vi "Autonomous Independent.vi"   [LabVIEW 2015]
doc: "This VI is called when autonomous begins, and will automatically be terminated when autonomous ends. You can carry out timed or sensor driven robot movement independently without needing to return to the caller."
uses:
  Robot Global Data.vi
  <vilib>/addons/control/pid/pid.llb/PID (DBL).vi
  navX Library v2/navX Library v2.lvlib
  <vilib>/addons/control/pid/NI_PID_pid.lvlib
panel:
  # "1 - Low Bar (Far Left)\n5 - Far Right"
  # "0 - Porticullis\n1 - Shovel the Fries\n2 - Low Bar\n3 - Rock Wall\n4 - Rough Terrain\n5\n6\n7"
types:
  T1 = typedef "navX Library v2.lvlib/Z900_navX_DeviceTypeDef.ctl" = cluster{"Interface":cluster{"Protocol":T2, "Update Rate (4Hz-60Hz)":u8, "navX Open TypeDef":variant}, "Notify Packet":refnum<notifier>, "Loop VI Refnum":refnum<vi>, "Ready to Close Occurrence Refnum":refnum<k4>}
  T2 = typedef "navX Library v2.lvlib/Z900_navX_ProtocolTypeDef.ctl" = enum16{"SERIAL", "I2C", "SPI"}
  T3 = typedef "WPI_EncoderDevRef.ctl" = cluster{"DevStatus":errorcluster, "EncoderIndex":T4, "CounterIndex":T5, "DistancePerCount":dbl, "Decoding Type":T6}
  T4 = typedef "FPGA_EncoderIdx.ctl" = enum8{"Enc 0", "Enc 1", "Enc 2", "Enc 3", "Enc 4", "Enc 5", "Enc 6", "Enc 7", "Invalid"}
  T5 = typedef "FPGA_CounterCtrSystemIndex.ctl" = enum8{"Ctr 0", "Ctr 1", "Ctr 2", "Ctr 3", "Ctr 4", "Ctr 5", "Ctr 6", "Ctr 7", "Invalid"}
  T6 = typedef "WPI_EncoderType.ctl" = enum16{"1x", "2x", "4x"}
  T7 = cluster{"proportional gain (Kc)":dbl, "integral time (Ti, min)":dbl, "derivative time (Td, min)":dbl}
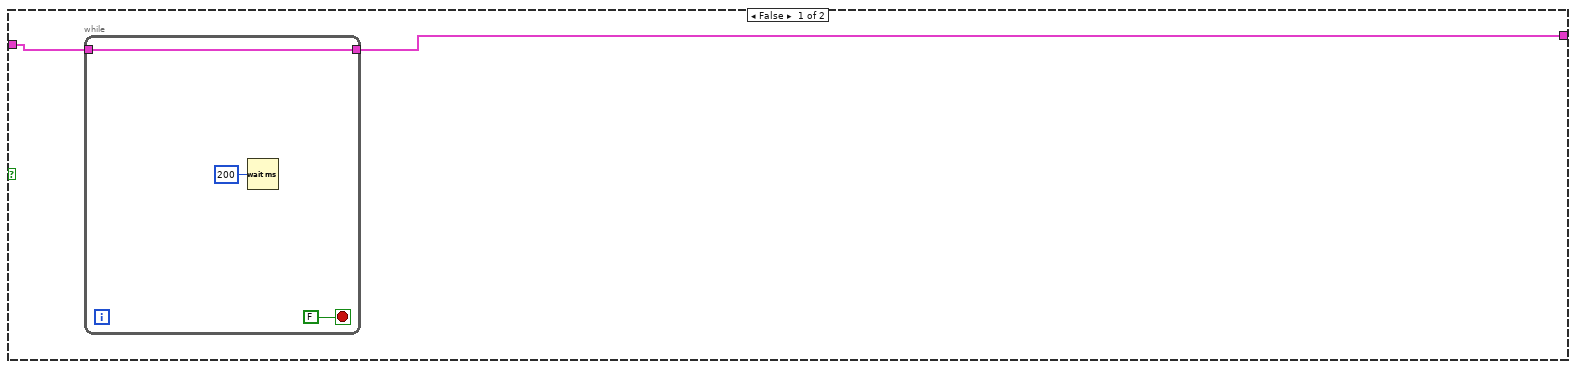
[diagram p2: hidden frame]
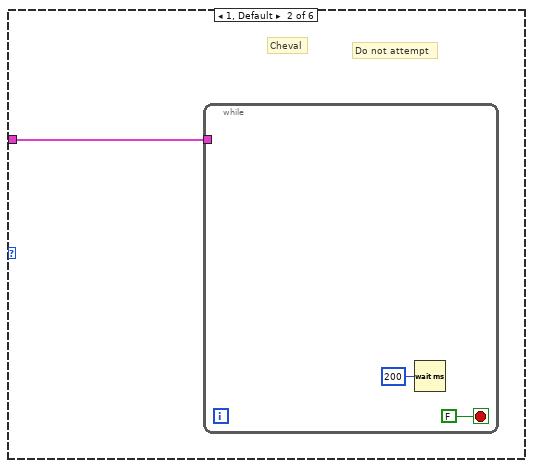
[diagram p3: hidden frame]
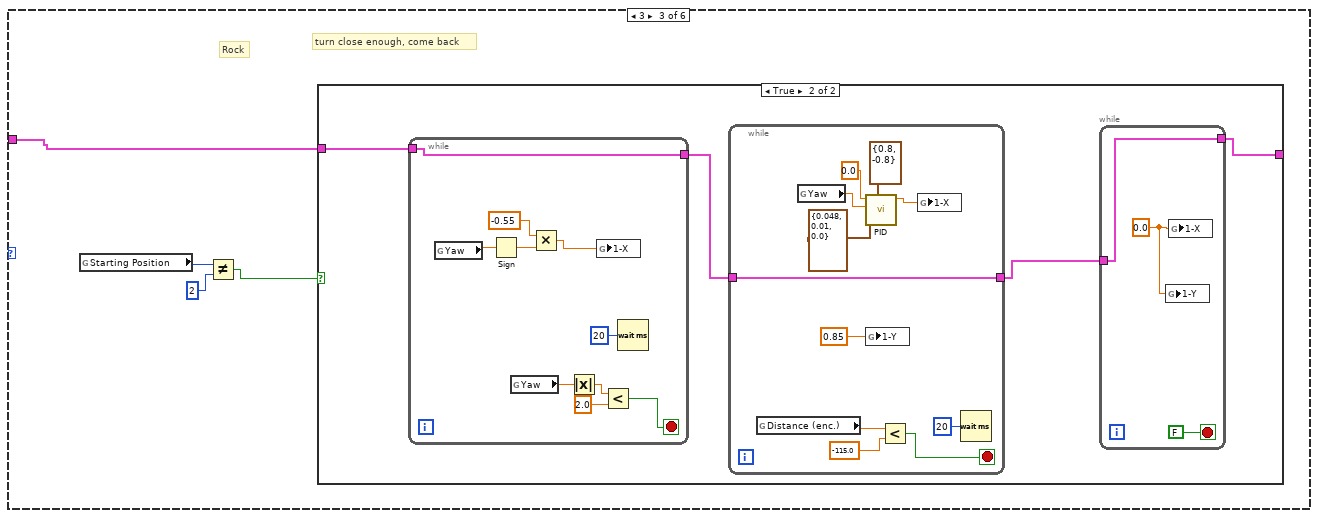
[diagram p4: hidden frame]
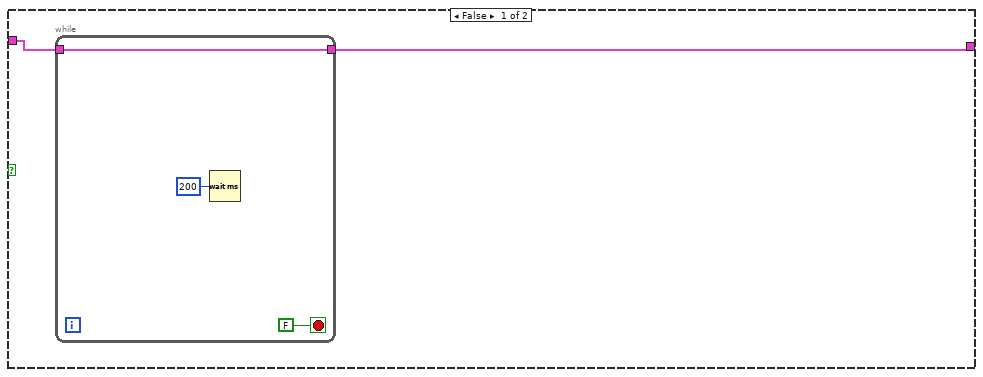
[diagram p5: hidden frame]
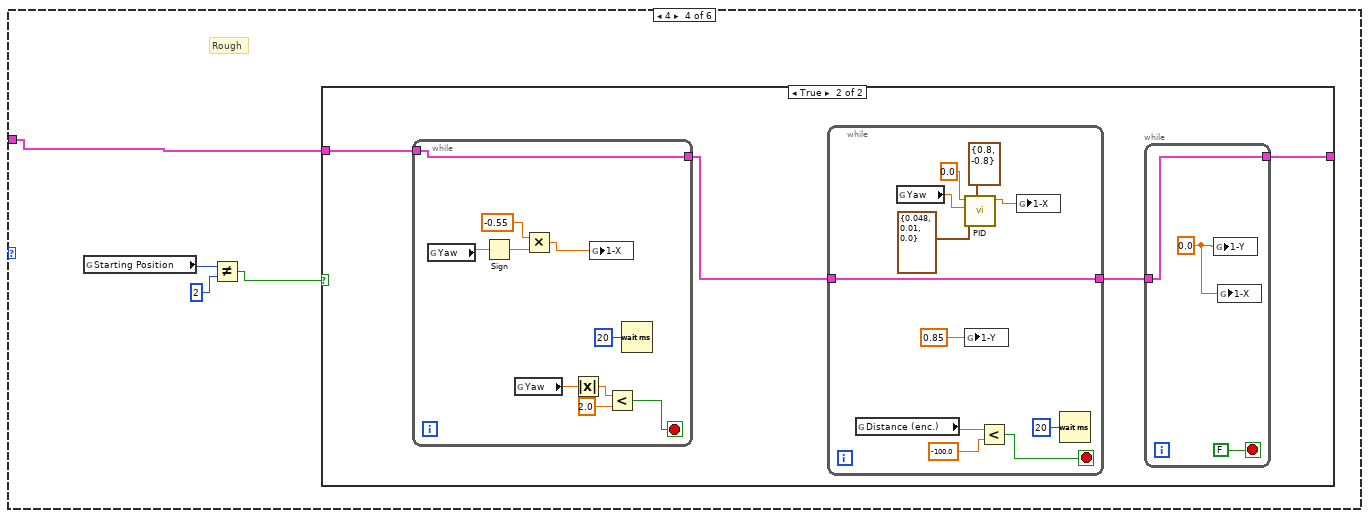
[diagram p6: hidden frame]
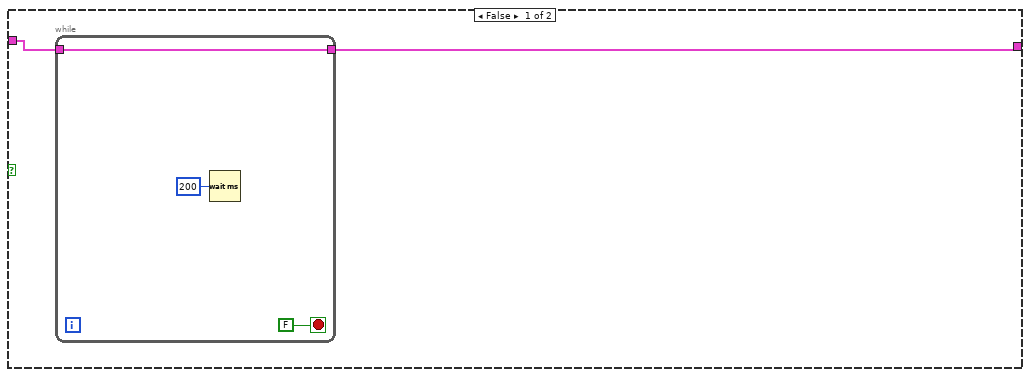
[diagram p7: hidden frame]
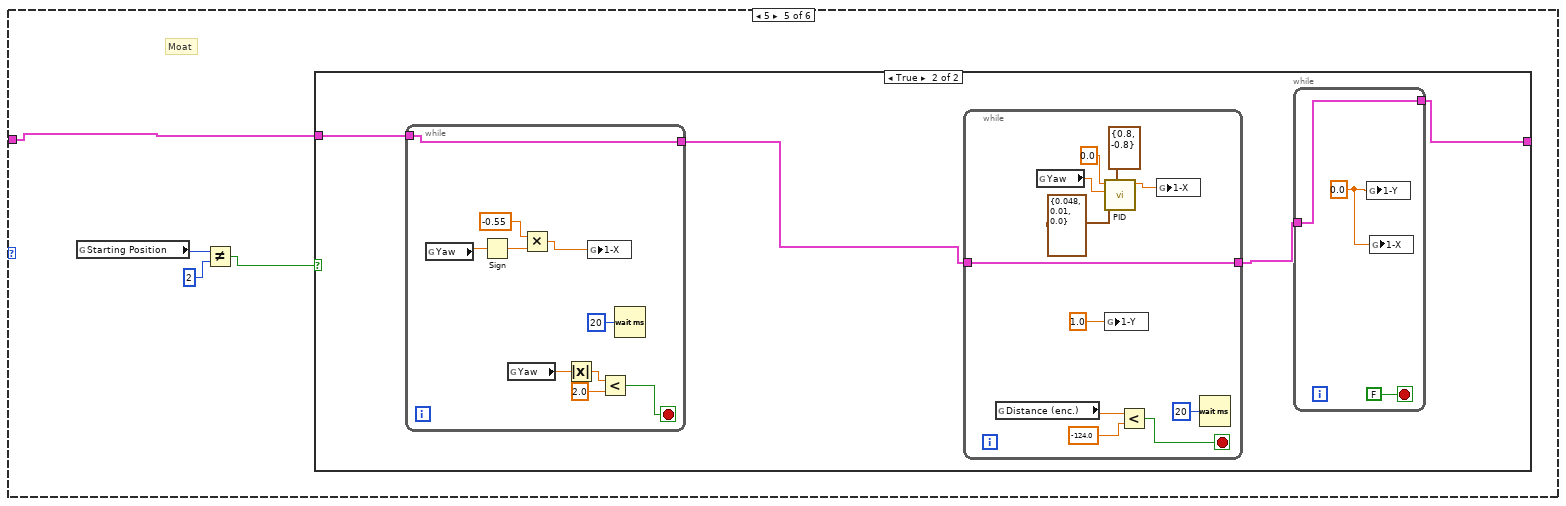
[diagram p8: hidden frame]
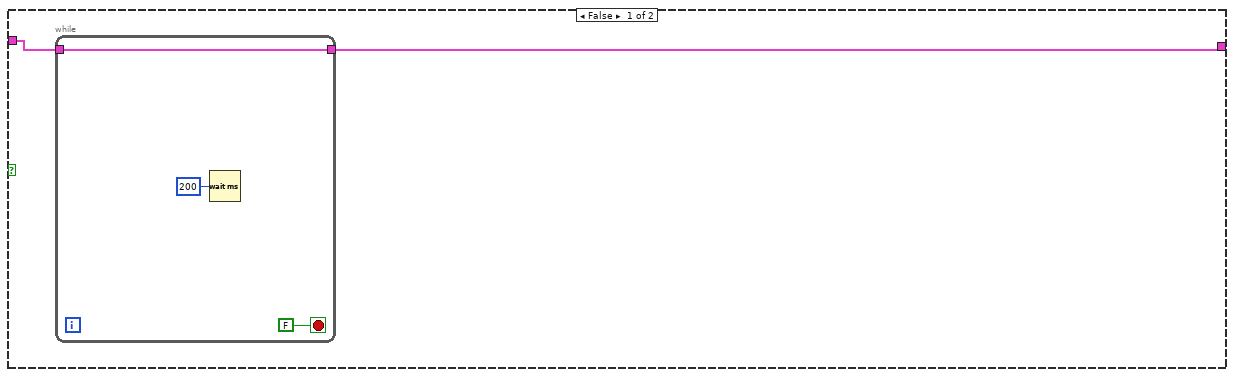
[diagram p9: hidden frame]
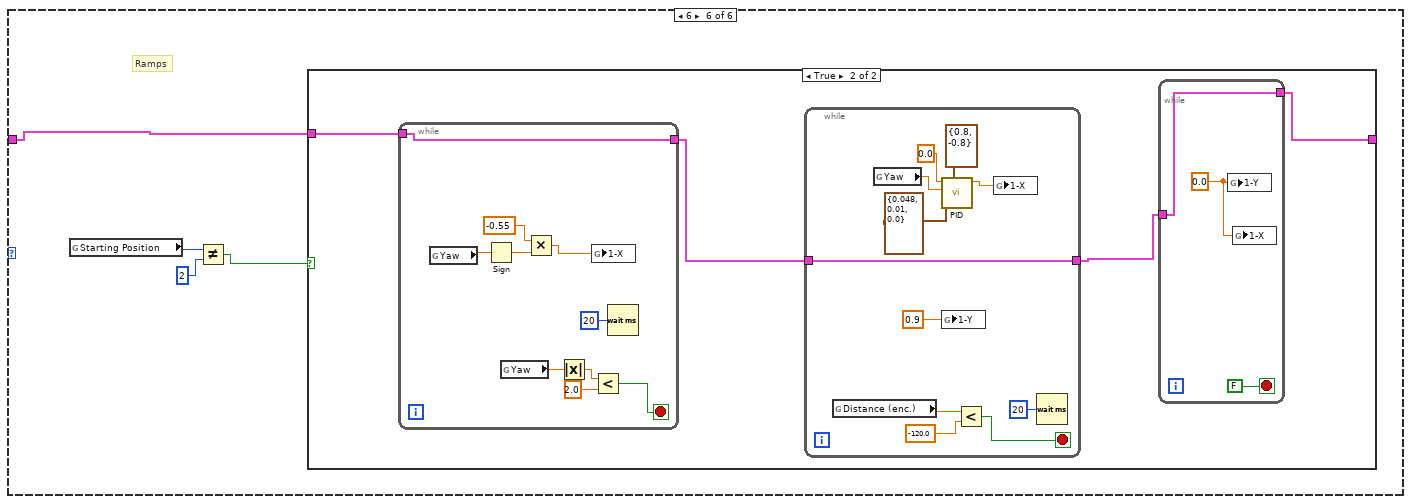
[diagram p10: hidden frame]
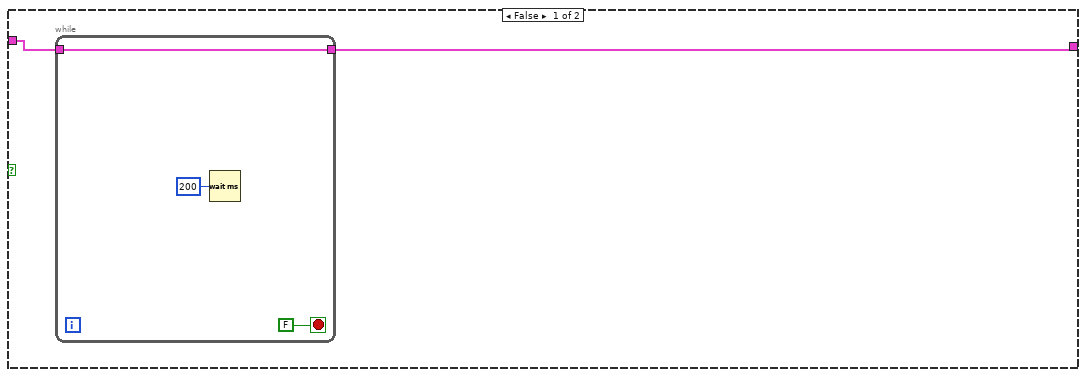
[diagram p11: hidden frame]
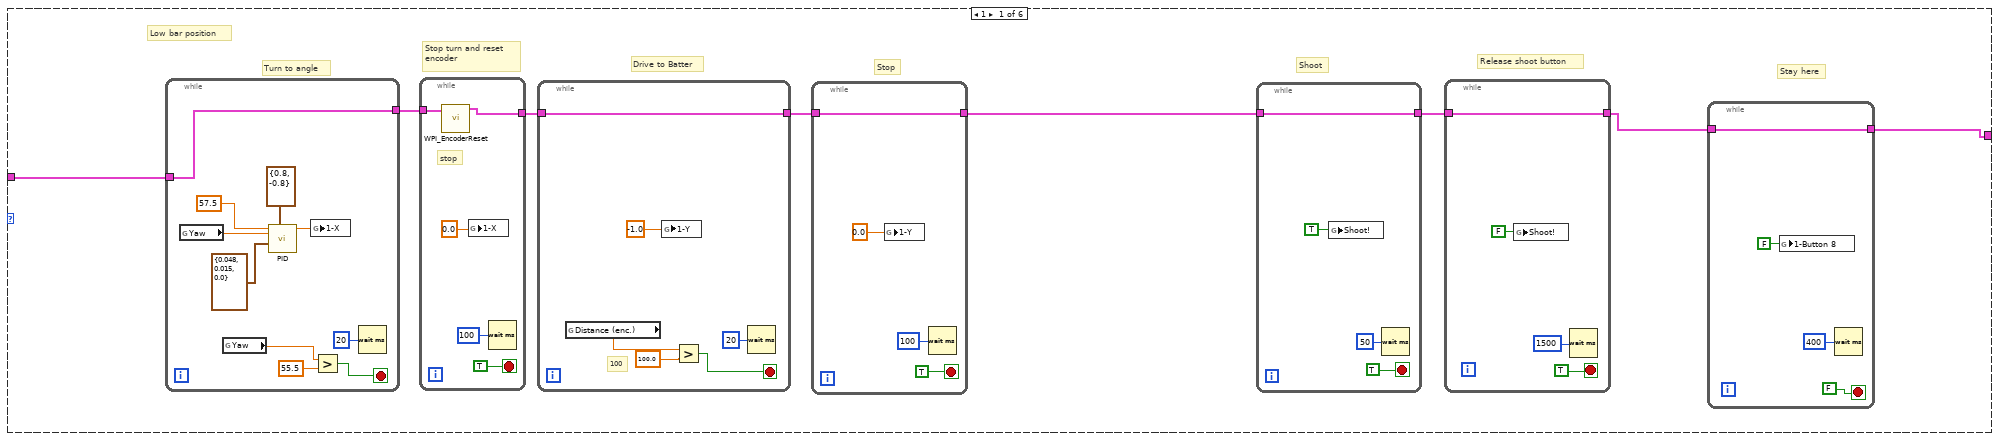
[diagram p12: hidden frame]
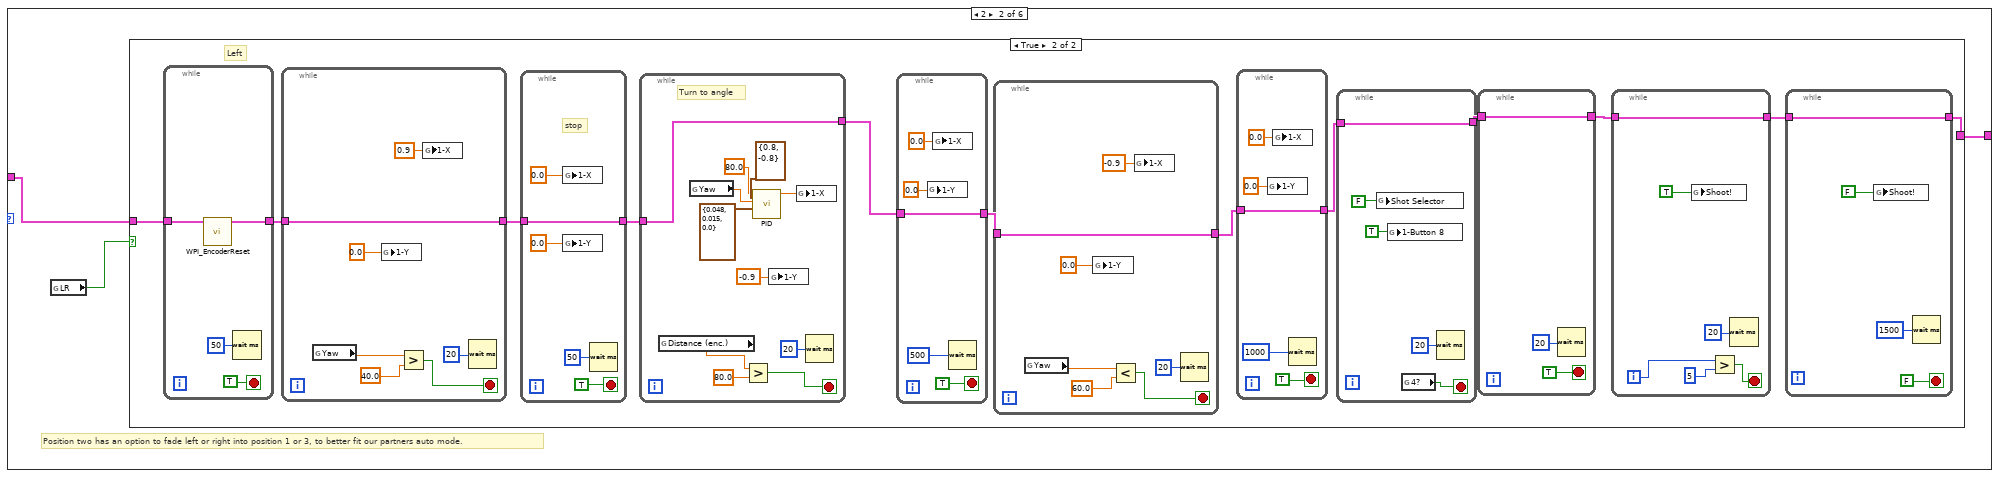
[diagram p13: hidden frame]
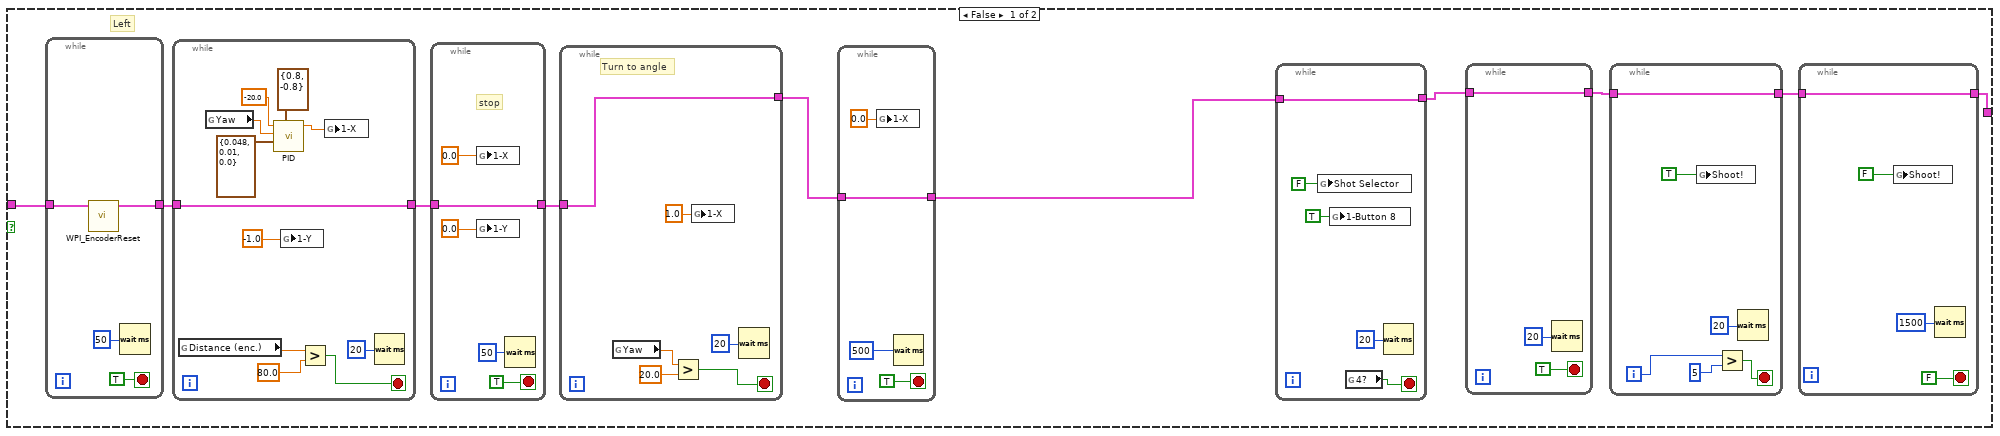
[diagram p14: hidden frame]
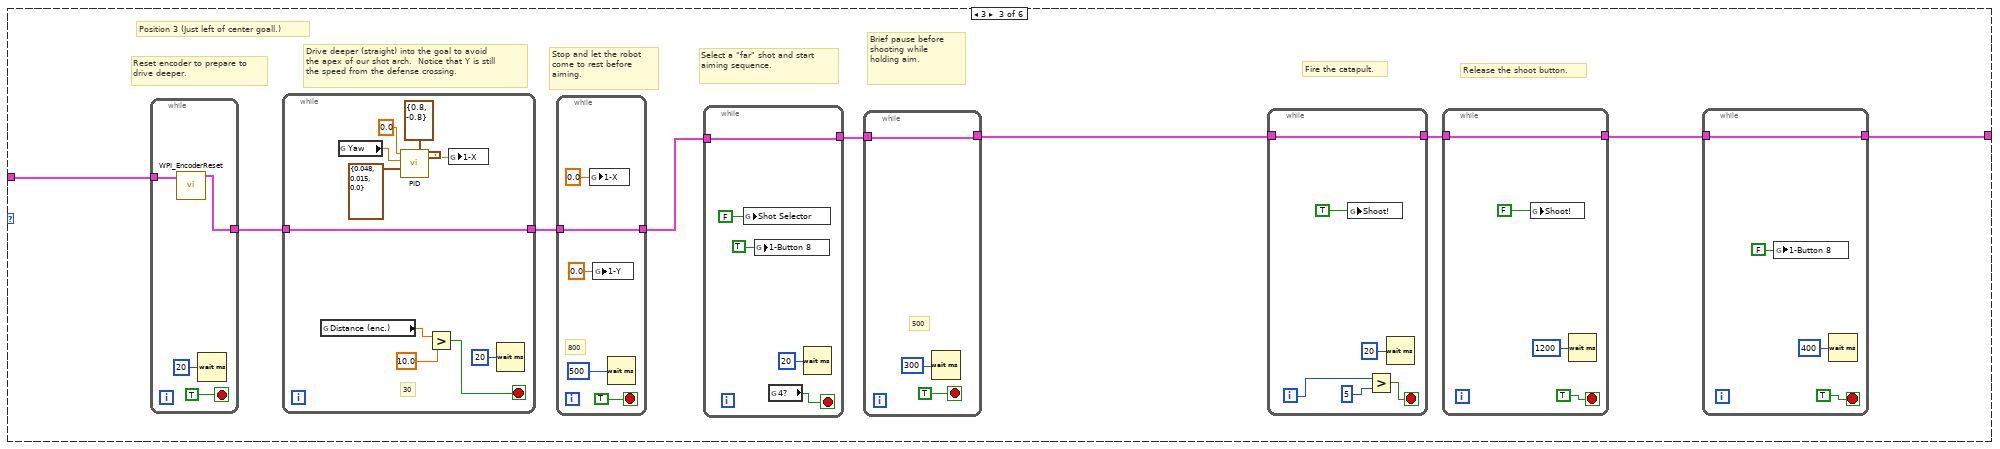
[diagram p15: hidden frame]
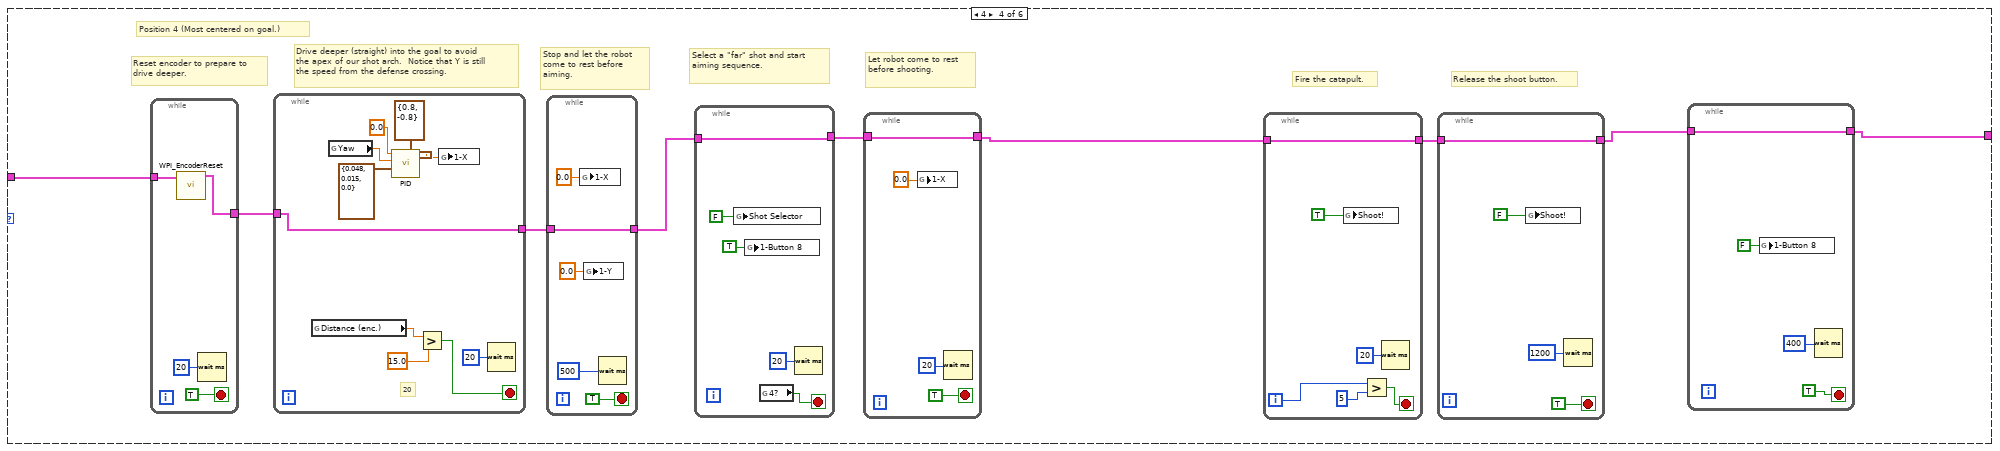
[diagram p16: hidden frame]
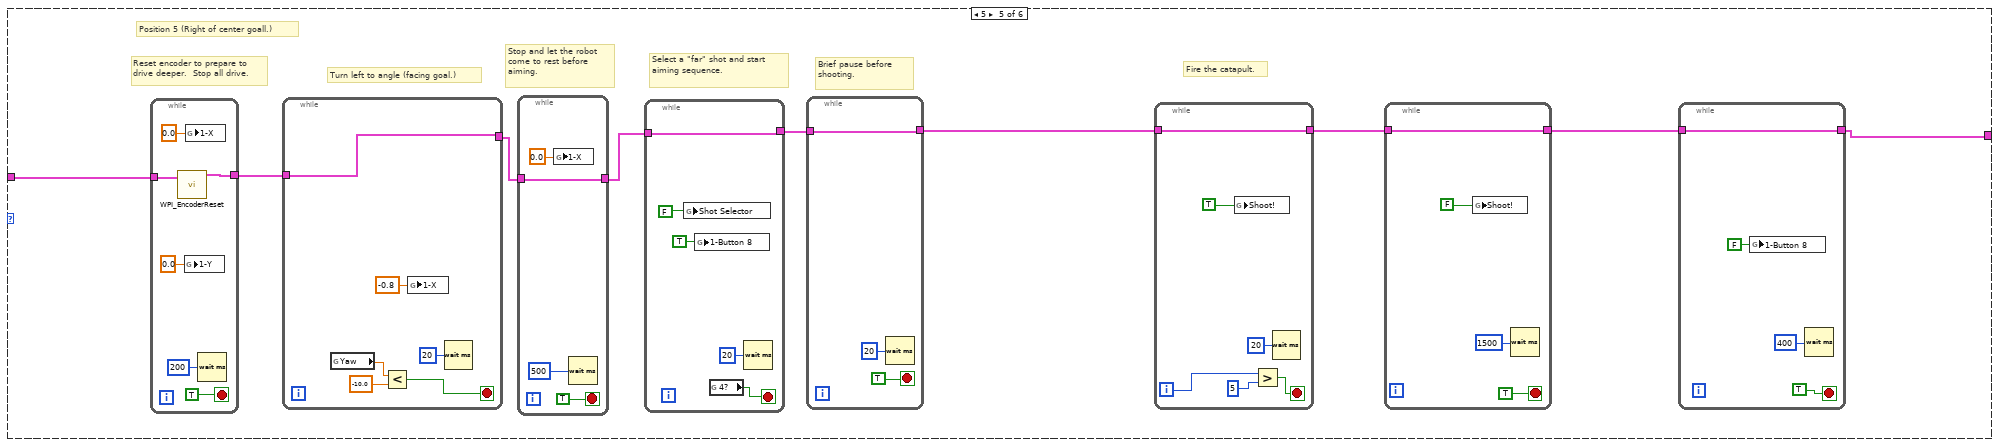
[diagram p17: hidden frame]
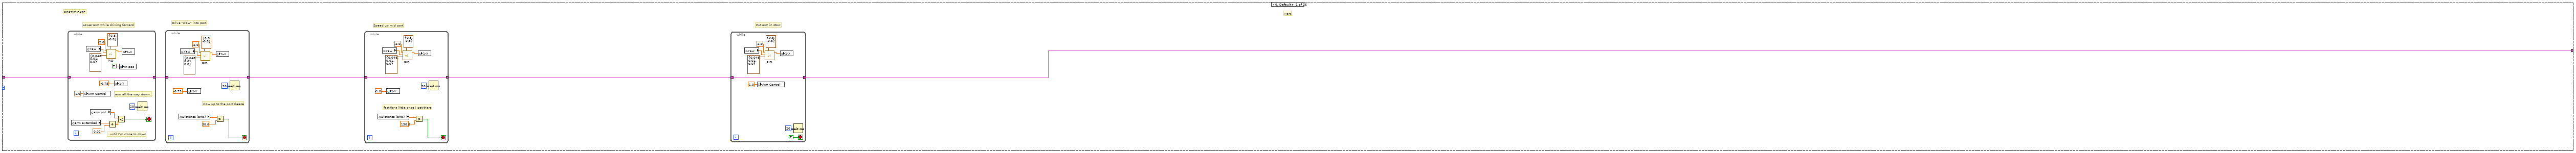
[diagram p18: hidden frame]
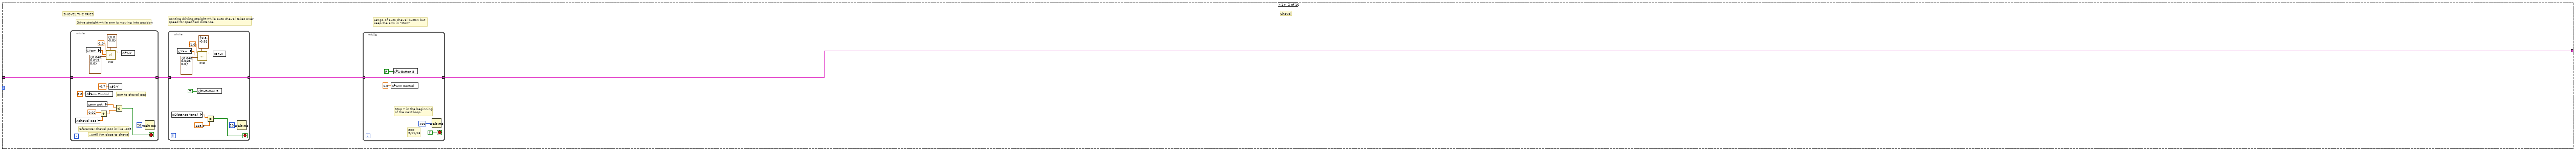
[diagram p19: hidden frame]
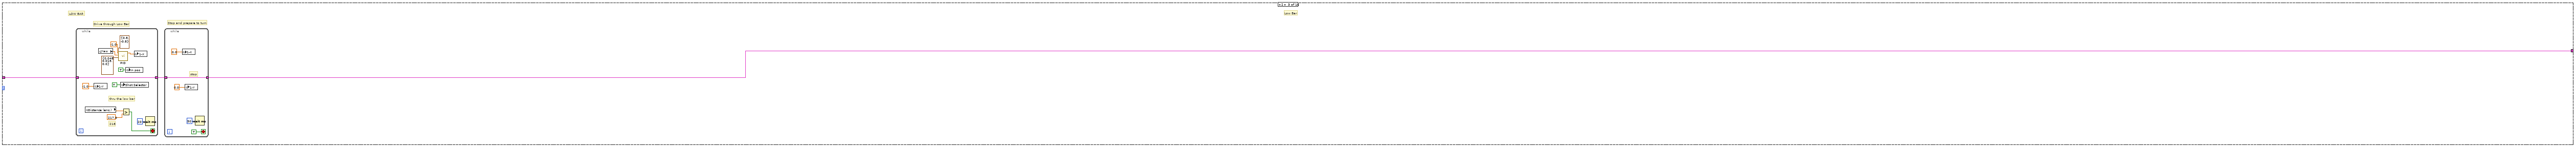
[diagram p20: hidden frame]
diagram:
  # "Our auto philosophy is to write the driver inputs to global variables, and the code for both modes is in periodic tasks"
  # "If the defense is not Cheval\nand the position is not 2\n(bc of wierd fade in 2),\nreturn to the neutral zone"
  # "GUIDE TO THESE AUTOS:\nThree loops are present. \nThe first is generally the \"cross defense\" loop, with the selector being which defense is to be crossed\nThe second is \"shoot the ball\".  The selector is what position - defense pos 5 and 2 in particular are different from the rest.\nThe third is \"return to neutral zone\". Specific to each defense\n\nTwo ball is entirely in the first loop"
  # "Last year we once had a problem.\nWe saved as default a hard left turn on the\njoystick. When we started auto we crashed into\nthe wall. We went overboard to make sure that's\nfixed this year. Reset EVERYTHING"
  # "Forces low bar to be low bar!"
  # "Every 20ms, report that we are running autonomous\ncode. Loop will abort the same time as the VI."
  # "This tells you the driver position\nand alliance color"
  n1 = while {
    stop <- FALSE stop-if-true
    n2 = call <vilib>:"WPI_DriverStationReport Robot Code State.vi"("Autonomous"=TRUE) -> ()  [unwired: 10 in, 1 out]
    n3 = Wait (ms)(milliseconds to wait=u32 20) -> ()  [unwired: 1 out]
  }
  n4 = call <vilib>:"WPI_DriverStationGet Alliance Info.vi"() -> ()  [unwired: 12 out]
  n5 = call "Z900_navX_RefNum_Get.vi"("refnum name"="NavX") -> ("navX Device"=w1:T1)  [unwired: 9 in, 1 out]
  n6 = call <vilib>:"WPI_EncoderRefNum Registry Get.vi"("refnum name"="encoder") -> ("EncoderDevRef"=w15:T3)  [unwired: 9 in, 1 out]
  n7 = while {
    tunnel: w15 -> [w40]
    tunnel: [w39] -> w13
    tunnel: w1 -> [w24]
    stop <- TRUE stop-if-true
    # "500"
    n8 = global read "Robot Global Data.vi" "CamTargetMem"() -> (w19:dbl)
    n9 = global write "Robot Global Data.vi" "In pos"(FALSE ("In pos")) -> ()
    n10 = global write "Robot Global Data.vi" "arm override"(FALSE ("In pos")) -> ()
    n11 = global write "Robot Global Data.vi" "1-X"(0.0 ("1-X")) -> ()
    n12 = global write "Robot Global Data.vi" "1-Y"(0.0 ("1-X")) -> ()
    n13 = call "Z900_navX_Set_ZeroYaw.vi"("navX Device"=w24) -> ()  [unwired: 9 in, 2 out]
    n14 = global write "Robot Global Data.vi" "1-Trigger"(FALSE ("In pos")) -> ()
    n15 = global write "Robot Global Data.vi" "retainer num"(i16 2 ("retainer num")) -> ()
    n16 = global write "Robot Global Data.vi" "in ctl num"(i16 0 ("retainer num")) -> ()
    n17 = global write "Robot Global Data.vi" "Shoot!"(FALSE ("In pos")) -> ()
    n18 = global write "Robot Global Data.vi" "Shot Selector"(FALSE ("In pos")) -> ()
    n19 = global write "Robot Global Data.vi" "Arm Control"(1.0 ("retainer num")) -> ()
    n20 = global write "Robot Global Data.vi" "climb num"(0 ("retainer num")) -> ()
    n21 = global write "Robot Global Data.vi" "left num"(i8 0 ("retainer num")) -> ()
    n22 = global write "Robot Global Data.vi" "right num"(i8 0 ("retainer num")) -> ()
    n23 = global write "Robot Global Data.vi" "1-Button 5"(FALSE ("In pos")) -> ()
    n24 = global write "Robot Global Data.vi" "1-TopLeft"(FALSE ("In pos")) -> ()
    n25 = call <vilib>:"WPI_EncoderReset.vi"("EncoderDevRef"=w40) -> ("EncoderDevRef"=w39:T3)  [unwired: 9 in, 1 out]
    n26 = global write "Robot Global Data.vi" "Pins / Intake timing"(550.0 ("Pins / Intake timing")) -> ()
    n27 = global write "Robot Global Data.vi" "CamTargetReal"(w19) -> ()
    n28 = global write "Robot Global Data.vi" "Slew"(0.2 ("PTO speed")) -> ()
    n29 = Wait (ms)(milliseconds to wait=u32 50) -> ()  [unwired: 1 out]
  }
  n30 = global read "Robot Global Data.vi" "Defense to Cross"() -> (w12:i32)
  n31 = case shown="8" w12 {
    tunnel: w13 -> [w46 w96 w129 w149 w162 w175 w188 w212 w311 w604 w625 w823 w1043 w1309 w1568 w1848]
    tunnel: [w42 w93 w128 w148 w161 w174 w187 w200 w313 w603 w627 w825 w1045 w1311 w1570 w1850] -> w3
    frame 0, Default {
      # "Port"
      # "Put arm in stow"
      # "Speed up mid port"
      # "Drive \"slow\" into port."
      # "Lower arm while driving forward"
      # "PORTICLEASE"
      n32 = while {
        tunnel: w46 -> [w86]
        tunnel: [w86] -> w45
        stop <- w87 stop-if-true
        # "..until I'm close to down"
        # "arm all the way down..."
        n33 = global read "Robot Global Data.vi" "arm extended"() -> (w89:dbl)
        n34 = global write "Robot Global Data.vi" "Arm Control"(-1.0 ("retainer num")) -> ()
        n35 = global read "Robot Global Data.vi" "Yaw"() -> (w79:dbl)
        n36 = global read "Robot Global Data.vi" "arm pot"() -> (w91:dbl)
        n37 = call-poly <vilib>:"PID.vi"("output range"=cluster{"output high":dbl, "output low":dbl} {"output high"=0.8, "output low"=-0.8} ("output range 2"), "PID gains"=T7 {"proportional gain (Kc)"=0.048, "integral time (Ti, min)"=0.01, "derivative time (Td, min)"=0.0} ("PID gains 2"), "process variable"=w79, "setpoint"=-2.0) -> ("output"=w81:dbl)  [unwired: 6 in, 1 out]
        n38 = Add(x=w89, y=0.02) -> (x+y=w90:dbl)
        n39 = global write "Robot Global Data.vi" "1-Y"(-0.75 ("1-X")) -> ()
        n40 = Less?(x=w91, y=w90) -> (x < y?=w87:bool)
        n41 = global write "Robot Global Data.vi" "In pos"(TRUE ("In pos")) -> ()
        n42 = global write "Robot Global Data.vi" "1-X"(w81) -> ()
        n43 = Wait (ms)(milliseconds to wait=u32 20) -> ()  [unwired: 1 out]
      }
      n44 = while {
        tunnel: w45 -> [w72]
        tunnel: [w72] -> w44
        stop <- w74 stop-if-true
        # "slow up to the porticlease"
        n45 = global read "Robot Global Data.vi" "Distance (enc.)"() -> (w76:dbl)
        n46 = global read "Robot Global Data.vi" "Yaw"() -> (w67:dbl)
        n47 = global write "Robot Global Data.vi" "1-Y"(-0.75 ("1-X")) -> ()
        n48 = call-poly <vilib>:"PID.vi"("output range"=cluster{"output high":dbl, "output low":dbl} {"output high"=0.8, "output low"=-0.8} ("output range 2"), "PID gains"=T7 {"proportional gain (Kc)"=0.048, "integral time (Ti, min)"=0.01, "derivative time (Td, min)"=0.0} ("PID gains 2"), "process variable"=w67, "setpoint"=-2.0) -> ("output"=w69:dbl)  [unwired: 6 in, 1 out]
        n49 = Greater?(x=w76, y=50.0) -> (0:w74:bool)
        n50 = global write "Robot Global Data.vi" "1-X"(w69) -> ()
        n51 = Wait (ms)(milliseconds to wait=u32 20) -> ()  [unwired: 1 out]
      }
      n52 = while {
        tunnel: w44 -> [w61]
        tunnel: [w61] -> w43
        stop <- w63 stop-if-true
        # "fast for a little once i get there"
        n53 = global read "Robot Global Data.vi" "Distance (enc.)"() -> (w65:dbl)
        n54 = global read "Robot Global Data.vi" "Yaw"() -> (w56:dbl)
        n55 = global write "Robot Global Data.vi" "1-Y"(-1.0 ("1-X")) -> ()
        n56 = call-poly <vilib>:"PID.vi"("output range"=cluster{"output high":dbl, "output low":dbl} {"output high"=0.8, "output low"=-0.8} ("output range 2"), "PID gains"=T7 {"proportional gain (Kc)"=0.048, "integral time (Ti, min)"=0.01, "derivative time (Td, min)"=0.0} ("PID gains 2"), "process variable"=w56, "setpoint"=-2.0) -> ("output"=w58:dbl)  [unwired: 6 in, 1 out]
        n57 = Greater?(x=w65, y=130.0) -> (0:w63:bool)
        n58 = global write "Robot Global Data.vi" "1-X"(w58) -> ()
        n59 = Wait (ms)(milliseconds to wait=u32 20) -> ()  [unwired: 1 out]
      }
      n60 = while {
        tunnel: w43 -> [w54]
        tunnel: [w54] -> w42
        stop <- TRUE stop-if-true
        n61 = global read "Robot Global Data.vi" "Yaw"() -> (w47:dbl)
        n62 = global write "Robot Global Data.vi" "Arm Control"(-1.0 ("retainer num")) -> ()
        n63 = call-poly <vilib>:"PID.vi"("output range"=cluster{"output high":dbl, "output low":dbl} {"output high"=0.8, "output low"=-0.8} ("output range 2"), "PID gains"=T7 {"proportional gain (Kc)"=0.048, "integral time (Ti, min)"=0.01, "derivative time (Td, min)"=0.0} ("PID gains 2"), "process variable"=w47, "setpoint"=-2.0) -> ("output"=w49:dbl)  [unwired: 6 in, 1 out]
        n64 = global write "Robot Global Data.vi" "1-X"(w49) -> ()
        n65 = Wait (ms)(milliseconds to wait=u32 20) -> ()  [unwired: 1 out]
      }
    }
    frame 1 {
      # "Cheval"
      # "Let go of auto cheval button but keep the arm in \"stow\""
      # "Contine driving straight while auto cheval takes over speed for specified distance."
      # "Drive straight while arm is moving into position"
      # "SHOVEL THE FRIES"
      n66 = while {
        tunnel: w96 -> [w125]
        tunnel: [w125] -> w95
        stop <- w119 stop-if-true
        # "reference: cheval pos is like .425"
        # "..until I'm close to cheval"
        # "arm to cheval pos"
        n67 = global read "Robot Global Data.vi" "cheval pos"() -> (w120:dbl)
        n68 = global write "Robot Global Data.vi" "Arm Control"(0.0 ("retainer num")) -> ()
        n69 = global read "Robot Global Data.vi" "Yaw"() -> (w114:dbl)
        n70 = global read "Robot Global Data.vi" "arm pot"() -> (w123:dbl)
        n71 = Add(x=0.02, y=w120) -> (x+y=w122:dbl)
        n72 = call-poly <vilib>:"PID.vi"("output range"=cluster{"output high":dbl, "output low":dbl} {"output high"=0.8, "output low"=-0.8} ("output range 2"), "PID gains"=T7 {"proportional gain (Kc)"=0.048, "integral time (Ti, min)"=0.015, "derivative time (Td, min)"=0.0} ("PID gains 2"), "process variable"=w114, "setpoint"=-1.0) -> ("output"=w116:dbl)  [unwired: 6 in, 1 out]
        n73 = global write "Robot Global Data.vi" "1-Y"(-0.7 ("1-Y")) -> ()
        n74 = Less?(x=w123, y=w122) -> (x < y?=w119:bool)
        n75 = global write "Robot Global Data.vi" "1-X"(w116) -> ()
        n76 = Wait (ms)(milliseconds to wait=u32 20) -> ()  [unwired: 1 out]
      }
      n77 = while {
        tunnel: w95 -> [w111]
        tunnel: [w111] -> w94
        stop <- w107 stop-if-true
        n78 = global read "Robot Global Data.vi" "Distance (enc.)"() -> (w109:dbl)
        n79 = global read "Robot Global Data.vi" "Yaw"() -> (w102:dbl)
        n80 = global write "Robot Global Data.vi" "1-Button 5"(TRUE ("In pos")) -> ()
        n81 = call-poly <vilib>:"PID.vi"("output range"=cluster{"output high":dbl, "output low":dbl} {"output high"=0.8, "output low"=-0.8} ("output range 2"), "PID gains"=T7 {"proportional gain (Kc)"=0.048, "integral time (Ti, min)"=0.015, "derivative time (Td, min)"=0.0} ("PID gains 2"), "process variable"=w102, "setpoint"=-1.0) -> ("output"=w104:dbl)  [unwired: 6 in, 1 out]
        n82 = Greater?(x=w109, y=125.0) -> (0:w107:bool)
        n83 = global write "Robot Global Data.vi" "1-X"(w104) -> ()
        n84 = Wait (ms)(milliseconds to wait=u32 20) -> ()  [unwired: 1 out]
      }
      n85 = while {
        tunnel: w94 -> [w100]
        tunnel: [w100] -> w93
        stop <- TRUE stop-if-true
        # "800\n3/11/16"
        # "Stop Y in the beginning\nof the next loop."
        n86 = global write "Robot Global Data.vi" "Arm Control"(1.0 ("retainer num")) -> ()
        n87 = global write "Robot Global Data.vi" "1-Button 5"(FALSE ("In pos")) -> ()
        n88 = Wait (ms)(milliseconds to wait=u32 400) -> ()  [unwired: 1 out]
      }
    }
    frame 2 {
      # "Low Bar"
      # "Stop and prepare to turn"
      # "Drive through Low Bar"
      # "LOW BAR"
      n89 = while {
        tunnel: w129 -> [w146]
        tunnel: [w146] -> w127
        stop <- w142 stop-if-true
        # "218"
        # "thru the low bar"
        n90 = global read "Robot Global Data.vi" "Distance (enc.)"() -> (w144:dbl)
        n91 = global write "Robot Global Data.vi" "1-Y"(-1.0 ("1-X")) -> ()
        n92 = global read "Robot Global Data.vi" "Yaw"() -> (w137:dbl)
        n93 = call-poly <vilib>:"PID.vi"("output range"=cluster{"output high":dbl, "output low":dbl} {"output high"=0.8, "output low"=-0.8} ("output range 2"), "PID gains"=T7 {"proportional gain (Kc)"=0.048, "integral time (Ti, min)"=0.015, "derivative time (Td, min)"=0.0} ("PID gains 2"), "process variable"=w137, "setpoint"=-1.0) -> ("output"=w139:dbl)  [unwired: 6 in, 1 out]
        n94 = global write "Robot Global Data.vi" "Shot Selector"(TRUE ("In pos")) -> ()
        n95 = Greater?(x=w144, y=217.0) -> (0:w142:bool)
        n96 = global write "Robot Global Data.vi" "In pos"(TRUE ("In pos")) -> ()
        n97 = global write "Robot Global Data.vi" "1-X"(w139) -> ()
        n98 = Wait (ms)(milliseconds to wait=u32 20) -> ()  [unwired: 1 out]
      }
      n99 = while {
        tunnel: w127 -> [w133]
        tunnel: [w133] -> w128
        stop <- TRUE stop-if-true
        # "stop"
        n100 = global write "Robot Global Data.vi" "1-X"(0.0 ("1-X")) -> ()
        n101 = global write "Robot Global Data.vi" "1-Y"(0.0 ("1-X")) -> ()
        n102 = Wait (ms)(milliseconds to wait=u32 50) -> ()  [unwired: 1 out]
      }
    }
    frame 3 {
      # "Rock"
      # "Drive straight at speed for distance"
      # "Rock Wall"
      n103 = while {
        tunnel: w149 -> [w159]
        tunnel: [w159] -> w148
        stop <- w155 stop-if-true
        n104 = global read "Robot Global Data.vi" "Distance (enc.)"() -> (w157:dbl)
        n105 = global read "Robot Global Data.vi" "Yaw"() -> (w150:dbl)
        n106 = global write "Robot Global Data.vi" "1-Y"(-0.85 ("1-X")) -> ()
        n107 = call-poly <vilib>:"PID.vi"("output range"=cluster{"output high":dbl, "output low":dbl} {"output high"=0.8, "output low"=-0.8} ("output range 2"), "PID gains"=T7 {"proportional gain (Kc)"=0.048, "integral time (Ti, min)"=0.01, "derivative time (Td, min)"=0.0} ("PID gains 2"), "process variable"=w150, "setpoint"=-1.0) -> ("output"=w152:dbl)  [unwired: 6 in, 1 out]
        n108 = Greater?(x=w157, y=145.0) -> (0:w155:bool)
        n109 = global write "Robot Global Data.vi" "1-X"(w152) -> ()
        n110 = Wait (ms)(milliseconds to wait=u32 20) -> ()  [unwired: 1 out]
      }
    }
    frame 4 {
      # "Rough"
      # "Drive straight at speed for distance"
      # "Rough Terrain"
      n111 = while {
        tunnel: w162 -> [w172]
        tunnel: [w172] -> w161
        stop <- w168 stop-if-true
        n112 = global read "Robot Global Data.vi" "Distance (enc.)"() -> (w170:dbl)
        n113 = global read "Robot Global Data.vi" "Yaw"() -> (w163:dbl)
        n114 = call-poly <vilib>:"PID.vi"("output range"=cluster{"output high":dbl, "output low":dbl} {"output high"=0.8, "output low"=-0.8} ("output range 2"), "PID gains"=T7 {"proportional gain (Kc)"=0.048, "integral time (Ti, min)"=0.008, "derivative time (Td, min)"=0.0} ("PID gains 2"), "process variable"=w163, "setpoint"=-1.0) -> ("output"=w165:dbl)  [unwired: 6 in, 1 out]
        n115 = global write "Robot Global Data.vi" "1-Y"(-0.9 ("1-X")) -> ()
        n116 = Greater?(x=w170, y=135.0) -> (0:w168:bool)
        n117 = global write "Robot Global Data.vi" "1-X"(w165) -> ()
        n118 = Wait (ms)(milliseconds to wait=u32 20) -> ()  [unwired: 1 out]
      }
    }
    frame 5 {
      # "Moat"
      # "Drive straight at speed for distance"
      # "Moat !!!!!"
      n119 = while {
        tunnel: w175 -> [w185]
        tunnel: [w185] -> w174
        stop <- w181 stop-if-true
        n120 = global read "Robot Global Data.vi" "Distance (enc.)"() -> (w183:dbl)
        n121 = global read "Robot Global Data.vi" "Yaw"() -> (w176:dbl)
        n122 = call-poly <vilib>:"PID.vi"("output range"=cluster{"output high":dbl, "output low":dbl} {"output high"=0.8, "output low"=-0.8} ("output range 2"), "PID gains"=T7 {"proportional gain (Kc)"=0.048, "integral time (Ti, min)"=0.01, "derivative time (Td, min)"=0.0} ("PID gains 2"), "process variable"=w176, "setpoint"=-1.0) -> ("output"=w178:dbl)  [unwired: 6 in, 1 out]
        n123 = global write "Robot Global Data.vi" "1-Y"(-0.85 ("1-X")) -> ()
        n124 = Greater?(x=w183, y=150.0) -> (0:w181:bool)
        n125 = global write "Robot Global Data.vi" "1-X"(w178) -> ()
        n126 = Wait (ms)(milliseconds to wait=u32 20) -> ()  [unwired: 1 out]
      }
    }
    frame 6 {
      # "Ramps"
      # "Drive straight at speed for distance"
      # "Ramparts !!!!!"
      n127 = while {
        tunnel: w188 -> [w198]
        tunnel: [w198] -> w187
        stop <- w194 stop-if-true
        n128 = global read "Robot Global Data.vi" "Distance (enc.)"() -> (w196:dbl)
        n129 = global read "Robot Global Data.vi" "Yaw"() -> (w189:dbl)
        n130 = call-poly <vilib>:"PID.vi"("output range"=cluster{"output high":dbl, "output low":dbl} {"output high"=0.8, "output low"=-0.8} ("output range 2"), "PID gains"=T7 {"proportional gain (Kc)"=0.048, "integral time (Ti, min)"=0.01, "derivative time (Td, min)"=0.0} ("PID gains 2"), "process variable"=w189, "setpoint"=-1.0) -> ("output"=w191:dbl)  [unwired: 6 in, 1 out]
        n131 = global write "Robot Global Data.vi" "1-Y"(-0.9 ("1-X")) -> ()
        n132 = Greater?(x=w196, y=140.0) -> (0:w194:bool)
        n133 = global write "Robot Global Data.vi" "1-X"(w191) -> ()
        n134 = Wait (ms)(milliseconds to wait=u32 20) -> ()  [unwired: 1 out]
      }
    }
    frame 7 {
      # "Low bar, far shot with vision and return to neutral zone. Contained fully in this loop, since pos 1 was already used for no vision batter shot low bar"
      # "Stop turn and reset encoder"
      # "Turn to angle"
      # "Low bar position"
      # "Stop and prepare to turn"
      # "Drive through Low Bar"
      # "LOW BAR"
      n135 = while {
        tunnel: w212 -> [w284]
        tunnel: [w284] -> w211
        stop <- w280 stop-if-true
        # "218"
        # "thru the low bar"
        n136 = global read "Robot Global Data.vi" "Distance (enc.)"() -> (w282:dbl)
        n137 = global write "Robot Global Data.vi" "1-Y"(-1.0 ("1-X")) -> ()
        n138 = global read "Robot Global Data.vi" "Yaw"() -> (w275:dbl)
        n139 = call-poly <vilib>:"PID.vi"("output range"=cluster{"output high":dbl, "output low":dbl} {"output high"=0.8, "output low"=-0.8} ("output range 2"), "PID gains"=T7 {"proportional gain (Kc)"=0.048, "integral time (Ti, min)"=0.015, "derivative time (Td, min)"=0.0} ("PID gains 2"), "process variable"=w275, "setpoint"=-1.0) -> ("output"=w277:dbl)  [unwired: 6 in, 1 out]
        n140 = Greater?(x=w282, y=200.0) -> (0:w280:bool)
        n141 = global write "Robot Global Data.vi" "In pos"(TRUE ("In pos")) -> ()
        n142 = global write "Robot Global Data.vi" "1-X"(w277) -> ()
        n143 = Wait (ms)(milliseconds to wait=u32 20) -> ()  [unwired: 1 out]
      }
      n144 = while {
        tunnel: w211 -> [w272]
        tunnel: [w272] -> w209
        stop <- TRUE stop-if-true
        # "stop"
        n145 = global write "Robot Global Data.vi" "1-X"(0.0 ("1-X")) -> ()
        n146 = global write "Robot Global Data.vi" "1-Y"(0.0 ("1-X")) -> ()
        n147 = Wait (ms)(milliseconds to wait=u32 50) -> ()  [unwired: 1 out]
      }
      n148 = while {
        tunnel: [w265] -> w210
        tunnel: w209 -> [w265]
        stop <- w264 stop-if-true
        n149 = global read "Robot Global Data.vi" "Yaw"() -> (w267:dbl)
        n150 = global write "Robot Global Data.vi" "1-X"(0.8 ("1-X")) -> ()
        n151 = Greater?(x=w267, y=20.0) -> (0:w264:bool)
        n152 = Wait (ms)(milliseconds to wait=u32 20) -> ()  [unwired: 1 out]
      }
      n153 = while {
        tunnel: [w259] -> w206
        tunnel: w210 -> [w259]
        stop <- TRUE stop-if-true
        n154 = global write "Robot Global Data.vi" "1-X"(0.0 ("1-X")) -> ()
        n155 = Wait (ms)(milliseconds to wait=u32 500) -> ()  [unwired: 1 out]
      }
      n156 = while {
        tunnel: [w256] -> w205
        tunnel: w206 -> [w256]
        stop <- w258 stop-if-true
        n157 = global write "Robot Global Data.vi" "Shot Selector"(FALSE ("In pos")) -> ()
        n158 = global write "Robot Global Data.vi" "1-Button 8"(TRUE ("1-Button 8")) -> ()
        n159 = global read "Robot Global Data.vi" "4?"() -> (w258:bool)
        n160 = Wait (ms)(milliseconds to wait=u32 20) -> ()  [unwired: 1 out]
      }
      n161 = while {
        tunnel: w205 -> [w242]
        tunnel: [w242] -> w207
        stop <- TRUE stop-if-true
        n162 = Wait (ms)(milliseconds to wait=u32 200) -> ()  [unwired: 1 out]
      }
      n163 = while {
        tunnel: [w253] -> w208
        tunnel: w207 -> [w253]
        i -> [w251]
        stop <- w249 stop-if-true
        n164 = global write "Robot Global Data.vi" "Shoot!"(TRUE ("1-Button 8")) -> ()
        n165 = Greater?(x=w251, y=5) -> (0:w249:bool)
        n166 = Wait (ms)(milliseconds to wait=u32 20) -> ()  [unwired: 1 out]
      }
      n167 = while {
        tunnel: [w247] -> w203
        tunnel: w208 -> [w247]
        stop <- TRUE stop-if-true
        n168 = global write "Robot Global Data.vi" "Shoot!"(FALSE ("1-Button 8")) -> ()
        n169 = Wait (ms)(milliseconds to wait=u32 1200) -> ()  [unwired: 1 out]
      }
      n170 = while {
        tunnel: w203 -> [w235]
        tunnel: [w235] -> w204
        stop <- w237 stop-if-true
        n171 = global read "Robot Global Data.vi" "Yaw"() -> (w234:dbl)
        n172 = global write "Robot Global Data.vi" "1-Button 8"(FALSE ("1-Button 8")) -> ()
        n173 = Sign(1:w234) -> (0:w233:dbl)
        n174 = global read "Robot Global Data.vi" "Yaw"() -> (w240:dbl)
        n175 = Multiply(x=-0.57, y=w233) -> (x*y=w231:dbl)
        n176 = Absolute Value(x=w240) -> (abs(x)=w239:dbl)
        n177 = Less?(x=w239, y=7.0) -> (x < y?=w237:bool)
        n178 = global write "Robot Global Data.vi" "1-X"(w231) -> ()
        n179 = Wait (ms)(milliseconds to wait=u32 20) -> ()  [unwired: 1 out]
      }
      n180 = while {
        tunnel: w204 -> [w229]
        tunnel: [w229] -> w202
        stop <- TRUE stop-if-true
        w227 = 0.0 ("1-X")
        n181 = Wait (ms)(milliseconds to wait=u32 20) -> ()  [unwired: 1 out]
        n182 = global write "Robot Global Data.vi" "1-X"(w227) -> ()
        n183 = global write "Robot Global Data.vi" "1-Y"(w227) -> ()
      }
      n184 = while {
        tunnel: w202 -> [w225]
        tunnel: [w225] -> w201
        stop <- w217 stop-if-true
        n185 = global read "Robot Global Data.vi" "Yaw"() -> (w220:dbl)
        n186 = global read "Robot Global Data.vi" "Distance (enc.)"() -> (w219:dbl)
        n187 = call-poly <vilib>:"PID.vi"("output range"=cluster{"output high":dbl, "output low":dbl} {"output high"=0.8, "output low"=-0.8} ("output range 2"), "PID gains"=T7 {"proportional gain (Kc)"=0.048, "integral time (Ti, min)"=0.015, "derivative time (Td, min)"=0.0} ("PID gains 2"), "process variable"=w220, "setpoint"=-1.0) -> ("output"=w222:dbl)  [unwired: 6 in, 1 out]
        n188 = global write "Robot Global Data.vi" "1-Y"(1.0 ("1-Y")) -> ()
        n189 = global write "Robot Global Data.vi" "1-X"(w222) -> ()
        n190 = Less?(x=w219, y=30.0) -> (x < y?=w217:bool)
      }
      n191 = while {
        tunnel: w201 -> [w215]
        tunnel: [w215] -> w200
        stop <- FALSE stop-if-true
        w213 = 0.0 ("1-X")
        n192 = global write "Robot Global Data.vi" "1-X"(w213) -> ()
        n193 = global write "Robot Global Data.vi" "1-Y"(w213) -> ()
      }
    }
    frame 8 {
      # "REAL 2 BALL"
      # "3 STAGE DECEL"
      # "?"
      # "3 STAGE DECELERATION AND LOW GEAR"
      # "APPRX GOAL"
      # "and STOP"
      # "DO IT AGAIN"
      # "PICK UP"
      # "COME BACK"
      # "TURN TO 0"
      # "FIRE"
      # "AIM"
      # "SICK DROPS"
      # "S CURVE"
      # "APPRX GOAL"
      # "DISRGARD ALL COMMENTS NOT IN CAPS"
      # "2 BALL?"
      n194 = while {
        tunnel: w311 -> [w540]
        tunnel: [w540] -> w310
        i -> [w533]
        stop <- w537 stop-if-true
        # "stop"
        n195 = global write "Robot Global Data.vi" "Arm Control"(-1.0 ("retainer num")) -> ()
        n196 = global write "Robot Global Data.vi" "In pos"(TRUE ("In pos")) -> ()
        n197 = global write "Robot Global Data.vi" "in ctl num"(i16 2 ("retainer num")) -> ()
        n198 = global write "Robot Global Data.vi" "1-Trigger"(TRUE ("In pos")) -> ()
        n199 = global write "Robot Global Data.vi" "retainer num"(i16 2 ("retainer num")) -> ()
        n200 = global write "Robot Global Data.vi" "1-X"(0.0 ("1-X")) -> ()
        n201 = Greater?(x=w533, y=15) -> (0:w537:bool)
        n202 = global write "Robot Global Data.vi" "1-Y"(0.0 ("1-X")) -> ()
        n203 = Wait (ms)(milliseconds to wait=u32 20) -> ()  [unwired: 1 out]
      }
      n204 = while {
        tunnel: w310 -> [w528]
        tunnel: [w528] -> w309
        i -> [w521]
        stop <- w525 stop-if-true
        # "stop"
        n205 = global write "Robot Global Data.vi" "In pos"(TRUE ("In pos")) -> ()
        n206 = global write "Robot Global Data.vi" "in ctl num"(i16 2 ("retainer num")) -> ()
        n207 = global write "Robot Global Data.vi" "retainer num"(i16 2 ("retainer num")) -> ()
        n208 = global write "Robot Global Data.vi" "Arm Control"(1.0 ("retainer num")) -> ()
        n209 = global write "Robot Global Data.vi" "1-X"(0.0 ("1-X")) -> ()
        n210 = Greater?(x=w521, y=17) -> (0:w525:bool)
        n211 = global write "Robot Global Data.vi" "1-Y"(0.0 ("1-X")) -> ()
        n212 = Wait (ms)(milliseconds to wait=u32 20) -> ()  [unwired: 1 out]
      }
      n213 = while {
        tunnel: w309 -> [w569]
        tunnel: [w569] -> w312
        stop <- w565 stop-if-true
        # "-23"
        # "218"
        # "thru the low bar"
        n214 = global read "Robot Global Data.vi" "CamTargetMem"() -> (w557:dbl)
        n215 = global read "Robot Global Data.vi" "Distance (enc.)"() -> (w567:dbl)
        n216 = global write "Robot Global Data.vi" "1-Y"(-0.8 ("1-X")) -> ()
        n217 = global read "Robot Global Data.vi" "Yaw"() -> (w560:dbl)
        n218 = Add(x=w557, y=0.01) -> (x+y=w558:dbl)
        n219 = global write "Robot Global Data.vi" "Pins / Intake timing"(0.0 ("Pins / Intake timing")) -> ()
        n220 = call-poly <vilib>:"PID.vi"("output range"=cluster{"output high":dbl, "output low":dbl} {"output high"=0.8, "output low"=-0.8} ("output range 2"), "PID gains"=T7 {"proportional gain (Kc)"=0.048, "integral time (Ti, min)"=0.015, "derivative time (Td, min)"=0.0} ("PID gains 2"), "process variable"=w560, "setpoint"=-26.0) -> ("output"=w562:dbl)  [unwired: 6 in, 1 out]
        n221 = global write "Robot Global Data.vi" "CamTargetReal"(w558) -> ()
        n222 = Greater?(x=w567, y=16.0) -> (0:w565:bool)
        n223 = global write "Robot Global Data.vi" "1-X"(w562) -> ()
        n224 = Wait (ms)(milliseconds to wait=u32 20) -> ()  [unwired: 1 out]
      }
      n225 = while {
        tunnel: w312 -> [w555]
        tunnel: [w555] -> w297
        stop <- w551 stop-if-true
        # "125"
        # "thru the low bar"
        n226 = global write "Robot Global Data.vi" "in ctl num"(i16 0 ("retainer num")) -> ()
        n227 = global read "Robot Global Data.vi" "Distance (enc.)"() -> (w553:dbl)
        n228 = global write "Robot Global Data.vi" "1-Y"(-1.0 ("1-X")) -> ()
        n229 = global read "Robot Global Data.vi" "Yaw"() -> (w546:dbl)
        n230 = call-poly <vilib>:"PID.vi"("output range"=cluster{"output high":dbl, "output low":dbl} {"output high"=0.8, "output low"=-0.8} ("output range 2"), "PID gains"=T7 {"proportional gain (Kc)"=0.048, "integral time (Ti, min)"=0.015, "derivative time (Td, min)"=0.0} ("PID gains 2"), "process variable"=w546, "setpoint"=4.0) -> ("output"=w548:dbl)  [unwired: 6 in, 1 out]
        n231 = Greater?(x=w553, y=100.0) -> (0:w551:bool)
        n232 = global write "Robot Global Data.vi" "1-X"(w548) -> ()
        n233 = global write "Robot Global Data.vi" "Slew"(0.2 ("1-Y")) -> ()
        n234 = global write "Robot Global Data.vi" "In pos"(TRUE ("In pos")) -> ()
        n235 = Wait (ms)(milliseconds to wait=u32 20) -> ()  [unwired: 1 out]
      }
      n236 = while {
        tunnel: w297 -> [w427]
        tunnel: [w427] -> w293
        stop <- w423 stop-if-true
        # "125"
        # "thru the low bar"
        n237 = global write "Robot Global Data.vi" "in ctl num"(i16 0 ("retainer num")) -> ()
        n238 = global read "Robot Global Data.vi" "Distance (enc.)"() -> (w425:dbl)
        n239 = global write "Robot Global Data.vi" "1-Y"(-1.0 ("1-X")) -> ()
        n240 = global read "Robot Global Data.vi" "Yaw"() -> (w418:dbl)
        n241 = call-poly <vilib>:"PID.vi"("output range"=cluster{"output high":dbl, "output low":dbl} {"output high"=0.8, "output low"=-0.8} ("output range 2"), "PID gains"=T7 {"proportional gain (Kc)"=0.048, "integral time (Ti, min)"=0.015, "derivative time (Td, min)"=0.0} ("PID gains 2"), "process variable"=w418, "setpoint"=4.0) -> ("output"=w420:dbl)  [unwired: 6 in, 1 out]
        n242 = Greater?(x=w425, y=175.0) -> (0:w423:bool)
        n243 = global write "Robot Global Data.vi" "1-X"(w420) -> ()
        n244 = global write "Robot Global Data.vi" "Slew"(0.2 ("1-Y")) -> ()
        n245 = global write "Robot Global Data.vi" "In pos"(TRUE ("In pos")) -> ()
        n246 = Wait (ms)(milliseconds to wait=u32 20) -> ()  [unwired: 1 out]
      }
      n247 = while {
        tunnel: w293 -> [w391]
        tunnel: [w391] -> w292
        stop <- w387 stop-if-true
        # "180"
        # "125"
        # "thru the low bar"
        n248 = global write "Robot Global Data.vi" "in ctl num"(i16 0 ("retainer num")) -> ()
        n249 = global read "Robot Global Data.vi" "Distance (enc.)"() -> (w389:dbl)
        n250 = global write "Robot Global Data.vi" "1-Trigger"(FALSE ("In pos")) -> ()
        n251 = global write "Robot Global Data.vi" "1-Y"(-0.65 ("1-X")) -> ()
        n252 = global read "Robot Global Data.vi" "Yaw"() -> (w382:dbl)
        n253 = call-poly <vilib>:"PID.vi"("output range"=cluster{"output high":dbl, "output low":dbl} {"output high"=0.8, "output low"=-0.8} ("output range 2"), "PID gains"=T7 {"proportional gain (Kc)"=0.048, "integral time (Ti, min)"=0.015, "derivative time (Td, min)"=0.0} ("PID gains 2"), "process variable"=w382, "setpoint"=4.0) -> ("output"=w384:dbl)  [unwired: 6 in, 1 out]
        n254 = Greater?(x=w389, y=185.0) -> (0:w387:bool)
        n255 = global write "Robot Global Data.vi" "1-X"(w384) -> ()
        n256 = global write "Robot Global Data.vi" "Slew"(0.2 ("1-Y")) -> ()
        n257 = global write "Robot Global Data.vi" "In pos"(TRUE ("In pos")) -> ()
        n258 = Wait (ms)(milliseconds to wait=u32 20) -> ()  [unwired: 1 out]
      }
      n259 = while {
        tunnel: w292 -> [w376]
        tunnel: [w376] -> w291
        stop <- w372 stop-if-true
        # "190"
        # "125"
        # "thru the low bar"
        n260 = global write "Robot Global Data.vi" "in ctl num"(i16 0 ("retainer num")) -> ()
        n261 = global read "Robot Global Data.vi" "Distance (enc.)"() -> (w374:dbl)
        n262 = global write "Robot Global Data.vi" "1-Trigger"(FALSE ("In pos")) -> ()
        n263 = global write "Robot Global Data.vi" "1-Y"(-0.55 ("1-X")) -> ()
        n264 = global read "Robot Global Data.vi" "Yaw"() -> (w367:dbl)
        n265 = call-poly <vilib>:"PID.vi"("output range"=cluster{"output high":dbl, "output low":dbl} {"output high"=0.8, "output low"=-0.8} ("output range 2"), "PID gains"=T7 {"proportional gain (Kc)"=0.048, "integral time (Ti, min)"=0.015, "derivative time (Td, min)"=0.0} ("PID gains 2"), "process variable"=w367, "setpoint"=4.0) -> ("output"=w369:dbl)  [unwired: 6 in, 1 out]
        n266 = Greater?(x=w374, y=195.0) -> (0:w372:bool)
        n267 = global write "Robot Global Data.vi" "1-X"(w369) -> ()
        n268 = global write "Robot Global Data.vi" "Slew"(0.2 ("1-Y")) -> ()
        n269 = global write "Robot Global Data.vi" "In pos"(TRUE ("In pos")) -> ()
        n270 = Wait (ms)(milliseconds to wait=u32 20) -> ()  [unwired: 1 out]
      }
      n271 = while {
        tunnel: w291 -> [w439]
        tunnel: [w439] -> w301
        stop <- w445 stop-if-true
        # "35"
        n272 = global write "Robot Global Data.vi" "in ctl num"(i16 0 ("retainer num")) -> ()
        n273 = global write "Robot Global Data.vi" "Slew"(0.2 ("1-Y")) -> ()
        n274 = global read "Robot Global Data.vi" "Yaw"() -> (w447:dbl)
        n275 = global write "Robot Global Data.vi" "retainer num"(i16 0 ("retainer num")) -> ()
        n276 = Greater?(x=w447, y=27.0) -> (0:w445:bool)
        n277 = global write "Robot Global Data.vi" "1-Y"(0.0 ("1-Y")) -> ()
        n278 = global write "Robot Global Data.vi" "1-X"(0.75 ("1-X")) -> ()
        n279 = Wait (ms)(milliseconds to wait=u32 20) -> ()  [unwired: 1 out]
      }
      n280 = while {
        tunnel: w301 -> [w437]
        tunnel: [w437] -> w299
        stop <- TRUE stop-if-true
        # "stop"
        n281 = global write "Robot Global Data.vi" "1-X"(0.0 ("1-X")) -> ()
        n282 = global write "Robot Global Data.vi" "1-Y"(0.0 ("1-X")) -> ()
        n283 = Wait (ms)(milliseconds to wait=u32 700) -> ()  [unwired: 1 out]
      }
      n284 = while {
        tunnel: w299 -> [w432]
        tunnel: [w432] -> w298
        stop <- TRUE stop-if-true
        # "stop"
        n285 = global write "Robot Global Data.vi" "1-X"(0.0 ("1-X")) -> ()
        n286 = global write "Robot Global Data.vi" "Slew"(0.2 ("1-Y")) -> ()
        n287 = global write "Robot Global Data.vi" "1-Y"(0.0 ("1-X")) -> ()
        n288 = Wait (ms)(milliseconds to wait=u32 20) -> ()  [unwired: 1 out]
      }
      n289 = while {
        tunnel: [w600] -> w315
        tunnel: w298 -> [w600]
        stop <- w602 stop-if-true
        n290 = global write "Robot Global Data.vi" "Shot Selector"(FALSE ("In pos")) -> ()
        n291 = global write "Robot Global Data.vi" "1-Button 8"(TRUE ("1-Button 8")) -> ()
        n292 = global read "Robot Global Data.vi" "4?"() -> (w602:bool)
        n293 = Wait (ms)(milliseconds to wait=u32 20) -> ()  [unwired: 1 out]
      }
      n294 = while {
        tunnel: w315 -> [w586]
        tunnel: [w586] -> w316
        stop <- TRUE stop-if-true
        n295 = Wait (ms)(milliseconds to wait=u32 200) -> ()  [unwired: 1 out]
      }
      n296 = while {
        tunnel: [w597] -> w317
        tunnel: w316 -> [w597]
        i -> [w595]
        stop <- w593 stop-if-true
        n297 = global write "Robot Global Data.vi" "Shoot!"(TRUE ("1-Button 8")) -> ()
        n298 = Greater?(x=w595, y=5) -> (0:w593:bool)
        n299 = Wait (ms)(milliseconds to wait=u32 20) -> ()  [unwired: 1 out]
      }
      n300 = while {
        tunnel: [w591] -> w314
        tunnel: w317 -> [w591]
        stop <- TRUE stop-if-true
        n301 = global write "Robot Global Data.vi" "Shoot!"(FALSE ("1-Button 8")) -> ()
        n302 = Wait (ms)(milliseconds to wait=u32 500) -> ()  [unwired: 1 out]
      }
      n303 = while {
        tunnel: w314 -> [w583]
        tunnel: [w583] -> w307
        stop <- TRUE stop-if-true
        n304 = global write "Robot Global Data.vi" "1-Button 8"(FALSE ("1-Button 8")) -> ()
        n305 = Wait (ms)(milliseconds to wait=u32 20) -> ()  [unwired: 1 out]
      }
      n306 = while {
        tunnel: w307 -> [w513]
        tunnel: [w513] -> w308
        stop <- w515 stop-if-true
        # "13"
        n307 = global read "Robot Global Data.vi" "Yaw"() -> (w512:dbl)
        n308 = global write "Robot Global Data.vi" "1-Button 8"(FALSE ("1-Button 8")) -> ()
        n309 = Sign(1:w512) -> (0:w511:dbl)
        n310 = global read "Robot Global Data.vi" "Yaw"() -> (w518:dbl)
        n311 = Multiply(x=-0.65, y=w511) -> (x*y=w509:dbl)
        n312 = global write "Robot Global Data.vi" "retainer num"(i16 2 ("retainer num")) -> ()
        n313 = Absolute Value(x=w518) -> (abs(x)=w517:dbl)
        n314 = Less?(x=w517, y=21.0) -> (x < y?=w515:bool)
        n315 = global write "Robot Global Data.vi" "1-X"(w509) -> ()
        n316 = Wait (ms)(milliseconds to wait=u32 20) -> ()  [unwired: 1 out]
      }
      n317 = while {
        tunnel: w308 -> [w505]
        tunnel: [w505] -> w306
        stop <- w501 stop-if-true
        # "218"
        # "thru the low bar"
        n318 = global write "Robot Global Data.vi" "in ctl num"(i16 0 ("retainer num")) -> ()
        n319 = global read "Robot Global Data.vi" "Distance (enc.)"() -> (w503:dbl)
        n320 = global write "Robot Global Data.vi" "1-Y"(1.0 ("1-X")) -> ()
        n321 = global read "Robot Global Data.vi" "Yaw"() -> (w496:dbl)
        n322 = call-poly <vilib>:"PID.vi"("output range"=cluster{"output high":dbl, "output low":dbl} {"output high"=0.8, "output low"=-0.8} ("output range 2"), "PID gains"=T7 {"proportional gain (Kc)"=0.048, "integral time (Ti, min)"=0.015, "derivative time (Td, min)"=0.0} ("PID gains 2"), "process variable"=w496, "setpoint"=4.0) -> ("output"=w498:dbl)  [unwired: 6 in, 1 out]
        n323 = Less?(x=w503, y=90.0) -> (x < y?=w501:bool)
        n324 = global write "Robot Global Data.vi" "In pos"(TRUE ("In pos")) -> ()
        n325 = global write "Robot Global Data.vi" "1-X"(w498) -> ()
        n326 = Wait (ms)(milliseconds to wait=u32 20) -> ()  [unwired: 1 out]
      }
      n327 = while {
        tunnel: w306 -> [w492]
        tunnel: [w492] -> w300
        stop <- w488 stop-if-true
        # "32"
        # "thru the low bar"
        n328 = global write "Robot Global Data.vi" "in ctl num"(i16 2 ("retainer num")) -> ()
        n329 = global read "Robot Global Data.vi" "Distance (enc.)"() -> (w490:dbl)
        n330 = global write "Robot Global Data.vi" "1-Y"(0.66 ("1-X")) -> ()
        n331 = global read "Robot Global Data.vi" "Yaw"() -> (w483:dbl)
        n332 = call-poly <vilib>:"PID.vi"("output range"=cluster{"output high":dbl, "output low":dbl} {"output high"=0.8, "output low"=-0.8} ("output range 2"), "PID gains"=T7 {"proportional gain (Kc)"=0.048, "integral time (Ti, min)"=0.015, "derivative time (Td, min)"=0.0} ("PID gains 2"), "process variable"=w483, "setpoint"=2.0) -> ("output"=w485:dbl)  [unwired: 6 in, 1 out]
        n333 = Less?(x=w490, y=42.0) -> (x < y?=w488:bool)
        n334 = global write "Robot Global Data.vi" "1-Trigger"(TRUE ("In pos")) -> ()
        n335 = global write "Robot Global Data.vi" "In pos"(TRUE ("In pos")) -> ()
        n336 = global write "Robot Global Data.vi" "1-X"(w485) -> ()
        n337 = Wait (ms)(milliseconds to wait=u32 20) -> ()  [unwired: 1 out]
      }
      n338 = while {
        tunnel: w300 -> [w578]
        tunnel: [w577] -> w290
        i -> [w575]
        stop <- w576 stop-if-true
        w580 = 0.0 ("1-X")
        n339 = call <vilib>:"WPI_EncoderReset.vi"("EncoderDevRef"=w578) -> ("EncoderDevRef"=w577:T3)  [unwired: 9 in, 1 out]
        n340 = Wait (ms)(milliseconds to wait=u32 20) -> ()  [unwired: 1 out]
        n341 = global write "Robot Global Data.vi" "1-X"(w580) -> ()
        n342 = Greater?(x=w575, y=10) -> (0:w576:bool)
        n343 = global write "Robot Global Data.vi" "1-Y"(w580) -> ()
      }
      n344 = while {
        tunnel: w290 -> [w460]
        tunnel: [w460] -> w287
        stop <- w456 stop-if-true
        # "115"
        # "218"
        # "thru the low bar"
        n345 = global write "Robot Global Data.vi" "in ctl num"(i16 2 ("retainer num")) -> ()
        n346 = global read "Robot Global Data.vi" "Distance (enc.)"() -> (w458:dbl)
        n347 = global write "Robot Global Data.vi" "1-Y"(-0.9 ("1-X")) -> ()
        n348 = global read "Robot Global Data.vi" "Yaw"() -> (w451:dbl)
        n349 = call-poly <vilib>:"PID.vi"("output range"=cluster{"output high":dbl, "output low":dbl} {"output high"=0.8, "output low"=-0.8} ("output range 2"), "PID gains"=T7 {"proportional gain (Kc)"=0.048, "integral time (Ti, min)"=0.015, "derivative time (Td, min)"=0.0} ("PID gains 2"), "process variable"=w451, "setpoint"=-1.0) -> ("output"=w453:dbl)  [unwired: 6 in, 1 out]
        n350 = Greater?(x=w458, y=70.0) -> (0:w456:bool)
        n351 = global write "Robot Global Data.vi" "In pos"(TRUE ("In pos")) -> ()
        n352 = global write "Robot Global Data.vi" "1-X"(w453) -> ()
        n353 = Wait (ms)(milliseconds to wait=u32 20) -> ()  [unwired: 1 out]
      }
      n354 = while {
        tunnel: w287 -> [w361]
        tunnel: [w361] -> w289
        stop <- w357 stop-if-true
        # "125"
        # "thru the low bar"
        n355 = global write "Robot Global Data.vi" "in ctl num"(i16 0 ("retainer num")) -> ()
        n356 = global read "Robot Global Data.vi" "Distance (enc.)"() -> (w359:dbl)
        n357 = global write "Robot Global Data.vi" "1-Y"(-1.0 ("1-X")) -> ()
        n358 = global read "Robot Global Data.vi" "Yaw"() -> (w352:dbl)
        n359 = call-poly <vilib>:"PID.vi"("output range"=cluster{"output high":dbl, "output low":dbl} {"output high"=0.8, "output low"=-0.8} ("output range 2"), "PID gains"=T7 {"proportional gain (Kc)"=0.048, "integral time (Ti, min)"=0.015, "derivative time (Td, min)"=0.0} ("PID gains 2"), "process variable"=w352, "setpoint"=4.0) -> ("output"=w354:dbl)  [unwired: 6 in, 1 out]
        n360 = Greater?(x=w359, y=165.0) -> (0:w357:bool)
        n361 = global write "Robot Global Data.vi" "1-X"(w354) -> ()
        n362 = global write "Robot Global Data.vi" "Slew"(0.2 ("1-Y")) -> ()
        n363 = global write "Robot Global Data.vi" "In pos"(TRUE ("In pos")) -> ()
        n364 = Wait (ms)(milliseconds to wait=u32 20) -> ()  [unwired: 1 out]
      }
      n365 = while {
        tunnel: w289 -> [w347]
        tunnel: [w347] -> w288
        stop <- w343 stop-if-true
        # "180"
        # "125"
        # "thru the low bar"
        n366 = global write "Robot Global Data.vi" "in ctl num"(i16 0 ("retainer num")) -> ()
        n367 = global read "Robot Global Data.vi" "Distance (enc.)"() -> (w345:dbl)
        n368 = global write "Robot Global Data.vi" "1-Trigger"(FALSE ("In pos")) -> ()
        n369 = global write "Robot Global Data.vi" "1-Y"(-0.65 ("1-X")) -> ()
        n370 = global read "Robot Global Data.vi" "Yaw"() -> (w338:dbl)
        n371 = call-poly <vilib>:"PID.vi"("output range"=cluster{"output high":dbl, "output low":dbl} {"output high"=0.8, "output low"=-0.8} ("output range 2"), "PID gains"=T7 {"proportional gain (Kc)"=0.048, "integral time (Ti, min)"=0.015, "derivative time (Td, min)"=0.0} ("PID gains 2"), "process variable"=w338, "setpoint"=4.0) -> ("output"=w340:dbl)  [unwired: 6 in, 1 out]
        n372 = Greater?(x=w345, y=175.0) -> (0:w343:bool)
        n373 = global write "Robot Global Data.vi" "1-X"(w340) -> ()
        n374 = global write "Robot Global Data.vi" "Slew"(0.2 ("1-Y")) -> ()
        n375 = global write "Robot Global Data.vi" "In pos"(TRUE ("In pos")) -> ()
        n376 = Wait (ms)(milliseconds to wait=u32 20) -> ()  [unwired: 1 out]
      }
      n377 = while {
        tunnel: w288 -> [w332]
        tunnel: [w332] -> w286
        stop <- w328 stop-if-true
        # "190"
        # "125"
        # "thru the low bar"
        n378 = global write "Robot Global Data.vi" "in ctl num"(i16 0 ("retainer num")) -> ()
        n379 = global read "Robot Global Data.vi" "Distance (enc.)"() -> (w330:dbl)
        n380 = global write "Robot Global Data.vi" "1-Trigger"(FALSE ("In pos")) -> ()
        n381 = global write "Robot Global Data.vi" "1-Y"(-0.55 ("1-X")) -> ()
        n382 = global read "Robot Global Data.vi" "Yaw"() -> (w323:dbl)
        n383 = call-poly <vilib>:"PID.vi"("output range"=cluster{"output high":dbl, "output low":dbl} {"output high"=0.8, "output low"=-0.8} ("output range 2"), "PID gains"=T7 {"proportional gain (Kc)"=0.048, "integral time (Ti, min)"=0.015, "derivative time (Td, min)"=0.0} ("PID gains 2"), "process variable"=w323, "setpoint"=4.0) -> ("output"=w325:dbl)  [unwired: 6 in, 1 out]
        n384 = Greater?(x=w330, y=185.0) -> (0:w328:bool)
        n385 = global write "Robot Global Data.vi" "1-X"(w325) -> ()
        n386 = global write "Robot Global Data.vi" "Slew"(0.2 ("1-Y")) -> ()
        n387 = global write "Robot Global Data.vi" "In pos"(TRUE ("In pos")) -> ()
        n388 = Wait (ms)(milliseconds to wait=u32 20) -> ()  [unwired: 1 out]
      }
      n389 = while {
        tunnel: w286 -> [w413]
        tunnel: [w413] -> w296
        stop <- w409 stop-if-true
        # "25"
        n390 = global write "Robot Global Data.vi" "in ctl num"(i16 0 ("retainer num")) -> ()
        n391 = global write "Robot Global Data.vi" "Slew"(0.2 ("1-Y")) -> ()
        n392 = global read "Robot Global Data.vi" "Yaw"() -> (w411:dbl)
        n393 = global write "Robot Global Data.vi" "retainer num"(i16 0 ("retainer num")) -> ()
        n394 = global write "Robot Global Data.vi" "1-Trigger"(FALSE ("In pos")) -> ()
        n395 = Greater?(x=w411, y=33.0) -> (0:w409:bool)
        n396 = global write "Robot Global Data.vi" "1-Y"(0.0 ("1-Y")) -> ()
        n397 = global write "Robot Global Data.vi" "1-X"(0.75 ("1-X")) -> ()
        n398 = Wait (ms)(milliseconds to wait=u32 20) -> ()  [unwired: 1 out]
      }
      n399 = while {
        tunnel: w296 -> [w401]
        tunnel: [w401] -> w295
        stop <- TRUE stop-if-true
        # "stop"
        n400 = global write "Robot Global Data.vi" "1-X"(0.0 ("1-X")) -> ()
        n401 = global write "Robot Global Data.vi" "1-Y"(0.0 ("1-X")) -> ()
        n402 = Wait (ms)(milliseconds to wait=u32 700) -> ()  [unwired: 1 out]
      }
      n403 = while {
        tunnel: w295 -> [w396]
        tunnel: [w396] -> w294
        stop <- TRUE stop-if-true
        # "stop"
        n404 = global write "Robot Global Data.vi" "1-X"(0.0 ("1-X")) -> ()
        n405 = global write "Robot Global Data.vi" "Slew"(0.2 ("1-Y")) -> ()
        n406 = global write "Robot Global Data.vi" "1-Y"(0.0 ("1-X")) -> ()
        n407 = Wait (ms)(milliseconds to wait=u32 20) -> ()  [unwired: 1 out]
      }
      n408 = while {
        tunnel: [w477] -> w305
        tunnel: w294 -> [w477]
        stop <- w479 stop-if-true
        n409 = global write "Robot Global Data.vi" "Shot Selector"(FALSE ("In pos")) -> ()
        n410 = global write "Robot Global Data.vi" "1-Button 8"(TRUE ("1-Button 8")) -> ()
        n411 = global read "Robot Global Data.vi" "4?"() -> (w479:bool)
        n412 = Wait (ms)(milliseconds to wait=u32 20) -> ()  [unwired: 1 out]
      }
      n413 = while {
        tunnel: w305 -> [w463]
        tunnel: [w463] -> w303
        stop <- TRUE stop-if-true
        n414 = Wait (ms)(milliseconds to wait=u32 250) -> ()  [unwired: 1 out]
      }
      n415 = while {
        tunnel: [w474] -> w304
        tunnel: w303 -> [w474]
        i -> [w472]
        stop <- w470 stop-if-true
        n416 = global write "Robot Global Data.vi" "Shoot!"(TRUE ("1-Button 8")) -> ()
        n417 = Greater?(x=w472, y=5) -> (0:w470:bool)
        n418 = Wait (ms)(milliseconds to wait=u32 20) -> ()  [unwired: 1 out]
      }
      n419 = while {
        tunnel: [w468] -> w302
        tunnel: w304 -> [w468]
        stop <- TRUE stop-if-true
        n420 = global write "Robot Global Data.vi" "Shoot!"(FALSE ("1-Button 8")) -> ()
        n421 = Wait (ms)(milliseconds to wait=u32 700) -> ()  [unwired: 1 out]
      }
      n422 = while {
        tunnel: w302 -> [w573]
        tunnel: [w573] -> w313
        stop <- FALSE stop-if-true
        w571 = 0.0 ("1-X")
        n423 = global write "Robot Global Data.vi" "1-X"(w571) -> ()
        n424 = global write "Robot Global Data.vi" "1-Y"(w571) -> ()
      }
    }
    frame 9 {
      # "Do nothing"
      n425 = while {
        tunnel: w604 -> [w605]
        tunnel: [w605] -> w603
        stop <- FALSE stop-if-true
        n426 = Wait (ms)(milliseconds to wait=u32 30000) -> ()  [unwired: 1 out]
      }
    }
    frame 10 {
      # "OLD 2 BALL"
      # "DO IT AGAIN"
      # "PICK UP"
      # "COME BACK"
      # "TURN TO 0"
      # "FIRE"
      # "AIM"
      # "SICK DROPS"
      # "S CURVE"
      # "APPRX GOAL"
      # "DISRGARD ALL COMMENTS NOT IN CAPS"
      # "2 BALL?"
      n427 = while {
        tunnel: w625 -> [w745]
        tunnel: [w745] -> w622
        i -> [w738]
        stop <- w742 stop-if-true
        # "stop"
        n428 = global write "Robot Global Data.vi" "Arm Control"(-1.0 ("retainer num")) -> ()
        n429 = global write "Robot Global Data.vi" "In pos"(TRUE ("In pos")) -> ()
        n430 = global write "Robot Global Data.vi" "in ctl num"(i16 2 ("retainer num")) -> ()
        n431 = global write "Robot Global Data.vi" "1-Trigger"(FALSE ("In pos")) -> ()
        n432 = global write "Robot Global Data.vi" "retainer num"(i16 0 ("retainer num")) -> ()
        n433 = global write "Robot Global Data.vi" "1-X"(0.0 ("1-X")) -> ()
        n434 = Greater?(x=w738, y=15) -> (0:w742:bool)
        n435 = global write "Robot Global Data.vi" "1-Y"(0.0 ("1-X")) -> ()
        n436 = Wait (ms)(milliseconds to wait=u32 20) -> ()  [unwired: 1 out]
      }
      n437 = while {
        tunnel: w622 -> [w724]
        tunnel: [w724] -> w621
        i -> [w717]
        stop <- w721 stop-if-true
        # "stop"
        n438 = global write "Robot Global Data.vi" "In pos"(TRUE ("In pos")) -> ()
        n439 = global write "Robot Global Data.vi" "in ctl num"(i16 2 ("retainer num")) -> ()
        n440 = global write "Robot Global Data.vi" "retainer num"(i16 0 ("retainer num")) -> ()
        n441 = global write "Robot Global Data.vi" "Arm Control"(1.0 ("retainer num")) -> ()
        n442 = global write "Robot Global Data.vi" "1-X"(0.0 ("1-X")) -> ()
        n443 = Greater?(x=w717, y=17) -> (0:w721:bool)
        n444 = global write "Robot Global Data.vi" "1-Y"(0.0 ("1-X")) -> ()
        n445 = Wait (ms)(milliseconds to wait=u32 20) -> ()  [unwired: 1 out]
      }
      n446 = while {
        tunnel: w621 -> [w775]
        tunnel: [w775] -> w626
        stop <- w771 stop-if-true
        # "218"
        # "thru the low bar"
        n447 = global read "Robot Global Data.vi" "Distance (enc.)"() -> (w773:dbl)
        n448 = global write "Robot Global Data.vi" "1-Y"(-1.0 ("1-X")) -> ()
        n449 = global read "Robot Global Data.vi" "Yaw"() -> (w766:dbl)
        n450 = global write "Robot Global Data.vi" "Pins / Intake timing"(0.0 ("Pins / Intake timing")) -> ()
        n451 = call-poly <vilib>:"PID.vi"("output range"=cluster{"output high":dbl, "output low":dbl} {"output high"=0.8, "output low"=-0.8} ("output range 2"), "PID gains"=T7 {"proportional gain (Kc)"=0.048, "integral time (Ti, min)"=0.015, "derivative time (Td, min)"=0.0} ("PID gains 2"), "process variable"=w766, "setpoint"=-36.0) -> ("output"=w768:dbl)  [unwired: 6 in, 1 out]
        n452 = Greater?(x=w773, y=26.0) -> (0:w771:bool)
        n453 = global write "Robot Global Data.vi" "1-X"(w768) -> ()
        n454 = Wait (ms)(milliseconds to wait=u32 20) -> ()  [unwired: 1 out]
      }
      n455 = while {
        tunnel: w626 -> [w763]
        tunnel: [w763] -> w624
        stop <- w759 stop-if-true
        # "218"
        # "thru the low bar"
        n456 = global write "Robot Global Data.vi" "in ctl num"(i16 0 ("retainer num")) -> ()
        n457 = global read "Robot Global Data.vi" "Distance (enc.)"() -> (w761:dbl)
        n458 = global write "Robot Global Data.vi" "1-Y"(-1.0 ("1-X")) -> ()
        n459 = global read "Robot Global Data.vi" "Yaw"() -> (w754:dbl)
        n460 = call-poly <vilib>:"PID.vi"("output range"=cluster{"output high":dbl, "output low":dbl} {"output high"=0.8, "output low"=-0.8} ("output range 2"), "PID gains"=T7 {"proportional gain (Kc)"=0.048, "integral time (Ti, min)"=0.015, "derivative time (Td, min)"=0.0} ("PID gains 2"), "process variable"=w754, "setpoint"=2.0) -> ("output"=w756:dbl)  [unwired: 6 in, 1 out]
        n461 = Greater?(x=w761, y=175.0) -> (0:w759:bool)
        n462 = global write "Robot Global Data.vi" "In pos"(TRUE ("In pos")) -> ()
        n463 = global write "Robot Global Data.vi" "1-X"(w756) -> ()
        n464 = Wait (ms)(milliseconds to wait=u32 20) -> ()  [unwired: 1 out]
      }
      n465 = while {
        tunnel: w624 -> [w733]
        tunnel: [w733] -> w623
        stop <- w730 stop-if-true
        # "218"
        n466 = global read "Robot Global Data.vi" "Yaw"() -> (w728:dbl)
        n467 = global write "Robot Global Data.vi" "1-Trigger"(FALSE ("In pos")) -> ()
        n468 = global write "Robot Global Data.vi" "1-X"(0.8 ("1-X")) -> ()
        n469 = global write "Robot Global Data.vi" "1-Y"(0.0 ("1-X")) -> ()
        n470 = Greater?(x=w728, y=8.0) -> (0:w730:bool)
        n471 = global write "Robot Global Data.vi" "In pos"(TRUE ("In pos")) -> ()
        n472 = Wait (ms)(milliseconds to wait=u32 20) -> ()  [unwired: 1 out]
      }
      n473 = while {
        tunnel: w623 -> [w750]
        tunnel: [w750] -> w616
        stop <- TRUE stop-if-true
        # "stop"
        n474 = global write "Robot Global Data.vi" "1-X"(0.0 ("1-X")) -> ()
        n475 = global write "Robot Global Data.vi" "1-Y"(0.0 ("1-X")) -> ()
        n476 = Wait (ms)(milliseconds to wait=u32 500) -> ()  [unwired: 1 out]
      }
      n477 = while {
        tunnel: [w803] -> w629
        tunnel: w616 -> [w803]
        stop <- w805 stop-if-true
        n478 = global write "Robot Global Data.vi" "Shot Selector"(FALSE ("In pos")) -> ()
        n479 = global write "Robot Global Data.vi" "1-Button 8"(TRUE ("1-Button 8")) -> ()
        n480 = global read "Robot Global Data.vi" "4?"() -> (w805:bool)
        n481 = Wait (ms)(milliseconds to wait=u32 20) -> ()  [unwired: 1 out]
      }
      n482 = while {
        tunnel: w629 -> [w789]
        tunnel: [w789] -> w630
        stop <- TRUE stop-if-true
        n483 = Wait (ms)(milliseconds to wait=u32 350) -> ()  [unwired: 1 out]
      }
      n484 = while {
        tunnel: [w800] -> w631
        tunnel: w630 -> [w800]
        i -> [w798]
        stop <- w796 stop-if-true
        n485 = global write "Robot Global Data.vi" "Shoot!"(TRUE ("1-Button 8")) -> ()
        n486 = Greater?(x=w798, y=5) -> (0:w796:bool)
        n487 = Wait (ms)(milliseconds to wait=u32 20) -> ()  [unwired: 1 out]
      }
      n488 = while {
        tunnel: [w794] -> w628
        tunnel: w631 -> [w794]
        stop <- TRUE stop-if-true
        n489 = global write "Robot Global Data.vi" "Shoot!"(FALSE ("1-Button 8")) -> ()
        n490 = Wait (ms)(milliseconds to wait=u32 700) -> ()  [unwired: 1 out]
      }
      n491 = while {
        tunnel: w628 -> [w786]
        tunnel: [w786] -> w619
        stop <- TRUE stop-if-true
        n492 = global write "Robot Global Data.vi" "1-Button 8"(FALSE ("1-Button 8")) -> ()
        n493 = Wait (ms)(milliseconds to wait=u32 20) -> ()  [unwired: 1 out]
      }
      n494 = while {
        tunnel: w619 -> [w709]
        tunnel: [w709] -> w620
        stop <- w711 stop-if-true
        n495 = global read "Robot Global Data.vi" "Yaw"() -> (w708:dbl)
        n496 = global write "Robot Global Data.vi" "1-Button 8"(FALSE ("1-Button 8")) -> ()
        n497 = Sign(1:w708) -> (0:w707:dbl)
        n498 = global read "Robot Global Data.vi" "Yaw"() -> (w714:dbl)
        n499 = Multiply(x=-0.65, y=w707) -> (x*y=w705:dbl)
        n500 = Absolute Value(x=w714) -> (abs(x)=w713:dbl)
        n501 = Less?(x=w713, y=13.0) -> (x < y?=w711:bool)
        n502 = global write "Robot Global Data.vi" "1-X"(w705) -> ()
        n503 = Wait (ms)(milliseconds to wait=u32 20) -> ()  [unwired: 1 out]
      }
      n504 = while {
        tunnel: w620 -> [w702]
        tunnel: [w702] -> w618
        stop <- w698 stop-if-true
        # "218"
        # "thru the low bar"
        n505 = global write "Robot Global Data.vi" "in ctl num"(i16 0 ("retainer num")) -> ()
        n506 = global read "Robot Global Data.vi" "Distance (enc.)"() -> (w700:dbl)
        n507 = global write "Robot Global Data.vi" "1-Y"(1.0 ("1-X")) -> ()
        n508 = global read "Robot Global Data.vi" "Yaw"() -> (w693:dbl)
        n509 = call-poly <vilib>:"PID.vi"("output range"=cluster{"output high":dbl, "output low":dbl} {"output high"=0.8, "output low"=-0.8} ("output range 2"), "PID gains"=T7 {"proportional gain (Kc)"=0.048, "integral time (Ti, min)"=0.015, "derivative time (Td, min)"=0.0} ("PID gains 2"), "process variable"=w693, "setpoint"=7.0) -> ("output"=w695:dbl)  [unwired: 6 in, 1 out]
        n510 = Less?(x=w700, y=120.0) -> (x < y?=w698:bool)
        n511 = global write "Robot Global Data.vi" "In pos"(TRUE ("In pos")) -> ()
        n512 = global write "Robot Global Data.vi" "1-X"(w695) -> ()
        n513 = Wait (ms)(milliseconds to wait=u32 20) -> ()  [unwired: 1 out]
      }
      n514 = while {
        tunnel: w618 -> [w689]
        tunnel: [w689] -> w617
        stop <- w685 stop-if-true
        # "218"
        # "thru the low bar"
        n515 = global write "Robot Global Data.vi" "in ctl num"(i16 2 ("retainer num")) -> ()
        n516 = global read "Robot Global Data.vi" "Distance (enc.)"() -> (w687:dbl)
        n517 = global write "Robot Global Data.vi" "1-Y"(1.0 ("1-X")) -> ()
        n518 = global read "Robot Global Data.vi" "Yaw"() -> (w680:dbl)
        n519 = call-poly <vilib>:"PID.vi"("output range"=cluster{"output high":dbl, "output low":dbl} {"output high"=0.8, "output low"=-0.8} ("output range 2"), "PID gains"=T7 {"proportional gain (Kc)"=0.048, "integral time (Ti, min)"=0.015, "derivative time (Td, min)"=0.0} ("PID gains 2"), "process variable"=w680, "setpoint"=9.0) -> ("output"=w682:dbl)  [unwired: 6 in, 1 out]
        n520 = Less?(x=w687, y=20.0) -> (x < y?=w685:bool)
        n521 = global write "Robot Global Data.vi" "In pos"(TRUE ("In pos")) -> ()
        n522 = global write "Robot Global Data.vi" "1-X"(w682) -> ()
        n523 = Wait (ms)(milliseconds to wait=u32 20) -> ()  [unwired: 1 out]
      }
      n524 = while {
        tunnel: w617 -> [w783]
        tunnel: [w783] -> w615
        stop <- TRUE stop-if-true
        w781 = 0.0 ("1-X")
        n525 = Wait (ms)(milliseconds to wait=u32 20) -> ()  [unwired: 1 out]
        n526 = global write "Robot Global Data.vi" "1-X"(w781) -> ()
        n527 = global write "Robot Global Data.vi" "1-Y"(w781) -> ()
      }
      n528 = while {
        tunnel: w615 -> [w657]
        tunnel: [w657] -> w611
        stop <- w653 stop-if-true
        # "218"
        # "thru the low bar"
        n529 = global write "Robot Global Data.vi" "in ctl num"(i16 2 ("retainer num")) -> ()
        n530 = global read "Robot Global Data.vi" "Distance (enc.)"() -> (w655:dbl)
        n531 = global write "Robot Global Data.vi" "1-Y"(-1.0 ("1-X")) -> ()
        n532 = global read "Robot Global Data.vi" "Yaw"() -> (w648:dbl)
        n533 = call-poly <vilib>:"PID.vi"("output range"=cluster{"output high":dbl, "output low":dbl} {"output high"=0.8, "output low"=-0.8} ("output range 2"), "PID gains"=T7 {"proportional gain (Kc)"=0.048, "integral time (Ti, min)"=0.015, "derivative time (Td, min)"=0.0} ("PID gains 2"), "process variable"=w648, "setpoint"=0.0) -> ("output"=w650:dbl)  [unwired: 6 in, 1 out]
        n534 = Greater?(x=w655, y=175.0) -> (0:w653:bool)
        n535 = global write "Robot Global Data.vi" "In pos"(TRUE ("In pos")) -> ()
        n536 = global write "Robot Global Data.vi" "1-X"(w650) -> ()
        n537 = Wait (ms)(milliseconds to wait=u32 20) -> ()  [unwired: 1 out]
      }
      n538 = while {
        tunnel: w611 -> [w639]
        tunnel: [w639] -> w612
        stop <- w636 stop-if-true
        # "218"
        # "thru the low bar"
        n539 = global read "Robot Global Data.vi" "Yaw"() -> (w634:dbl)
        n540 = global write "Robot Global Data.vi" "1-X"(0.9 ("1-X")) -> ()
        n541 = global write "Robot Global Data.vi" "in ctl num"(i16 0 ("retainer num")) -> ()
        n542 = global write "Robot Global Data.vi" "1-Y"(0.0 ("1-X")) -> ()
        n543 = Greater?(x=w634, y=8.0) -> (0:w636:bool)
        n544 = global write "Robot Global Data.vi" "In pos"(TRUE ("In pos")) -> ()
        n545 = Wait (ms)(milliseconds to wait=u32 20) -> ()  [unwired: 1 out]
      }
      n546 = while {
        tunnel: w612 -> [w644]
        tunnel: [w644] -> w614
        stop <- TRUE stop-if-true
        # "stop"
        n547 = global write "Robot Global Data.vi" "1-X"(0.0 ("1-X")) -> ()
        n548 = global write "Robot Global Data.vi" "1-Y"(0.0 ("1-X")) -> ()
        n549 = Wait (ms)(milliseconds to wait=u32 500) -> ()  [unwired: 1 out]
      }
      n550 = while {
        tunnel: [w675] -> w613
        tunnel: w614 -> [w675]
        stop <- w677 stop-if-true
        n551 = global write "Robot Global Data.vi" "Shot Selector"(FALSE ("In pos")) -> ()
        n552 = global write "Robot Global Data.vi" "1-Button 8"(TRUE ("1-Button 8")) -> ()
        n553 = global read "Robot Global Data.vi" "4?"() -> (w677:bool)
        n554 = Wait (ms)(milliseconds to wait=u32 20) -> ()  [unwired: 1 out]
      }
      n555 = while {
        tunnel: w613 -> [w661]
        tunnel: [w661] -> w609
        stop <- TRUE stop-if-true
        n556 = global write "Robot Global Data.vi" "1-Button 8"(FALSE ("1-Button 8")) -> ()
        n557 = Wait (ms)(milliseconds to wait=u32 350) -> ()  [unwired: 1 out]
      }
      n558 = while {
        tunnel: [w672] -> w610
        tunnel: w609 -> [w672]
        i -> [w670]
        stop <- w668 stop-if-true
        n559 = global write "Robot Global Data.vi" "Shoot!"(TRUE ("1-Button 8")) -> ()
        n560 = Greater?(x=w670, y=5) -> (0:w668:bool)
        n561 = Wait (ms)(milliseconds to wait=u32 20) -> ()  [unwired: 1 out]
      }
      n562 = while {
        tunnel: [w666] -> w608
        tunnel: w610 -> [w666]
        stop <- TRUE stop-if-true
        n563 = global write "Robot Global Data.vi" "Shoot!"(FALSE ("1-Button 8")) -> ()
        n564 = Wait (ms)(milliseconds to wait=u32 700) -> ()  [unwired: 1 out]
      }
      n565 = while {
        tunnel: w608 -> [w779]
        tunnel: [w779] -> w627
        stop <- FALSE stop-if-true
        w777 = 0.0 ("1-X")
        n566 = global write "Robot Global Data.vi" "1-X"(w777) -> ()
        n567 = global write "Robot Global Data.vi" "1-Y"(w777) -> ()
      }
    }
    frame 11 {
      # "OLD 2 BALL"
      # "THIS  IS A TWO BALL THAT HAS WORKED IN UNDER 14 SECONDS"
      # "and STOP"
      # "DO IT AGAIN"
      # "PICK UP"
      # "COME BACK"
      # "TURN TO 0"
      # "FIRE"
      # "AIM"
      # "SICK DROPS"
      # "S CURVE"
      # "APPRX GOAL"
      # "DISRGARD ALL COMMENTS NOT IN CAPS"
      # "2 BALL?"
      n568 = while {
        tunnel: w823 -> [w962]
        tunnel: [w962] -> w822
        i -> [w955]
        stop <- w959 stop-if-true
        # "stop"
        n569 = global write "Robot Global Data.vi" "Arm Control"(-1.0 ("retainer num")) -> ()
        n570 = global write "Robot Global Data.vi" "In pos"(TRUE ("In pos")) -> ()
        n571 = global write "Robot Global Data.vi" "in ctl num"(i16 2 ("retainer num")) -> ()
        n572 = global write "Robot Global Data.vi" "1-Trigger"(TRUE ("In pos")) -> ()
        n573 = global write "Robot Global Data.vi" "retainer num"(i16 2 ("retainer num")) -> ()
        n574 = global write "Robot Global Data.vi" "1-X"(0.0 ("1-X")) -> ()
        n575 = Greater?(x=w955, y=15) -> (0:w959:bool)
        n576 = global write "Robot Global Data.vi" "1-Y"(0.0 ("1-X")) -> ()
        n577 = Wait (ms)(milliseconds to wait=u32 20) -> ()  [unwired: 1 out]
      }
      n578 = while {
        tunnel: w822 -> [w950]
        tunnel: [w950] -> w821
        i -> [w943]
        stop <- w947 stop-if-true
        # "stop"
        n579 = global write "Robot Global Data.vi" "In pos"(TRUE ("In pos")) -> ()
        n580 = global write "Robot Global Data.vi" "in ctl num"(i16 2 ("retainer num")) -> ()
        n581 = global write "Robot Global Data.vi" "retainer num"(i16 2 ("retainer num")) -> ()
        n582 = global write "Robot Global Data.vi" "Arm Control"(1.0 ("retainer num")) -> ()
        n583 = global write "Robot Global Data.vi" "1-X"(0.0 ("1-X")) -> ()
        n584 = Greater?(x=w943, y=17) -> (0:w947:bool)
        n585 = global write "Robot Global Data.vi" "1-Y"(0.0 ("1-X")) -> ()
        n586 = Wait (ms)(milliseconds to wait=u32 20) -> ()  [unwired: 1 out]
      }
      n587 = while {
        tunnel: w821 -> [w987]
        tunnel: [w987] -> w824
        stop <- w983 stop-if-true
        # "-23"
        # "218"
        # "thru the low bar"
        n588 = global read "Robot Global Data.vi" "Distance (enc.)"() -> (w985:dbl)
        n589 = global write "Robot Global Data.vi" "1-Y"(-0.8 ("1-X")) -> ()
        n590 = global read "Robot Global Data.vi" "Yaw"() -> (w978:dbl)
        n591 = global write "Robot Global Data.vi" "Pins / Intake timing"(0.0 ("Pins / Intake timing")) -> ()
        n592 = call-poly <vilib>:"PID.vi"("output range"=cluster{"output high":dbl, "output low":dbl} {"output high"=0.8, "output low"=-0.8} ("output range 2"), "PID gains"=T7 {"proportional gain (Kc)"=0.048, "integral time (Ti, min)"=0.015, "derivative time (Td, min)"=0.0} ("PID gains 2"), "process variable"=w978, "setpoint"=-26.0) -> ("output"=w980:dbl)  [unwired: 6 in, 1 out]
        n593 = Greater?(x=w985, y=16.0) -> (0:w983:bool)
        n594 = global write "Robot Global Data.vi" "1-X"(w980) -> ()
        n595 = Wait (ms)(milliseconds to wait=u32 20) -> ()  [unwired: 1 out]
      }
      n596 = while {
        tunnel: w824 -> [w976]
        tunnel: [w976] -> w812
        stop <- w972 stop-if-true
        # "125"
        # "thru the low bar"
        n597 = global write "Robot Global Data.vi" "in ctl num"(i16 0 ("retainer num")) -> ()
        n598 = global read "Robot Global Data.vi" "Distance (enc.)"() -> (w974:dbl)
        n599 = global write "Robot Global Data.vi" "1-Y"(-1.0 ("1-X")) -> ()
        n600 = global read "Robot Global Data.vi" "Yaw"() -> (w967:dbl)
        n601 = call-poly <vilib>:"PID.vi"("output range"=cluster{"output high":dbl, "output low":dbl} {"output high"=0.8, "output low"=-0.8} ("output range 2"), "PID gains"=T7 {"proportional gain (Kc)"=0.048, "integral time (Ti, min)"=0.015, "derivative time (Td, min)"=0.0} ("PID gains 2"), "process variable"=w967, "setpoint"=4.0) -> ("output"=w969:dbl)  [unwired: 6 in, 1 out]
        n602 = Greater?(x=w974, y=135.0) -> (0:w972:bool)
        n603 = global write "Robot Global Data.vi" "1-X"(w969) -> ()
        n604 = global write "Robot Global Data.vi" "In pos"(TRUE ("In pos")) -> ()
        n605 = Wait (ms)(milliseconds to wait=u32 20) -> ()  [unwired: 1 out]
      }
      n606 = while {
        tunnel: w812 -> [w868]
        tunnel: [w868] -> w811
        stop <- w864 stop-if-true
        # "198"
        # "188"
        n607 = global write "Robot Global Data.vi" "in ctl num"(i16 0 ("retainer num")) -> ()
        n608 = global read "Robot Global Data.vi" "Distance (enc.)"() -> (w866:dbl)
        n609 = global write "Robot Global Data.vi" "retainer num"(i16 0 ("retainer num")) -> ()
        n610 = global read "Robot Global Data.vi" "Yaw"() -> (w859:dbl)
        n611 = global write "Robot Global Data.vi" "Slew"(0.2 ("1-Y")) -> ()
        n612 = Greater?(x=w866, y=194.0) -> (0:w864:bool)
        n613 = call-poly <vilib>:"PID.vi"("output range"=cluster{"output high":dbl, "output low":dbl} {"output high"=0.8, "output low"=-0.8} ("output range 2"), "PID gains"=T7 {"proportional gain (Kc)"=0.048, "integral time (Ti, min)"=0.015, "derivative time (Td, min)"=0.0} ("PID gains 2"), "process variable"=w859, "setpoint"=52.0) -> ("output"=w861:dbl)  [unwired: 6 in, 1 out]
        n614 = global write "Robot Global Data.vi" "1-Y"(-0.7 ("1-Y")) -> ()
        n615 = global write "Robot Global Data.vi" "1-X"(w861) -> ()
        n616 = Wait (ms)(milliseconds to wait=u32 20) -> ()  [unwired: 1 out]
      }
      n617 = while {
        tunnel: w811 -> [w853]
        tunnel: [w853] -> w810
        stop <- TRUE stop-if-true
        # "stop"
        n618 = global write "Robot Global Data.vi" "1-X"(0.0 ("1-X")) -> ()
        n619 = global write "Robot Global Data.vi" "1-Trigger"(FALSE ("In pos")) -> ()
        n620 = global write "Robot Global Data.vi" "1-Y"(0.0 ("1-X")) -> ()
        n621 = Wait (ms)(milliseconds to wait=u32 500) -> ()  [unwired: 1 out]
      }
      n622 = while {
        tunnel: [w1018] -> w827
        tunnel: w810 -> [w1018]
        stop <- w1020 stop-if-true
        n623 = global write "Robot Global Data.vi" "Shot Selector"(FALSE ("In pos")) -> ()
        n624 = global write "Robot Global Data.vi" "1-Button 8"(TRUE ("1-Button 8")) -> ()
        n625 = global read "Robot Global Data.vi" "4?"() -> (w1020:bool)
        n626 = Wait (ms)(milliseconds to wait=u32 20) -> ()  [unwired: 1 out]
      }
      n627 = while {
        tunnel: w827 -> [w1004]
        tunnel: [w1004] -> w828
        stop <- TRUE stop-if-true
        n628 = Wait (ms)(milliseconds to wait=u32 200) -> ()  [unwired: 1 out]
      }
      n629 = while {
        tunnel: [w1015] -> w829
        tunnel: w828 -> [w1015]
        i -> [w1013]
        stop <- w1011 stop-if-true
        n630 = global write "Robot Global Data.vi" "Shoot!"(TRUE ("1-Button 8")) -> ()
        n631 = Greater?(x=w1013, y=5) -> (0:w1011:bool)
        n632 = Wait (ms)(milliseconds to wait=u32 20) -> ()  [unwired: 1 out]
      }
      n633 = while {
        tunnel: [w1009] -> w826
        tunnel: w829 -> [w1009]
        stop <- TRUE stop-if-true
        n634 = global write "Robot Global Data.vi" "Shoot!"(FALSE ("1-Button 8")) -> ()
        n635 = Wait (ms)(milliseconds to wait=u32 500) -> ()  [unwired: 1 out]
      }
      n636 = while {
        tunnel: w826 -> [w1001]
        tunnel: [w1001] -> w819
        stop <- TRUE stop-if-true
        n637 = global write "Robot Global Data.vi" "1-Button 8"(FALSE ("1-Button 8")) -> ()
        n638 = Wait (ms)(milliseconds to wait=u32 20) -> ()  [unwired: 1 out]
      }
      n639 = while {
        tunnel: w819 -> [w935]
        tunnel: [w935] -> w820
        stop <- w937 stop-if-true
        # "13"
        n640 = global read "Robot Global Data.vi" "Yaw"() -> (w934:dbl)
        n641 = global write "Robot Global Data.vi" "1-Button 8"(FALSE ("1-Button 8")) -> ()
        n642 = Sign(1:w934) -> (0:w933:dbl)
        n643 = global read "Robot Global Data.vi" "Yaw"() -> (w940:dbl)
        n644 = Multiply(x=-0.65, y=w933) -> (x*y=w931:dbl)
        n645 = global write "Robot Global Data.vi" "retainer num"(i16 2 ("retainer num")) -> ()
        n646 = Absolute Value(x=w940) -> (abs(x)=w939:dbl)
        n647 = Less?(x=w939, y=21.0) -> (x < y?=w937:bool)
        n648 = global write "Robot Global Data.vi" "1-X"(w931) -> ()
        n649 = Wait (ms)(milliseconds to wait=u32 20) -> ()  [unwired: 1 out]
      }
      n650 = while {
        tunnel: w820 -> [w927]
        tunnel: [w927] -> w818
        stop <- w923 stop-if-true
        # "218"
        # "thru the low bar"
        n651 = global write "Robot Global Data.vi" "in ctl num"(i16 0 ("retainer num")) -> ()
        n652 = global read "Robot Global Data.vi" "Distance (enc.)"() -> (w925:dbl)
        n653 = global write "Robot Global Data.vi" "1-Y"(1.0 ("1-X")) -> ()
        n654 = global read "Robot Global Data.vi" "Yaw"() -> (w918:dbl)
        n655 = call-poly <vilib>:"PID.vi"("output range"=cluster{"output high":dbl, "output low":dbl} {"output high"=0.8, "output low"=-0.8} ("output range 2"), "PID gains"=T7 {"proportional gain (Kc)"=0.048, "integral time (Ti, min)"=0.015, "derivative time (Td, min)"=0.0} ("PID gains 2"), "process variable"=w918, "setpoint"=10.0) -> ("output"=w920:dbl)  [unwired: 6 in, 1 out]
        n656 = Less?(x=w925, y=90.0) -> (x < y?=w923:bool)
        n657 = global write "Robot Global Data.vi" "In pos"(TRUE ("In pos")) -> ()
        n658 = global write "Robot Global Data.vi" "1-X"(w920) -> ()
        n659 = Wait (ms)(milliseconds to wait=u32 20) -> ()  [unwired: 1 out]
      }
      n660 = while {
        tunnel: w818 -> [w914]
        tunnel: [w914] -> w807
        stop <- w910 stop-if-true
        # "32"
        # "thru the low bar"
        n661 = global write "Robot Global Data.vi" "in ctl num"(i16 2 ("retainer num")) -> ()
        n662 = global read "Robot Global Data.vi" "Distance (enc.)"() -> (w912:dbl)
        n663 = global write "Robot Global Data.vi" "retainer num"(i16 0 ("retainer num")) -> ()
        n664 = global write "Robot Global Data.vi" "1-Y"(0.66 ("1-X")) -> ()
        n665 = global read "Robot Global Data.vi" "Yaw"() -> (w905:dbl)
        n666 = call-poly <vilib>:"PID.vi"("output range"=cluster{"output high":dbl, "output low":dbl} {"output high"=0.8, "output low"=-0.8} ("output range 2"), "PID gains"=T7 {"proportional gain (Kc)"=0.048, "integral time (Ti, min)"=0.015, "derivative time (Td, min)"=0.0} ("PID gains 2"), "process variable"=w905, "setpoint"=5.0) -> ("output"=w907:dbl)  [unwired: 6 in, 1 out]
        n667 = Less?(x=w912, y=44.0) -> (x < y?=w910:bool)
        n668 = global write "Robot Global Data.vi" "1-Trigger"(TRUE ("In pos")) -> ()
        n669 = global write "Robot Global Data.vi" "In pos"(TRUE ("In pos")) -> ()
        n670 = global write "Robot Global Data.vi" "1-X"(w907) -> ()
        n671 = Wait (ms)(milliseconds to wait=u32 20) -> ()  [unwired: 1 out]
      }
      n672 = while {
        tunnel: w807 -> [w996]
        tunnel: [w995] -> w817
        i -> [w993]
        stop <- w994 stop-if-true
        w998 = 0.0 ("1-X")
        n673 = call <vilib>:"WPI_EncoderReset.vi"("EncoderDevRef"=w996) -> ("EncoderDevRef"=w995:T3)  [unwired: 9 in, 1 out]
        n674 = Wait (ms)(milliseconds to wait=u32 20) -> ()  [unwired: 1 out]
        n675 = global write "Robot Global Data.vi" "1-X"(w998) -> ()
        n676 = Greater?(x=w993, y=3) -> (0:w994:bool)
        n677 = global write "Robot Global Data.vi" "1-Y"(w998) -> ()
      }
      n678 = while {
        tunnel: w817 -> [w880]
        tunnel: [w880] -> w809
        stop <- w876 stop-if-true
        # "115"
        # "218"
        # "thru the low bar"
        n679 = global write "Robot Global Data.vi" "in ctl num"(i16 2 ("retainer num")) -> ()
        n680 = global read "Robot Global Data.vi" "Distance (enc.)"() -> (w878:dbl)
        n681 = global write "Robot Global Data.vi" "1-Y"(-1.0 ("1-X")) -> ()
        n682 = global read "Robot Global Data.vi" "Yaw"() -> (w871:dbl)
        n683 = call-poly <vilib>:"PID.vi"("output range"=cluster{"output high":dbl, "output low":dbl} {"output high"=0.8, "output low"=-0.8} ("output range 2"), "PID gains"=T7 {"proportional gain (Kc)"=0.048, "integral time (Ti, min)"=0.015, "derivative time (Td, min)"=0.0} ("PID gains 2"), "process variable"=w871, "setpoint"=2.0) -> ("output"=w873:dbl)  [unwired: 6 in, 1 out]
        n684 = Greater?(x=w878, y=110.0) -> (0:w876:bool)
        n685 = global write "Robot Global Data.vi" "In pos"(TRUE ("In pos")) -> ()
        n686 = global write "Robot Global Data.vi" "1-X"(w873) -> ()
        n687 = Wait (ms)(milliseconds to wait=u32 20) -> ()  [unwired: 1 out]
      }
      n688 = while {
        tunnel: w809 -> [w848]
        tunnel: [w848] -> w806
        stop <- w844 stop-if-true
        # "175"
        # "thru the low bar"
        n689 = global read "Robot Global Data.vi" "Distance (enc.)"() -> (w846:dbl)
        n690 = global write "Robot Global Data.vi" "1-Y"(-0.7 ("1-X")) -> ()
        n691 = global read "Robot Global Data.vi" "Yaw"() -> (w839:dbl)
        n692 = call-poly <vilib>:"PID.vi"("output range"=cluster{"output high":dbl, "output low":dbl} {"output high"=0.8, "output low"=-0.8} ("output range 2"), "PID gains"=T7 {"proportional gain (Kc)"=0.048, "integral time (Ti, min)"=0.015, "derivative time (Td, min)"=0.0} ("PID gains 2"), "process variable"=w839, "setpoint"=52.0) -> ("output"=w841:dbl)  [unwired: 6 in, 1 out]
        n693 = Greater?(x=w846, y=183.0) -> (0:w844:bool)
        n694 = global write "Robot Global Data.vi" "1-X"(w841) -> ()
        n695 = global write "Robot Global Data.vi" "In pos"(TRUE ("In pos")) -> ()
        n696 = Wait (ms)(milliseconds to wait=u32 20) -> ()  [unwired: 1 out]
      }
      n697 = while {
        tunnel: w806 -> [w835]
        tunnel: [w835] -> w808
        stop <- TRUE stop-if-true
        # "stop"
        n698 = global write "Robot Global Data.vi" "in ctl num"(i16 0 ("retainer num")) -> ()
        n699 = global write "Robot Global Data.vi" "1-X"(0.0 ("1-X")) -> ()
        n700 = global write "Robot Global Data.vi" "1-Trigger"(FALSE ("In pos")) -> ()
        n701 = global write "Robot Global Data.vi" "1-Y"(0.0 ("1-X")) -> ()
        n702 = Wait (ms)(milliseconds to wait=u32 400) -> ()  [unwired: 1 out]
      }
      n703 = while {
        tunnel: [w898] -> w816
        tunnel: w808 -> [w898]
        stop <- w900 stop-if-true
        n704 = global write "Robot Global Data.vi" "Shot Selector"(FALSE ("In pos")) -> ()
        n705 = global write "Robot Global Data.vi" "1-Button 8"(TRUE ("1-Button 8")) -> ()
        n706 = global read "Robot Global Data.vi" "4?"() -> (w900:bool)
        n707 = Wait (ms)(milliseconds to wait=u32 20) -> ()  [unwired: 1 out]
      }
      n708 = while {
        tunnel: w816 -> [w884]
        tunnel: [w884] -> w814
        stop <- TRUE stop-if-true
        n709 = global write "Robot Global Data.vi" "1-Button 8"(FALSE ("1-Button 8")) -> ()
        n710 = Wait (ms)(milliseconds to wait=u32 250) -> ()  [unwired: 1 out]
      }
      n711 = while {
        tunnel: [w895] -> w815
        tunnel: w814 -> [w895]
        i -> [w893]
        stop <- w891 stop-if-true
        n712 = global write "Robot Global Data.vi" "Shoot!"(TRUE ("1-Button 8")) -> ()
        n713 = Greater?(x=w893, y=5) -> (0:w891:bool)
        n714 = Wait (ms)(milliseconds to wait=u32 20) -> ()  [unwired: 1 out]
      }
      n715 = while {
        tunnel: [w889] -> w813
        tunnel: w815 -> [w889]
        stop <- TRUE stop-if-true
        n716 = global write "Robot Global Data.vi" "Shoot!"(FALSE ("1-Button 8")) -> ()
        n717 = Wait (ms)(milliseconds to wait=u32 700) -> ()  [unwired: 1 out]
      }
      n718 = while {
        tunnel: w813 -> [w991]
        tunnel: [w991] -> w825
        stop <- FALSE stop-if-true
        w989 = 0.0 ("1-X")
        n719 = global write "Robot Global Data.vi" "1-X"(w989) -> ()
        n720 = global write "Robot Global Data.vi" "1-Y"(w989) -> ()
      }
    }
    frame 13 {
      # "OLD 2 BALL"
      # "APPRX GOAL"
      # "and STOP"
      # "DO IT AGAIN"
      # "PICK UP"
      # "COME BACK"
      # "TURN TO 0"
      # "FIRE"
      # "AIM"
      # "SICK DROPS"
      # "S CURVE"
      # "APPRX GOAL"
      # "DISRGARD ALL COMMENTS NOT IN CAPS"
      # "2 BALL?"
      n721 = while {
        tunnel: w1043 -> [w1229]
        tunnel: [w1229] -> w1042
        i -> [w1222]
        stop <- w1226 stop-if-true
        # "stop"
        n722 = global write "Robot Global Data.vi" "Arm Control"(-1.0 ("retainer num")) -> ()
        n723 = global write "Robot Global Data.vi" "In pos"(TRUE ("In pos")) -> ()
        n724 = global write "Robot Global Data.vi" "in ctl num"(i16 2 ("retainer num")) -> ()
        n725 = global write "Robot Global Data.vi" "1-Trigger"(TRUE ("In pos")) -> ()
        n726 = global write "Robot Global Data.vi" "retainer num"(i16 2 ("retainer num")) -> ()
        n727 = global write "Robot Global Data.vi" "1-X"(0.0 ("1-X")) -> ()
        n728 = Greater?(x=w1222, y=15) -> (0:w1226:bool)
        n729 = global write "Robot Global Data.vi" "1-Y"(0.0 ("1-X")) -> ()
        n730 = Wait (ms)(milliseconds to wait=u32 20) -> ()  [unwired: 1 out]
      }
      n731 = while {
        tunnel: w1042 -> [w1217]
        tunnel: [w1217] -> w1041
        i -> [w1210]
        stop <- w1214 stop-if-true
        # "stop"
        n732 = global write "Robot Global Data.vi" "In pos"(TRUE ("In pos")) -> ()
        n733 = global write "Robot Global Data.vi" "in ctl num"(i16 2 ("retainer num")) -> ()
        n734 = global write "Robot Global Data.vi" "retainer num"(i16 2 ("retainer num")) -> ()
        n735 = global write "Robot Global Data.vi" "Arm Control"(1.0 ("retainer num")) -> ()
        n736 = global write "Robot Global Data.vi" "1-X"(0.0 ("1-X")) -> ()
        n737 = Greater?(x=w1210, y=17) -> (0:w1214:bool)
        n738 = global write "Robot Global Data.vi" "1-Y"(0.0 ("1-X")) -> ()
        n739 = Wait (ms)(milliseconds to wait=u32 20) -> ()  [unwired: 1 out]
      }
      n740 = while {
        tunnel: w1041 -> [w1255]
        tunnel: [w1255] -> w1044
        stop <- w1251 stop-if-true
        # "-26"
        # "218"
        # "thru the low bar"
        n741 = global read "Robot Global Data.vi" "Distance (enc.)"() -> (w1253:dbl)
        n742 = global write "Robot Global Data.vi" "1-Y"(-0.8 ("1-X")) -> ()
        n743 = global read "Robot Global Data.vi" "Yaw"() -> (w1246:dbl)
        n744 = global write "Robot Global Data.vi" "Pins / Intake timing"(0.0 ("Pins / Intake timing")) -> ()
        n745 = call-poly <vilib>:"PID.vi"("output range"=cluster{"output high":dbl, "output low":dbl} {"output high"=0.8, "output low"=-0.8} ("output range 2"), "PID gains"=T7 {"proportional gain (Kc)"=0.048, "integral time (Ti, min)"=0.015, "derivative time (Td, min)"=0.0} ("PID gains 2"), "process variable"=w1246, "setpoint"=-24.0) -> ("output"=w1248:dbl)  [unwired: 6 in, 1 out]
        n746 = Greater?(x=w1253, y=16.0) -> (0:w1251:bool)
        n747 = global write "Robot Global Data.vi" "1-X"(w1248) -> ()
        n748 = Wait (ms)(milliseconds to wait=u32 20) -> ()  [unwired: 1 out]
      }
      n749 = while {
        tunnel: w1044 -> [w1244]
        tunnel: [w1244] -> w1029
        stop <- w1240 stop-if-true
        # "125"
        # "thru the low bar"
        n750 = global write "Robot Global Data.vi" "in ctl num"(i16 0 ("retainer num")) -> ()
        n751 = global read "Robot Global Data.vi" "Distance (enc.)"() -> (w1242:dbl)
        n752 = global write "Robot Global Data.vi" "1-Y"(-1.0 ("1-X")) -> ()
        n753 = global read "Robot Global Data.vi" "Yaw"() -> (w1235:dbl)
        n754 = call-poly <vilib>:"PID.vi"("output range"=cluster{"output high":dbl, "output low":dbl} {"output high"=0.8, "output low"=-0.8} ("output range 2"), "PID gains"=T7 {"proportional gain (Kc)"=0.048, "integral time (Ti, min)"=0.015, "derivative time (Td, min)"=0.0} ("PID gains 2"), "process variable"=w1235, "setpoint"=4.0) -> ("output"=w1237:dbl)  [unwired: 6 in, 1 out]
        n755 = Greater?(x=w1242, y=100.0) -> (0:w1240:bool)
        n756 = global write "Robot Global Data.vi" "1-X"(w1237) -> ()
        n757 = global write "Robot Global Data.vi" "Slew"(0.2 ("1-Y")) -> ()
        n758 = global write "Robot Global Data.vi" "In pos"(TRUE ("In pos")) -> ()
        n759 = Wait (ms)(milliseconds to wait=u32 20) -> ()  [unwired: 1 out]
      }
      n760 = while {
        tunnel: w1029 -> [w1114]
        tunnel: [w1114] -> w1028
        stop <- w1110 stop-if-true
        # "125"
        # "thru the low bar"
        n761 = global write "Robot Global Data.vi" "in ctl num"(i16 0 ("retainer num")) -> ()
        n762 = global read "Robot Global Data.vi" "Distance (enc.)"() -> (w1112:dbl)
        n763 = global write "Robot Global Data.vi" "1-Y"(-1.0 ("1-X")) -> ()
        n764 = global read "Robot Global Data.vi" "Yaw"() -> (w1105:dbl)
        n765 = call-poly <vilib>:"PID.vi"("output range"=cluster{"output high":dbl, "output low":dbl} {"output high"=0.8, "output low"=-0.8} ("output range 2"), "PID gains"=T7 {"proportional gain (Kc)"=0.048, "integral time (Ti, min)"=0.015, "derivative time (Td, min)"=0.0} ("PID gains 2"), "process variable"=w1105, "setpoint"=4.0) -> ("output"=w1107:dbl)  [unwired: 6 in, 1 out]
        n766 = Greater?(x=w1112, y=175.0) -> (0:w1110:bool)
        n767 = global write "Robot Global Data.vi" "1-X"(w1107) -> ()
        n768 = global write "Robot Global Data.vi" "Slew"(0.04 ("1-Y")) -> ()
        n769 = global write "Robot Global Data.vi" "In pos"(TRUE ("In pos")) -> ()
        n770 = Wait (ms)(milliseconds to wait=u32 20) -> ()  [unwired: 1 out]
      }
      n771 = while {
        tunnel: w1028 -> [w1136]
        tunnel: [w1136] -> w1033
        stop <- w1132 stop-if-true
        # "20"
        n772 = global write "Robot Global Data.vi" "in ctl num"(i16 0 ("retainer num")) -> ()
        n773 = global write "Robot Global Data.vi" "Slew"(0.2 ("1-Y")) -> ()
        n774 = global read "Robot Global Data.vi" "Yaw"() -> (w1134:dbl)
        n775 = global write "Robot Global Data.vi" "retainer num"(i16 0 ("retainer num")) -> ()
        n776 = global write "Robot Global Data.vi" "1-Trigger"(FALSE ("In pos")) -> ()
        n777 = Greater?(x=w1134, y=24.0) -> (0:w1132:bool)
        n778 = global write "Robot Global Data.vi" "1-Y"(0.0 ("1-Y")) -> ()
        n779 = global write "Robot Global Data.vi" "1-X"(0.8 ("1-X")) -> ()
        n780 = Wait (ms)(milliseconds to wait=u32 20) -> ()  [unwired: 1 out]
      }
      n781 = while {
        tunnel: w1033 -> [w1124]
        tunnel: [w1124] -> w1031
        stop <- TRUE stop-if-true
        # "stop"
        n782 = global write "Robot Global Data.vi" "1-X"(0.0 ("1-X")) -> ()
        n783 = global write "Robot Global Data.vi" "1-Y"(0.0 ("1-X")) -> ()
        n784 = Wait (ms)(milliseconds to wait=u32 500) -> ()  [unwired: 1 out]
      }
      n785 = while {
        tunnel: w1031 -> [w1119]
        tunnel: [w1119] -> w1030
        stop <- TRUE stop-if-true
        # "stop"
        n786 = global write "Robot Global Data.vi" "1-X"(0.0 ("1-X")) -> ()
        n787 = global write "Robot Global Data.vi" "Slew"(0.2 ("1-Y")) -> ()
        n788 = global write "Robot Global Data.vi" "1-Y"(0.0 ("1-X")) -> ()
        n789 = Wait (ms)(milliseconds to wait=u32 20) -> ()  [unwired: 1 out]
      }
      n790 = while {
        tunnel: [w1286] -> w1047
        tunnel: w1030 -> [w1286]
        stop <- w1288 stop-if-true
        n791 = global write "Robot Global Data.vi" "Shot Selector"(FALSE ("In pos")) -> ()
        n792 = global write "Robot Global Data.vi" "1-Button 8"(TRUE ("1-Button 8")) -> ()
        n793 = global read "Robot Global Data.vi" "4?"() -> (w1288:bool)
        n794 = Wait (ms)(milliseconds to wait=u32 20) -> ()  [unwired: 1 out]
      }
      n795 = while {
        tunnel: w1047 -> [w1272]
        tunnel: [w1272] -> w1048
        stop <- TRUE stop-if-true
        n796 = Wait (ms)(milliseconds to wait=u32 200) -> ()  [unwired: 1 out]
      }
      n797 = while {
        tunnel: [w1283] -> w1049
        tunnel: w1048 -> [w1283]
        i -> [w1281]
        stop <- w1279 stop-if-true
        n798 = global write "Robot Global Data.vi" "Shoot!"(TRUE ("1-Button 8")) -> ()
        n799 = Greater?(x=w1281, y=5) -> (0:w1279:bool)
        n800 = Wait (ms)(milliseconds to wait=u32 20) -> ()  [unwired: 1 out]
      }
      n801 = while {
        tunnel: [w1277] -> w1046
        tunnel: w1049 -> [w1277]
        stop <- TRUE stop-if-true
        n802 = global write "Robot Global Data.vi" "Shoot!"(FALSE ("1-Button 8")) -> ()
        n803 = Wait (ms)(milliseconds to wait=u32 500) -> ()  [unwired: 1 out]
      }
      n804 = while {
        tunnel: w1046 -> [w1269]
        tunnel: [w1269] -> w1040
        stop <- TRUE stop-if-true
        n805 = global write "Robot Global Data.vi" "1-Button 8"(FALSE ("1-Button 8")) -> ()
        n806 = Wait (ms)(milliseconds to wait=u32 20) -> ()  [unwired: 1 out]
      }
      n807 = while {
        tunnel: w1040 -> [w1202]
        tunnel: [w1202] -> w1022
        stop <- w1204 stop-if-true
        # "13"
        n808 = global read "Robot Global Data.vi" "Yaw"() -> (w1201:dbl)
        n809 = global write "Robot Global Data.vi" "1-Button 8"(FALSE ("1-Button 8")) -> ()
        n810 = Sign(1:w1201) -> (0:w1200:dbl)
        n811 = global read "Robot Global Data.vi" "Yaw"() -> (w1207:dbl)
        n812 = Multiply(x=-0.65, y=w1200) -> (x*y=w1198:dbl)
        n813 = global write "Robot Global Data.vi" "retainer num"(i16 2 ("retainer num")) -> ()
        n814 = Absolute Value(x=w1207) -> (abs(x)=w1206:dbl)
        n815 = Less?(x=w1206, y=20.0) -> (x < y?=w1204:bool)
        n816 = global write "Robot Global Data.vi" "1-X"(w1198) -> ()
        n817 = Wait (ms)(milliseconds to wait=u32 20) -> ()  [unwired: 1 out]
      }
      n818 = while {
        tunnel: w1022 -> [w1063]
        tunnel: [w1063] -> w1021
        stop <- w1059 stop-if-true
        # "218"
        # "thru the low bar"
        n819 = global write "Robot Global Data.vi" "in ctl num"(i16 0 ("retainer num")) -> ()
        n820 = global read "Robot Global Data.vi" "Distance (enc.)"() -> (w1061:dbl)
        n821 = global write "Robot Global Data.vi" "Slew"(0.04 ("Slew")) -> ()
        n822 = global write "Robot Global Data.vi" "1-Y"(1.0 ("1-X")) -> ()
        n823 = global read "Robot Global Data.vi" "Yaw"() -> (w1054:dbl)
        n824 = call-poly <vilib>:"PID.vi"("output range"=cluster{"output high":dbl, "output low":dbl} {"output high"=0.8, "output low"=-0.8} ("output range 2"), "PID gains"=T7 {"proportional gain (Kc)"=0.048, "integral time (Ti, min)"=0.015, "derivative time (Td, min)"=0.0} ("PID gains 2"), "process variable"=w1054, "setpoint"=2.0) -> ("output"=w1056:dbl)  [unwired: 6 in, 1 out]
        n825 = Less?(x=w1061, y=165.0) -> (x < y?=w1059:bool)
        n826 = global write "Robot Global Data.vi" "1-Trigger"(TRUE ("In pos")) -> ()
        n827 = global write "Robot Global Data.vi" "In pos"(TRUE ("In pos")) -> ()
        n828 = global write "Robot Global Data.vi" "1-X"(w1056) -> ()
        n829 = Wait (ms)(milliseconds to wait=u32 20) -> ()  [unwired: 1 out]
      }
      n830 = while {
        tunnel: w1021 -> [w1194]
        tunnel: [w1194] -> w1039
        stop <- w1190 stop-if-true
        # "218"
        # "thru the low bar"
        n831 = global write "Robot Global Data.vi" "in ctl num"(i16 0 ("retainer num")) -> ()
        n832 = global read "Robot Global Data.vi" "Distance (enc.)"() -> (w1192:dbl)
        n833 = global write "Robot Global Data.vi" "Slew"(0.2 ("Slew")) -> ()
        n834 = global write "Robot Global Data.vi" "1-Y"(0.6 ("1-X")) -> ()
        n835 = global read "Robot Global Data.vi" "Yaw"() -> (w1185:dbl)
        n836 = call-poly <vilib>:"PID.vi"("output range"=cluster{"output high":dbl, "output low":dbl} {"output high"=0.8, "output low"=-0.8} ("output range 2"), "PID gains"=T7 {"proportional gain (Kc)"=0.048, "integral time (Ti, min)"=0.015, "derivative time (Td, min)"=0.0} ("PID gains 2"), "process variable"=w1185, "setpoint"=3.0) -> ("output"=w1187:dbl)  [unwired: 6 in, 1 out]
        n837 = Less?(x=w1192, y=115.0) -> (x < y?=w1190:bool)
        n838 = global write "Robot Global Data.vi" "In pos"(TRUE ("In pos")) -> ()
        n839 = global write "Robot Global Data.vi" "1-X"(w1187) -> ()
        n840 = Wait (ms)(milliseconds to wait=u32 20) -> ()  [unwired: 1 out]
      }
      n841 = while {
        tunnel: w1039 -> [w1180]
        tunnel: [w1180] -> w1032
        stop <- w1176 stop-if-true
        # "4"
        # "32"
        # "thru the low bar"
        n842 = global write "Robot Global Data.vi" "in ctl num"(i16 2 ("retainer num")) -> ()
        n843 = global read "Robot Global Data.vi" "Distance (enc.)"() -> (w1178:dbl)
        n844 = global write "Robot Global Data.vi" "1-Y"(0.8 ("1-X")) -> ()
        n845 = global read "Robot Global Data.vi" "Yaw"() -> (w1171:dbl)
        n846 = call-poly <vilib>:"PID.vi"("output range"=cluster{"output high":dbl, "output low":dbl} {"output high"=0.8, "output low"=-0.8} ("output range 2"), "PID gains"=T7 {"proportional gain (Kc)"=0.048, "integral time (Ti, min)"=0.015, "derivative time (Td, min)"=0.0} ("PID gains 2"), "process variable"=w1171, "setpoint"=5.0) -> ("output"=w1173:dbl)  [unwired: 6 in, 1 out]
        n847 = Less?(x=w1178, y=44.0) -> (x < y?=w1176:bool)
        n848 = global write "Robot Global Data.vi" "In pos"(TRUE ("In pos")) -> ()
        n849 = global write "Robot Global Data.vi" "1-X"(w1173) -> ()
        n850 = Wait (ms)(milliseconds to wait=u32 20) -> ()  [unwired: 1 out]
      }
      n851 = while {
        tunnel: w1032 -> [w1264]
        tunnel: [w1263] -> w1038
        i -> [w1261]
        stop <- w1262 stop-if-true
        w1266 = 0.0 ("1-X")
        n852 = call <vilib>:"WPI_EncoderReset.vi"("EncoderDevRef"=w1264) -> ("EncoderDevRef"=w1263:T3)  [unwired: 9 in, 1 out]
        n853 = Wait (ms)(milliseconds to wait=u32 20) -> ()  [unwired: 1 out]
        n854 = global write "Robot Global Data.vi" "1-X"(w1266) -> ()
        n855 = Greater?(x=w1261, y=3) -> (0:w1262:bool)
        n856 = global write "Robot Global Data.vi" "1-Y"(w1266) -> ()
      }
      n857 = while {
        tunnel: w1038 -> [w1148]
        tunnel: [w1148] -> w1024
        stop <- w1144 stop-if-true
        # "115"
        # "218"
        # "thru the low bar"
        n858 = global write "Robot Global Data.vi" "in ctl num"(i16 2 ("retainer num")) -> ()
        n859 = global read "Robot Global Data.vi" "Distance (enc.)"() -> (w1146:dbl)
        n860 = global write "Robot Global Data.vi" "1-Y"(-1.0 ("1-X")) -> ()
        n861 = global read "Robot Global Data.vi" "Yaw"() -> (w1139:dbl)
        n862 = call-poly <vilib>:"PID.vi"("output range"=cluster{"output high":dbl, "output low":dbl} {"output high"=0.8, "output low"=-0.8} ("output range 2"), "PID gains"=T7 {"proportional gain (Kc)"=0.048, "integral time (Ti, min)"=0.015, "derivative time (Td, min)"=0.0} ("PID gains 2"), "process variable"=w1139, "setpoint"=4.0) -> ("output"=w1141:dbl)  [unwired: 6 in, 1 out]
        n863 = Greater?(x=w1146, y=90.0) -> (0:w1144:bool)
        n864 = global write "Robot Global Data.vi" "In pos"(TRUE ("In pos")) -> ()
        n865 = global write "Robot Global Data.vi" "1-X"(w1141) -> ()
        n866 = Wait (ms)(milliseconds to wait=u32 20) -> ()  [unwired: 1 out]
      }
      n867 = while {
        tunnel: w1024 -> [w1078]
        tunnel: [w1078] -> w1025
        stop <- w1074 stop-if-true
        # "125"
        # "thru the low bar"
        n868 = global write "Robot Global Data.vi" "in ctl num"(i16 0 ("retainer num")) -> ()
        n869 = global read "Robot Global Data.vi" "Distance (enc.)"() -> (w1076:dbl)
        n870 = global write "Robot Global Data.vi" "1-Y"(-1.0 ("1-X")) -> ()
        n871 = global read "Robot Global Data.vi" "Yaw"() -> (w1069:dbl)
        n872 = call-poly <vilib>:"PID.vi"("output range"=cluster{"output high":dbl, "output low":dbl} {"output high"=0.8, "output low"=-0.8} ("output range 2"), "PID gains"=T7 {"proportional gain (Kc)"=0.048, "integral time (Ti, min)"=0.015, "derivative time (Td, min)"=0.0} ("PID gains 2"), "process variable"=w1069, "setpoint"=6.0) -> ("output"=w1071:dbl)  [unwired: 6 in, 1 out]
        n873 = Greater?(x=w1076, y=175.0) -> (0:w1074:bool)
        n874 = global write "Robot Global Data.vi" "1-X"(w1071) -> ()
        n875 = global write "Robot Global Data.vi" "Slew"(0.04 ("1-Y")) -> ()
        n876 = global write "Robot Global Data.vi" "In pos"(TRUE ("In pos")) -> ()
        n877 = Wait (ms)(milliseconds to wait=u32 20) -> ()  [unwired: 1 out]
      }
      n878 = while {
        tunnel: w1025 -> [w1100]
        tunnel: [w1100] -> w1027
        stop <- w1096 stop-if-true
        # "25"
        n879 = global write "Robot Global Data.vi" "in ctl num"(i16 0 ("retainer num")) -> ()
        n880 = global write "Robot Global Data.vi" "Slew"(0.2 ("1-Y")) -> ()
        n881 = global read "Robot Global Data.vi" "Yaw"() -> (w1098:dbl)
        n882 = global write "Robot Global Data.vi" "retainer num"(i16 0 ("retainer num")) -> ()
        n883 = global write "Robot Global Data.vi" "1-Trigger"(FALSE ("In pos")) -> ()
        n884 = Greater?(x=w1098, y=24.0) -> (0:w1096:bool)
        n885 = global write "Robot Global Data.vi" "1-Y"(0.0 ("1-Y")) -> ()
        n886 = global write "Robot Global Data.vi" "1-X"(0.8 ("1-X")) -> ()
        n887 = Wait (ms)(milliseconds to wait=u32 20) -> ()  [unwired: 1 out]
      }
      n888 = while {
        tunnel: w1027 -> [w1088]
        tunnel: [w1088] -> w1026
        stop <- TRUE stop-if-true
        # "stop"
        n889 = global write "Robot Global Data.vi" "1-X"(0.0 ("1-X")) -> ()
        n890 = global write "Robot Global Data.vi" "1-Y"(0.0 ("1-X")) -> ()
        n891 = Wait (ms)(milliseconds to wait=u32 500) -> ()  [unwired: 1 out]
      }
      n892 = while {
        tunnel: w1026 -> [w1083]
        tunnel: [w1083] -> w1023
        stop <- TRUE stop-if-true
        # "stop"
        n893 = global write "Robot Global Data.vi" "1-X"(0.0 ("1-X")) -> ()
        n894 = global write "Robot Global Data.vi" "Slew"(0.2 ("1-Y")) -> ()
        n895 = global write "Robot Global Data.vi" "1-Y"(0.0 ("1-X")) -> ()
        n896 = Wait (ms)(milliseconds to wait=u32 20) -> ()  [unwired: 1 out]
      }
      n897 = while {
        tunnel: [w1166] -> w1037
        tunnel: w1023 -> [w1166]
        stop <- w1168 stop-if-true
        n898 = global write "Robot Global Data.vi" "Shot Selector"(FALSE ("In pos")) -> ()
        n899 = global write "Robot Global Data.vi" "1-Button 8"(TRUE ("1-Button 8")) -> ()
        n900 = global read "Robot Global Data.vi" "4?"() -> (w1168:bool)
        n901 = Wait (ms)(milliseconds to wait=u32 20) -> ()  [unwired: 1 out]
      }
      n902 = while {
        tunnel: w1037 -> [w1152]
        tunnel: [w1152] -> w1035
        stop <- TRUE stop-if-true
        n903 = global write "Robot Global Data.vi" "1-Button 8"(FALSE ("1-Button 8")) -> ()
        n904 = Wait (ms)(milliseconds to wait=u32 250) -> ()  [unwired: 1 out]
      }
      n905 = while {
        tunnel: [w1163] -> w1036
        tunnel: w1035 -> [w1163]
        i -> [w1161]
        stop <- w1159 stop-if-true
        n906 = global write "Robot Global Data.vi" "Shoot!"(TRUE ("1-Button 8")) -> ()
        n907 = Greater?(x=w1161, y=5) -> (0:w1159:bool)
        n908 = Wait (ms)(milliseconds to wait=u32 20) -> ()  [unwired: 1 out]
      }
      n909 = while {
        tunnel: [w1157] -> w1034
        tunnel: w1036 -> [w1157]
        stop <- TRUE stop-if-true
        n910 = global write "Robot Global Data.vi" "Shoot!"(FALSE ("1-Button 8")) -> ()
        n911 = Wait (ms)(milliseconds to wait=u32 700) -> ()  [unwired: 1 out]
      }
      n912 = while {
        tunnel: w1034 -> [w1259]
        tunnel: [w1259] -> w1045
        stop <- FALSE stop-if-true
        w1257 = 0.0 ("1-X")
        n913 = global write "Robot Global Data.vi" "1-X"(w1257) -> ()
        n914 = global write "Robot Global Data.vi" "1-Y"(w1257) -> ()
      }
    }
    frame 14 {
      # "OLD 2 BALL"
      # "APPRX GOAL"
      # "and STOP"
      # "DO IT AGAIN"
      # "PICK UP"
      # "COME BACK"
      # "TURN TO 0"
      # "FIRE"
      # "AIM"
      # "SICK DROPS"
      # "S CURVE"
      # "APPRX GOAL"
      # "DISRGARD ALL COMMENTS NOT IN CAPS"
      # "2 BALL?"
      n915 = while {
        tunnel: w1309 -> [w1484]
        tunnel: [w1484] -> w1308
        i -> [w1477]
        stop <- w1481 stop-if-true
        # "stop"
        n916 = global write "Robot Global Data.vi" "Arm Control"(-1.0 ("retainer num")) -> ()
        n917 = global write "Robot Global Data.vi" "In pos"(TRUE ("In pos")) -> ()
        n918 = global write "Robot Global Data.vi" "in ctl num"(i16 2 ("retainer num")) -> ()
        n919 = global write "Robot Global Data.vi" "1-Trigger"(TRUE ("In pos")) -> ()
        n920 = global write "Robot Global Data.vi" "retainer num"(i16 2 ("retainer num")) -> ()
        n921 = global write "Robot Global Data.vi" "1-X"(0.0 ("1-X")) -> ()
        n922 = Greater?(x=w1477, y=15) -> (0:w1481:bool)
        n923 = global write "Robot Global Data.vi" "1-Y"(0.0 ("1-X")) -> ()
        n924 = Wait (ms)(milliseconds to wait=u32 20) -> ()  [unwired: 1 out]
      }
      n925 = while {
        tunnel: w1308 -> [w1472]
        tunnel: [w1472] -> w1307
        i -> [w1465]
        stop <- w1469 stop-if-true
        # "stop"
        n926 = global write "Robot Global Data.vi" "In pos"(TRUE ("In pos")) -> ()
        n927 = global write "Robot Global Data.vi" "in ctl num"(i16 2 ("retainer num")) -> ()
        n928 = global write "Robot Global Data.vi" "retainer num"(i16 2 ("retainer num")) -> ()
        n929 = global write "Robot Global Data.vi" "Arm Control"(1.0 ("retainer num")) -> ()
        n930 = global write "Robot Global Data.vi" "1-X"(0.0 ("1-X")) -> ()
        n931 = Greater?(x=w1465, y=17) -> (0:w1469:bool)
        n932 = global write "Robot Global Data.vi" "1-Y"(0.0 ("1-X")) -> ()
        n933 = Wait (ms)(milliseconds to wait=u32 20) -> ()  [unwired: 1 out]
      }
      n934 = while {
        tunnel: w1307 -> [w1510]
        tunnel: [w1510] -> w1310
        stop <- w1506 stop-if-true
        # "-26"
        # "218"
        # "thru the low bar"
        n935 = global read "Robot Global Data.vi" "Distance (enc.)"() -> (w1508:dbl)
        n936 = global write "Robot Global Data.vi" "1-Y"(-0.8 ("1-X")) -> ()
        n937 = global read "Robot Global Data.vi" "Yaw"() -> (w1501:dbl)
        n938 = global write "Robot Global Data.vi" "Pins / Intake timing"(0.0 ("Pins / Intake timing")) -> ()
        n939 = call-poly <vilib>:"PID.vi"("output range"=cluster{"output high":dbl, "output low":dbl} {"output high"=0.8, "output low"=-0.8} ("output range 2"), "PID gains"=T7 {"proportional gain (Kc)"=0.048, "integral time (Ti, min)"=0.015, "derivative time (Td, min)"=0.0} ("PID gains 2"), "process variable"=w1501, "setpoint"=-26.0) -> ("output"=w1503:dbl)  [unwired: 6 in, 1 out]
        n940 = Greater?(x=w1508, y=16.0) -> (0:w1506:bool)
        n941 = global write "Robot Global Data.vi" "1-X"(w1503) -> ()
        n942 = Wait (ms)(milliseconds to wait=u32 20) -> ()  [unwired: 1 out]
      }
      n943 = while {
        tunnel: w1310 -> [w1499]
        tunnel: [w1499] -> w1297
        stop <- w1495 stop-if-true
        # "125"
        # "thru the low bar"
        n944 = global write "Robot Global Data.vi" "in ctl num"(i16 0 ("retainer num")) -> ()
        n945 = global read "Robot Global Data.vi" "Distance (enc.)"() -> (w1497:dbl)
        n946 = global write "Robot Global Data.vi" "1-Y"(-1.0 ("1-X")) -> ()
        n947 = global read "Robot Global Data.vi" "Yaw"() -> (w1490:dbl)
        n948 = call-poly <vilib>:"PID.vi"("output range"=cluster{"output high":dbl, "output low":dbl} {"output high"=0.8, "output low"=-0.8} ("output range 2"), "PID gains"=T7 {"proportional gain (Kc)"=0.048, "integral time (Ti, min)"=0.015, "derivative time (Td, min)"=0.0} ("PID gains 2"), "process variable"=w1490, "setpoint"=4.0) -> ("output"=w1492:dbl)  [unwired: 6 in, 1 out]
        n949 = Greater?(x=w1497, y=100.0) -> (0:w1495:bool)
        n950 = global write "Robot Global Data.vi" "1-X"(w1492) -> ()
        n951 = global write "Robot Global Data.vi" "Slew"(0.2 ("1-Y")) -> ()
        n952 = global write "Robot Global Data.vi" "In pos"(TRUE ("In pos")) -> ()
        n953 = Wait (ms)(milliseconds to wait=u32 20) -> ()  [unwired: 1 out]
      }
      n954 = while {
        tunnel: w1297 -> [w1375]
        tunnel: [w1375] -> w1296
        stop <- w1371 stop-if-true
        # "125"
        # "thru the low bar"
        n955 = global write "Robot Global Data.vi" "in ctl num"(i16 0 ("retainer num")) -> ()
        n956 = global read "Robot Global Data.vi" "Distance (enc.)"() -> (w1373:dbl)
        n957 = global write "Robot Global Data.vi" "1-Y"(-1.0 ("1-X")) -> ()
        n958 = global read "Robot Global Data.vi" "Yaw"() -> (w1366:dbl)
        n959 = call-poly <vilib>:"PID.vi"("output range"=cluster{"output high":dbl, "output low":dbl} {"output high"=0.8, "output low"=-0.8} ("output range 2"), "PID gains"=T7 {"proportional gain (Kc)"=0.048, "integral time (Ti, min)"=0.015, "derivative time (Td, min)"=0.0} ("PID gains 2"), "process variable"=w1366, "setpoint"=4.0) -> ("output"=w1368:dbl)  [unwired: 6 in, 1 out]
        n960 = Greater?(x=w1373, y=185.0) -> (0:w1371:bool)
        n961 = global write "Robot Global Data.vi" "1-X"(w1368) -> ()
        n962 = global write "Robot Global Data.vi" "Slew"(0.04 ("1-Y")) -> ()
        n963 = global write "Robot Global Data.vi" "In pos"(TRUE ("In pos")) -> ()
        n964 = Wait (ms)(milliseconds to wait=u32 20) -> ()  [unwired: 1 out]
      }
      n965 = while {
        tunnel: w1296 -> [w1391]
        tunnel: [w1391] -> w1299
        stop <- w1387 stop-if-true
        # ".8"
        # "28"
        n966 = global write "Robot Global Data.vi" "in ctl num"(i16 0 ("retainer num")) -> ()
        n967 = global write "Robot Global Data.vi" "Slew"(0.2 ("1-Y")) -> ()
        n968 = global read "Robot Global Data.vi" "Yaw"() -> (w1389:dbl)
        n969 = global write "Robot Global Data.vi" "retainer num"(i16 0 ("retainer num")) -> ()
        n970 = global write "Robot Global Data.vi" "1-Trigger"(FALSE ("In pos")) -> ()
        n971 = Greater?(x=w1389, y=16.0) -> (0:w1387:bool)
        n972 = global write "Robot Global Data.vi" "1-Y"(0.0 ("1-Y")) -> ()
        n973 = global write "Robot Global Data.vi" "1-X"(0.8 ("1-X")) -> ()
        n974 = Wait (ms)(milliseconds to wait=u32 20) -> ()  [unwired: 1 out]
      }
      n975 = while {
        tunnel: w1299 -> [w1379]
        tunnel: [w1379] -> w1290
        stop <- TRUE stop-if-true
        # "stop"
        n976 = global write "Robot Global Data.vi" "1-X"(0.0 ("1-X")) -> ()
        n977 = global write "Robot Global Data.vi" "1-Y"(0.0 ("1-X")) -> ()
        n978 = Wait (ms)(milliseconds to wait=u32 700) -> ()  [unwired: 1 out]
      }
      n979 = while {
        tunnel: [w1542] -> w1313
        tunnel: w1290 -> [w1542]
        stop <- w1544 stop-if-true
        n980 = global write "Robot Global Data.vi" "Shot Selector"(FALSE ("In pos")) -> ()
        n981 = global write "Robot Global Data.vi" "1-Button 8"(TRUE ("1-Button 8")) -> ()
        n982 = global read "Robot Global Data.vi" "4?"() -> (w1544:bool)
        n983 = Wait (ms)(milliseconds to wait=u32 20) -> ()  [unwired: 1 out]
      }
      n984 = while {
        tunnel: w1313 -> [w1528]
        tunnel: [w1528] -> w1314
        stop <- TRUE stop-if-true
        # "200"
        n985 = Wait (ms)(milliseconds to wait=u32 450) -> ()  [unwired: 1 out]
      }
      n986 = while {
        tunnel: [w1539] -> w1315
        tunnel: w1314 -> [w1539]
        i -> [w1537]
        stop <- w1535 stop-if-true
        n987 = global write "Robot Global Data.vi" "Shoot!"(TRUE ("1-Button 8")) -> ()
        n988 = Greater?(x=w1537, y=5) -> (0:w1535:bool)
        n989 = Wait (ms)(milliseconds to wait=u32 20) -> ()  [unwired: 1 out]
      }
      n990 = while {
        tunnel: [w1533] -> w1312
        tunnel: w1315 -> [w1533]
        stop <- TRUE stop-if-true
        n991 = global write "Robot Global Data.vi" "Shoot!"(FALSE ("1-Button 8")) -> ()
        n992 = Wait (ms)(milliseconds to wait=u32 500) -> ()  [unwired: 1 out]
      }
      n993 = while {
        tunnel: w1312 -> [w1525]
        tunnel: [w1525] -> w1306
        stop <- TRUE stop-if-true
        n994 = global write "Robot Global Data.vi" "1-Button 8"(FALSE ("1-Button 8")) -> ()
        n995 = Wait (ms)(milliseconds to wait=u32 20) -> ()  [unwired: 1 out]
      }
      n996 = while {
        tunnel: w1306 -> [w1457]
        tunnel: [w1457] -> w1292
        stop <- w1459 stop-if-true
        # "13"
        n997 = global read "Robot Global Data.vi" "Yaw"() -> (w1456:dbl)
        n998 = global write "Robot Global Data.vi" "1-Button 8"(FALSE ("1-Button 8")) -> ()
        n999 = Sign(1:w1456) -> (0:w1455:dbl)
        n1000 = global read "Robot Global Data.vi" "Yaw"() -> (w1462:dbl)
        n1001 = Multiply(x=-0.65, y=w1455) -> (x*y=w1453:dbl)
        n1002 = global write "Robot Global Data.vi" "retainer num"(i16 2 ("retainer num")) -> ()
        n1003 = Absolute Value(x=w1462) -> (abs(x)=w1461:dbl)
        n1004 = Less?(x=w1461, y=19.0) -> (x < y?=w1459:bool)
        n1005 = global write "Robot Global Data.vi" "1-X"(w1453) -> ()
        n1006 = Wait (ms)(milliseconds to wait=u32 20) -> ()  [unwired: 1 out]
      }
      n1007 = while {
        tunnel: w1292 -> [w1329]
        tunnel: [w1329] -> w1291
        stop <- w1325 stop-if-true
        # "218"
        # "thru the low bar"
        n1008 = global write "Robot Global Data.vi" "in ctl num"(i16 0 ("retainer num")) -> ()
        n1009 = global read "Robot Global Data.vi" "Distance (enc.)"() -> (w1327:dbl)
        n1010 = global write "Robot Global Data.vi" "Slew"(0.04 ("Slew")) -> ()
        n1011 = global write "Robot Global Data.vi" "1-Y"(1.0 ("1-X")) -> ()
        n1012 = global read "Robot Global Data.vi" "Yaw"() -> (w1320:dbl)
        n1013 = call-poly <vilib>:"PID.vi"("output range"=cluster{"output high":dbl, "output low":dbl} {"output high"=0.8, "output low"=-0.8} ("output range 2"), "PID gains"=T7 {"proportional gain (Kc)"=0.048, "integral time (Ti, min)"=0.015, "derivative time (Td, min)"=0.0} ("PID gains 2"), "process variable"=w1320, "setpoint"=2.0) -> ("output"=w1322:dbl)  [unwired: 6 in, 1 out]
        n1014 = Less?(x=w1327, y=165.0) -> (x < y?=w1325:bool)
        n1015 = global write "Robot Global Data.vi" "1-Trigger"(TRUE ("In pos")) -> ()
        n1016 = global write "Robot Global Data.vi" "In pos"(TRUE ("In pos")) -> ()
        n1017 = global write "Robot Global Data.vi" "1-X"(w1322) -> ()
        n1018 = Wait (ms)(milliseconds to wait=u32 20) -> ()  [unwired: 1 out]
      }
      n1019 = while {
        tunnel: w1291 -> [w1449]
        tunnel: [w1449] -> w1305
        stop <- w1445 stop-if-true
        # "218"
        # "thru the low bar"
        n1020 = global write "Robot Global Data.vi" "in ctl num"(i16 0 ("retainer num")) -> ()
        n1021 = global read "Robot Global Data.vi" "Distance (enc.)"() -> (w1447:dbl)
        n1022 = global write "Robot Global Data.vi" "Slew"(0.2 ("Slew")) -> ()
        n1023 = global write "Robot Global Data.vi" "1-Y"(0.6 ("1-X")) -> ()
        n1024 = global read "Robot Global Data.vi" "Yaw"() -> (w1440:dbl)
        n1025 = call-poly <vilib>:"PID.vi"("output range"=cluster{"output high":dbl, "output low":dbl} {"output high"=0.8, "output low"=-0.8} ("output range 2"), "PID gains"=T7 {"proportional gain (Kc)"=0.048, "integral time (Ti, min)"=0.015, "derivative time (Td, min)"=0.0} ("PID gains 2"), "process variable"=w1440, "setpoint"=3.0) -> ("output"=w1442:dbl)  [unwired: 6 in, 1 out]
        n1026 = Less?(x=w1447, y=115.0) -> (x < y?=w1445:bool)
        n1027 = global write "Robot Global Data.vi" "In pos"(TRUE ("In pos")) -> ()
        n1028 = global write "Robot Global Data.vi" "1-X"(w1442) -> ()
        n1029 = Wait (ms)(milliseconds to wait=u32 20) -> ()  [unwired: 1 out]
      }
      n1030 = while {
        tunnel: w1305 -> [w1435]
        tunnel: [w1435] -> w1298
        stop <- w1431 stop-if-true
        # "4"
        # "44"
        # "thru the low bar"
        n1031 = global write "Robot Global Data.vi" "in ctl num"(i16 2 ("retainer num")) -> ()
        n1032 = global read "Robot Global Data.vi" "Distance (enc.)"() -> (w1433:dbl)
        n1033 = global write "Robot Global Data.vi" "1-Y"(0.8 ("1-X")) -> ()
        n1034 = global read "Robot Global Data.vi" "Yaw"() -> (w1426:dbl)
        n1035 = call-poly <vilib>:"PID.vi"("output range"=cluster{"output high":dbl, "output low":dbl} {"output high"=0.8, "output low"=-0.8} ("output range 2"), "PID gains"=T7 {"proportional gain (Kc)"=0.048, "integral time (Ti, min)"=0.015, "derivative time (Td, min)"=0.0} ("PID gains 2"), "process variable"=w1426, "setpoint"=3.0) -> ("output"=w1428:dbl)  [unwired: 6 in, 1 out]
        n1036 = Less?(x=w1433, y=42.0) -> (x < y?=w1431:bool)
        n1037 = global write "Robot Global Data.vi" "In pos"(TRUE ("In pos")) -> ()
        n1038 = global write "Robot Global Data.vi" "1-X"(w1428) -> ()
        n1039 = Wait (ms)(milliseconds to wait=u32 20) -> ()  [unwired: 1 out]
      }
      n1040 = while {
        tunnel: w1298 -> [w1520]
        tunnel: [w1519] -> w1304
        i -> [w1517]
        stop <- w1518 stop-if-true
        w1522 = 0.0 ("1-X")
        n1041 = call <vilib>:"WPI_EncoderReset.vi"("EncoderDevRef"=w1520) -> ("EncoderDevRef"=w1519:T3)  [unwired: 9 in, 1 out]
        n1042 = Wait (ms)(milliseconds to wait=u32 20) -> ()  [unwired: 1 out]
        n1043 = global write "Robot Global Data.vi" "1-X"(w1522) -> ()
        n1044 = global write "Robot Global Data.vi" "Slew"(0.04 ("1-Y")) -> ()
        n1045 = Greater?(x=w1517, y=8) -> (0:w1518:bool)
        n1046 = global write "Robot Global Data.vi" "1-Y"(w1522) -> ()
      }
      n1047 = while {
        tunnel: w1304 -> [w1403]
        tunnel: [w1403] -> w1293
        stop <- w1399 stop-if-true
        # "115"
        # "218"
        # "thru the low bar"
        n1048 = global write "Robot Global Data.vi" "in ctl num"(i16 2 ("retainer num")) -> ()
        n1049 = global read "Robot Global Data.vi" "Distance (enc.)"() -> (w1401:dbl)
        n1050 = global write "Robot Global Data.vi" "1-Y"(-1.0 ("1-X")) -> ()
        n1051 = global read "Robot Global Data.vi" "Yaw"() -> (w1394:dbl)
        n1052 = call-poly <vilib>:"PID.vi"("output range"=cluster{"output high":dbl, "output low":dbl} {"output high"=0.8, "output low"=-0.8} ("output range 2"), "PID gains"=T7 {"proportional gain (Kc)"=0.048, "integral time (Ti, min)"=0.015, "derivative time (Td, min)"=0.0} ("PID gains 2"), "process variable"=w1394, "setpoint"=-0.5) -> ("output"=w1396:dbl)  [unwired: 6 in, 1 out]
        n1053 = Greater?(x=w1401, y=90.0) -> (0:w1399:bool)
        n1054 = global write "Robot Global Data.vi" "In pos"(TRUE ("In pos")) -> ()
        n1055 = global write "Robot Global Data.vi" "1-X"(w1396) -> ()
        n1056 = Wait (ms)(milliseconds to wait=u32 20) -> ()  [unwired: 1 out]
      }
      n1057 = while {
        tunnel: w1293 -> [w1345]
        tunnel: [w1345] -> w1294
        stop <- w1341 stop-if-true
        # "125"
        # "thru the low bar"
        n1058 = global write "Robot Global Data.vi" "in ctl num"(i16 0 ("retainer num")) -> ()
        n1059 = global read "Robot Global Data.vi" "Distance (enc.)"() -> (w1343:dbl)
        n1060 = global write "Robot Global Data.vi" "Slew"(0.2 ("1-Y")) -> ()
        n1061 = global write "Robot Global Data.vi" "1-Y"(-1.0 ("1-X")) -> ()
        n1062 = global read "Robot Global Data.vi" "Yaw"() -> (w1336:dbl)
        n1063 = call-poly <vilib>:"PID.vi"("output range"=cluster{"output high":dbl, "output low":dbl} {"output high"=0.8, "output low"=-0.8} ("output range 2"), "PID gains"=T7 {"proportional gain (Kc)"=0.048, "integral time (Ti, min)"=0.015, "derivative time (Td, min)"=0.0} ("PID gains 2"), "process variable"=w1336, "setpoint"=5.0) -> ("output"=w1338:dbl)  [unwired: 6 in, 1 out]
        n1064 = Greater?(x=w1343, y=175.0) -> (0:w1341:bool)
        n1065 = global write "Robot Global Data.vi" "1-X"(w1338) -> ()
        n1066 = global write "Robot Global Data.vi" "Slew"(0.04 ("1-Y")) -> ()
        n1067 = global write "Robot Global Data.vi" "In pos"(TRUE ("In pos")) -> ()
        n1068 = Wait (ms)(milliseconds to wait=u32 20) -> ()  [unwired: 1 out]
      }
      n1069 = while {
        tunnel: w1294 -> [w1361]
        tunnel: [w1361] -> w1295
        stop <- w1357 stop-if-true
        # "24"
        n1070 = global write "Robot Global Data.vi" "in ctl num"(i16 0 ("retainer num")) -> ()
        n1071 = global write "Robot Global Data.vi" "Slew"(0.2 ("1-Y")) -> ()
        n1072 = global read "Robot Global Data.vi" "Yaw"() -> (w1359:dbl)
        n1073 = global write "Robot Global Data.vi" "retainer num"(i16 0 ("retainer num")) -> ()
        n1074 = global write "Robot Global Data.vi" "1-Trigger"(FALSE ("In pos")) -> ()
        n1075 = Greater?(x=w1359, y=16.0) -> (0:w1357:bool)
        n1076 = global write "Robot Global Data.vi" "1-Y"(0.0 ("1-Y")) -> ()
        n1077 = global write "Robot Global Data.vi" "1-X"(0.8 ("1-X")) -> ()
        n1078 = Wait (ms)(milliseconds to wait=u32 20) -> ()  [unwired: 1 out]
      }
      n1079 = while {
        tunnel: w1295 -> [w1349]
        tunnel: [w1349] -> w1289
        stop <- TRUE stop-if-true
        # "stop"
        n1080 = global write "Robot Global Data.vi" "1-X"(0.0 ("1-X")) -> ()
        n1081 = global write "Robot Global Data.vi" "1-Y"(0.0 ("1-X")) -> ()
        n1082 = Wait (ms)(milliseconds to wait=u32 700) -> ()  [unwired: 1 out]
      }
      n1083 = while {
        tunnel: [w1421] -> w1303
        tunnel: w1289 -> [w1421]
        stop <- w1423 stop-if-true
        n1084 = global write "Robot Global Data.vi" "Shot Selector"(FALSE ("In pos")) -> ()
        n1085 = global write "Robot Global Data.vi" "1-Button 8"(TRUE ("1-Button 8")) -> ()
        n1086 = global read "Robot Global Data.vi" "4?"() -> (w1423:bool)
        n1087 = Wait (ms)(milliseconds to wait=u32 20) -> ()  [unwired: 1 out]
      }
      n1088 = while {
        tunnel: w1303 -> [w1407]
        tunnel: [w1407] -> w1301
        stop <- TRUE stop-if-true
        n1089 = global write "Robot Global Data.vi" "1-Button 8"(FALSE ("1-Button 8")) -> ()
        n1090 = Wait (ms)(milliseconds to wait=u32 450) -> ()  [unwired: 1 out]
      }
      n1091 = while {
        tunnel: [w1418] -> w1302
        tunnel: w1301 -> [w1418]
        i -> [w1416]
        stop <- w1414 stop-if-true
        n1092 = global write "Robot Global Data.vi" "Shoot!"(TRUE ("1-Button 8")) -> ()
        n1093 = Greater?(x=w1416, y=5) -> (0:w1414:bool)
        n1094 = Wait (ms)(milliseconds to wait=u32 20) -> ()  [unwired: 1 out]
      }
      n1095 = while {
        tunnel: [w1412] -> w1300
        tunnel: w1302 -> [w1412]
        stop <- TRUE stop-if-true
        n1096 = global write "Robot Global Data.vi" "Shoot!"(FALSE ("1-Button 8")) -> ()
        n1097 = Wait (ms)(milliseconds to wait=u32 700) -> ()  [unwired: 1 out]
      }
      n1098 = while {
        tunnel: w1300 -> [w1514]
        tunnel: [w1514] -> w1311
        stop <- FALSE stop-if-true
        w1512 = 0.0 ("1-X")
        n1099 = global write "Robot Global Data.vi" "1-X"(w1512) -> ()
        n1100 = global write "Robot Global Data.vi" "1-Y"(w1512) -> ()
      }
    }
    frame 16 {
      # "OLD 2 BALL"
      # "?"
      # "3 STAGE DECELERATION AND LOW GEAR"
      # "LAST THING JACOB DID ON 4/20"
      # "APPRX GOAL"
      # "and STOP"
      # "DO IT AGAIN"
      # "PICK UP"
      # "COME BACK"
      # "TURN TO 0"
      # "FIRE"
      # "AIM"
      # "SICK DROPS"
      # "S CURVE"
      # "APPRX GOAL"
      # "DISRGARD ALL COMMENTS NOT IN CAPS"
      # "2 BALL?"
      n1101 = while {
        tunnel: w1568 -> [w1767]
        tunnel: [w1767] -> w1567
        i -> [w1760]
        stop <- w1764 stop-if-true
        # "stop"
        n1102 = global write "Robot Global Data.vi" "Arm Control"(-1.0 ("retainer num")) -> ()
        n1103 = global write "Robot Global Data.vi" "In pos"(TRUE ("In pos")) -> ()
        n1104 = global write "Robot Global Data.vi" "in ctl num"(i16 2 ("retainer num")) -> ()
        n1105 = global write "Robot Global Data.vi" "1-Trigger"(TRUE ("In pos")) -> ()
        n1106 = global write "Robot Global Data.vi" "retainer num"(i16 2 ("retainer num")) -> ()
        n1107 = global write "Robot Global Data.vi" "1-X"(0.0 ("1-X")) -> ()
        n1108 = Greater?(x=w1760, y=15) -> (0:w1764:bool)
        n1109 = global write "Robot Global Data.vi" "1-Y"(0.0 ("1-X")) -> ()
        n1110 = Wait (ms)(milliseconds to wait=u32 20) -> ()  [unwired: 1 out]
      }
      n1111 = while {
        tunnel: w1567 -> [w1755]
        tunnel: [w1755] -> w1566
        i -> [w1748]
        stop <- w1752 stop-if-true
        # "stop"
        n1112 = global write "Robot Global Data.vi" "In pos"(TRUE ("In pos")) -> ()
        n1113 = global write "Robot Global Data.vi" "in ctl num"(i16 2 ("retainer num")) -> ()
        n1114 = global write "Robot Global Data.vi" "retainer num"(i16 2 ("retainer num")) -> ()
        n1115 = global write "Robot Global Data.vi" "Arm Control"(1.0 ("retainer num")) -> ()
        n1116 = global write "Robot Global Data.vi" "1-X"(0.0 ("1-X")) -> ()
        n1117 = Greater?(x=w1748, y=17) -> (0:w1752:bool)
        n1118 = global write "Robot Global Data.vi" "1-Y"(0.0 ("1-X")) -> ()
        n1119 = Wait (ms)(milliseconds to wait=u32 20) -> ()  [unwired: 1 out]
      }
      n1120 = while {
        tunnel: w1566 -> [w1793]
        tunnel: [w1793] -> w1569
        stop <- w1789 stop-if-true
        # "-23"
        # "218"
        # "thru the low bar"
        n1121 = global read "Robot Global Data.vi" "Distance (enc.)"() -> (w1791:dbl)
        n1122 = global write "Robot Global Data.vi" "1-Y"(-0.8 ("1-X")) -> ()
        n1123 = global read "Robot Global Data.vi" "Yaw"() -> (w1784:dbl)
        n1124 = global write "Robot Global Data.vi" "Pins / Intake timing"(0.0 ("Pins / Intake timing")) -> ()
        n1125 = call-poly <vilib>:"PID.vi"("output range"=cluster{"output high":dbl, "output low":dbl} {"output high"=0.8, "output low"=-0.8} ("output range 2"), "PID gains"=T7 {"proportional gain (Kc)"=0.048, "integral time (Ti, min)"=0.015, "derivative time (Td, min)"=0.0} ("PID gains 2"), "process variable"=w1784, "setpoint"=-26.0) -> ("output"=w1786:dbl)  [unwired: 6 in, 1 out]
        n1126 = Greater?(x=w1791, y=16.0) -> (0:w1789:bool)
        n1127 = global write "Robot Global Data.vi" "1-X"(w1786) -> ()
        n1128 = Wait (ms)(milliseconds to wait=u32 20) -> ()  [unwired: 1 out]
      }
      n1129 = while {
        tunnel: w1569 -> [w1782]
        tunnel: [w1782] -> w1554
        stop <- w1778 stop-if-true
        # "125"
        # "thru the low bar"
        n1130 = global write "Robot Global Data.vi" "in ctl num"(i16 0 ("retainer num")) -> ()
        n1131 = global read "Robot Global Data.vi" "Distance (enc.)"() -> (w1780:dbl)
        n1132 = global write "Robot Global Data.vi" "1-Y"(-1.0 ("1-X")) -> ()
        n1133 = global read "Robot Global Data.vi" "Yaw"() -> (w1773:dbl)
        n1134 = call-poly <vilib>:"PID.vi"("output range"=cluster{"output high":dbl, "output low":dbl} {"output high"=0.8, "output low"=-0.8} ("output range 2"), "PID gains"=T7 {"proportional gain (Kc)"=0.048, "integral time (Ti, min)"=0.015, "derivative time (Td, min)"=0.0} ("PID gains 2"), "process variable"=w1773, "setpoint"=4.0) -> ("output"=w1775:dbl)  [unwired: 6 in, 1 out]
        n1135 = Greater?(x=w1780, y=100.0) -> (0:w1778:bool)
        n1136 = global write "Robot Global Data.vi" "1-X"(w1775) -> ()
        n1137 = global write "Robot Global Data.vi" "Slew"(0.2 ("1-Y")) -> ()
        n1138 = global write "Robot Global Data.vi" "In pos"(TRUE ("In pos")) -> ()
        n1139 = Wait (ms)(milliseconds to wait=u32 20) -> ()  [unwired: 1 out]
      }
      n1140 = while {
        tunnel: w1554 -> [w1654]
        tunnel: [w1654] -> w1548
        stop <- w1650 stop-if-true
        # "125"
        # "thru the low bar"
        n1141 = global write "Robot Global Data.vi" "in ctl num"(i16 0 ("retainer num")) -> ()
        n1142 = global read "Robot Global Data.vi" "Distance (enc.)"() -> (w1652:dbl)
        n1143 = global write "Robot Global Data.vi" "1-Y"(-1.0 ("1-X")) -> ()
        n1144 = global read "Robot Global Data.vi" "Yaw"() -> (w1645:dbl)
        n1145 = call-poly <vilib>:"PID.vi"("output range"=cluster{"output high":dbl, "output low":dbl} {"output high"=0.8, "output low"=-0.8} ("output range 2"), "PID gains"=T7 {"proportional gain (Kc)"=0.048, "integral time (Ti, min)"=0.015, "derivative time (Td, min)"=0.0} ("PID gains 2"), "process variable"=w1645, "setpoint"=4.0) -> ("output"=w1647:dbl)  [unwired: 6 in, 1 out]
        n1146 = Greater?(x=w1652, y=165.0) -> (0:w1650:bool)
        n1147 = global write "Robot Global Data.vi" "1-X"(w1647) -> ()
        n1148 = global write "Robot Global Data.vi" "Slew"(0.2 ("1-Y")) -> ()
        n1149 = global write "Robot Global Data.vi" "In pos"(TRUE ("In pos")) -> ()
        n1150 = Wait (ms)(milliseconds to wait=u32 20) -> ()  [unwired: 1 out]
      }
      n1151 = while {
        tunnel: w1548 -> [w1604]
        tunnel: [w1604] -> w1547
        stop <- w1600 stop-if-true
        # "125"
        # "thru the low bar"
        n1152 = global write "Robot Global Data.vi" "in ctl num"(i16 0 ("retainer num")) -> ()
        n1153 = global read "Robot Global Data.vi" "Distance (enc.)"() -> (w1602:dbl)
        n1154 = global write "Robot Global Data.vi" "1-Trigger"(FALSE ("In pos")) -> ()
        n1155 = global write "Robot Global Data.vi" "1-Y"(-0.65 ("1-X")) -> ()
        n1156 = global read "Robot Global Data.vi" "Yaw"() -> (w1595:dbl)
        n1157 = call-poly <vilib>:"PID.vi"("output range"=cluster{"output high":dbl, "output low":dbl} {"output high"=0.8, "output low"=-0.8} ("output range 2"), "PID gains"=T7 {"proportional gain (Kc)"=0.048, "integral time (Ti, min)"=0.015, "derivative time (Td, min)"=0.0} ("PID gains 2"), "process variable"=w1595, "setpoint"=4.0) -> ("output"=w1597:dbl)  [unwired: 6 in, 1 out]
        n1158 = Greater?(x=w1602, y=180.0) -> (0:w1600:bool)
        n1159 = global write "Robot Global Data.vi" "1-X"(w1597) -> ()
        n1160 = global write "Robot Global Data.vi" "Slew"(0.2 ("1-Y")) -> ()
        n1161 = global write "Robot Global Data.vi" "In pos"(TRUE ("In pos")) -> ()
        n1162 = Wait (ms)(milliseconds to wait=u32 20) -> ()  [unwired: 1 out]
      }
      n1163 = while {
        tunnel: w1547 -> [w1589]
        tunnel: [w1589] -> w1546
        stop <- w1585 stop-if-true
        # "125"
        # "thru the low bar"
        n1164 = global write "Robot Global Data.vi" "in ctl num"(i16 0 ("retainer num")) -> ()
        n1165 = global read "Robot Global Data.vi" "Distance (enc.)"() -> (w1587:dbl)
        n1166 = global write "Robot Global Data.vi" "1-Trigger"(FALSE ("In pos")) -> ()
        n1167 = global write "Robot Global Data.vi" "1-Y"(-0.55 ("1-X")) -> ()
        n1168 = global read "Robot Global Data.vi" "Yaw"() -> (w1580:dbl)
        n1169 = call-poly <vilib>:"PID.vi"("output range"=cluster{"output high":dbl, "output low":dbl} {"output high"=0.8, "output low"=-0.8} ("output range 2"), "PID gains"=T7 {"proportional gain (Kc)"=0.048, "integral time (Ti, min)"=0.015, "derivative time (Td, min)"=0.0} ("PID gains 2"), "process variable"=w1580, "setpoint"=4.0) -> ("output"=w1582:dbl)  [unwired: 6 in, 1 out]
        n1170 = Greater?(x=w1587, y=190.0) -> (0:w1585:bool)
        n1171 = global write "Robot Global Data.vi" "1-X"(w1582) -> ()
        n1172 = global write "Robot Global Data.vi" "Slew"(0.2 ("1-Y")) -> ()
        n1173 = global write "Robot Global Data.vi" "In pos"(TRUE ("In pos")) -> ()
        n1174 = Wait (ms)(milliseconds to wait=u32 20) -> ()  [unwired: 1 out]
      }
      n1175 = while {
        tunnel: w1546 -> [w1666]
        tunnel: [w1666] -> w1558
        stop <- w1672 stop-if-true
        # "35"
        n1176 = global write "Robot Global Data.vi" "in ctl num"(i16 0 ("retainer num")) -> ()
        n1177 = global write "Robot Global Data.vi" "Slew"(0.2 ("1-Y")) -> ()
        n1178 = global read "Robot Global Data.vi" "Yaw"() -> (w1674:dbl)
        n1179 = global write "Robot Global Data.vi" "retainer num"(i16 0 ("retainer num")) -> ()
        n1180 = Greater?(x=w1674, y=19.0) -> (0:w1672:bool)
        n1181 = global write "Robot Global Data.vi" "1-Y"(0.0 ("1-Y")) -> ()
        n1182 = global write "Robot Global Data.vi" "1-X"(0.8 ("1-X")) -> ()
        n1183 = Wait (ms)(milliseconds to wait=u32 20) -> ()  [unwired: 1 out]
      }
      n1184 = while {
        tunnel: w1558 -> [w1664]
        tunnel: [w1664] -> w1556
        stop <- TRUE stop-if-true
        # "stop"
        n1185 = global write "Robot Global Data.vi" "1-X"(0.0 ("1-X")) -> ()
        n1186 = global write "Robot Global Data.vi" "1-Y"(0.0 ("1-X")) -> ()
        n1187 = Wait (ms)(milliseconds to wait=u32 600) -> ()  [unwired: 1 out]
      }
      n1188 = while {
        tunnel: w1556 -> [w1659]
        tunnel: [w1659] -> w1555
        stop <- TRUE stop-if-true
        # "stop"
        n1189 = global write "Robot Global Data.vi" "1-X"(0.0 ("1-X")) -> ()
        n1190 = global write "Robot Global Data.vi" "Slew"(0.2 ("1-Y")) -> ()
        n1191 = global write "Robot Global Data.vi" "1-Y"(0.0 ("1-X")) -> ()
        n1192 = Wait (ms)(milliseconds to wait=u32 20) -> ()  [unwired: 1 out]
      }
      n1193 = while {
        tunnel: [w1824] -> w1572
        tunnel: w1555 -> [w1824]
        stop <- w1826 stop-if-true
        n1194 = global write "Robot Global Data.vi" "Shot Selector"(FALSE ("In pos")) -> ()
        n1195 = global write "Robot Global Data.vi" "1-Button 8"(TRUE ("1-Button 8")) -> ()
        n1196 = global read "Robot Global Data.vi" "4?"() -> (w1826:bool)
        n1197 = Wait (ms)(milliseconds to wait=u32 20) -> ()  [unwired: 1 out]
      }
      n1198 = while {
        tunnel: w1572 -> [w1810]
        tunnel: [w1810] -> w1573
        stop <- TRUE stop-if-true
        n1199 = Wait (ms)(milliseconds to wait=u32 200) -> ()  [unwired: 1 out]
      }
      n1200 = while {
        tunnel: [w1821] -> w1574
        tunnel: w1573 -> [w1821]
        i -> [w1819]
        stop <- w1817 stop-if-true
        n1201 = global write "Robot Global Data.vi" "Shoot!"(TRUE ("1-Button 8")) -> ()
        n1202 = Greater?(x=w1819, y=5) -> (0:w1817:bool)
        n1203 = Wait (ms)(milliseconds to wait=u32 20) -> ()  [unwired: 1 out]
      }
      n1204 = while {
        tunnel: [w1815] -> w1571
        tunnel: w1574 -> [w1815]
        stop <- TRUE stop-if-true
        n1205 = global write "Robot Global Data.vi" "Shoot!"(FALSE ("1-Button 8")) -> ()
        n1206 = Wait (ms)(milliseconds to wait=u32 500) -> ()  [unwired: 1 out]
      }
      n1207 = while {
        tunnel: w1571 -> [w1807]
        tunnel: [w1807] -> w1564
        stop <- TRUE stop-if-true
        n1208 = global write "Robot Global Data.vi" "1-Button 8"(FALSE ("1-Button 8")) -> ()
        n1209 = Wait (ms)(milliseconds to wait=u32 20) -> ()  [unwired: 1 out]
      }
      n1210 = while {
        tunnel: w1564 -> [w1740]
        tunnel: [w1740] -> w1565
        stop <- w1742 stop-if-true
        # "13"
        n1211 = global read "Robot Global Data.vi" "Yaw"() -> (w1739:dbl)
        n1212 = global write "Robot Global Data.vi" "1-Button 8"(FALSE ("1-Button 8")) -> ()
        n1213 = Sign(1:w1739) -> (0:w1738:dbl)
        n1214 = global read "Robot Global Data.vi" "Yaw"() -> (w1745:dbl)
        n1215 = Multiply(x=-0.65, y=w1738) -> (x*y=w1736:dbl)
        n1216 = global write "Robot Global Data.vi" "retainer num"(i16 2 ("retainer num")) -> ()
        n1217 = Absolute Value(x=w1745) -> (abs(x)=w1744:dbl)
        n1218 = Less?(x=w1744, y=21.0) -> (x < y?=w1742:bool)
        n1219 = global write "Robot Global Data.vi" "1-X"(w1736) -> ()
        n1220 = Wait (ms)(milliseconds to wait=u32 20) -> ()  [unwired: 1 out]
      }
      n1221 = while {
        tunnel: w1565 -> [w1732]
        tunnel: [w1732] -> w1563
        stop <- w1728 stop-if-true
        # "218"
        # "thru the low bar"
        n1222 = global write "Robot Global Data.vi" "in ctl num"(i16 0 ("retainer num")) -> ()
        n1223 = global read "Robot Global Data.vi" "Distance (enc.)"() -> (w1730:dbl)
        n1224 = global write "Robot Global Data.vi" "1-Y"(1.0 ("1-X")) -> ()
        n1225 = global read "Robot Global Data.vi" "Yaw"() -> (w1723:dbl)
        n1226 = call-poly <vilib>:"PID.vi"("output range"=cluster{"output high":dbl, "output low":dbl} {"output high"=0.8, "output low"=-0.8} ("output range 2"), "PID gains"=T7 {"proportional gain (Kc)"=0.048, "integral time (Ti, min)"=0.015, "derivative time (Td, min)"=0.0} ("PID gains 2"), "process variable"=w1723, "setpoint"=4.0) -> ("output"=w1725:dbl)  [unwired: 6 in, 1 out]
        n1227 = Less?(x=w1730, y=90.0) -> (x < y?=w1728:bool)
        n1228 = global write "Robot Global Data.vi" "In pos"(TRUE ("In pos")) -> ()
        n1229 = global write "Robot Global Data.vi" "1-X"(w1725) -> ()
        n1230 = Wait (ms)(milliseconds to wait=u32 20) -> ()  [unwired: 1 out]
      }
      n1231 = while {
        tunnel: w1563 -> [w1719]
        tunnel: [w1719] -> w1557
        stop <- w1715 stop-if-true
        # "32"
        # "thru the low bar"
        n1232 = global write "Robot Global Data.vi" "in ctl num"(i16 2 ("retainer num")) -> ()
        n1233 = global read "Robot Global Data.vi" "Distance (enc.)"() -> (w1717:dbl)
        n1234 = global write "Robot Global Data.vi" "1-Y"(0.66 ("1-X")) -> ()
        n1235 = global read "Robot Global Data.vi" "Yaw"() -> (w1710:dbl)
        n1236 = call-poly <vilib>:"PID.vi"("output range"=cluster{"output high":dbl, "output low":dbl} {"output high"=0.8, "output low"=-0.8} ("output range 2"), "PID gains"=T7 {"proportional gain (Kc)"=0.048, "integral time (Ti, min)"=0.015, "derivative time (Td, min)"=0.0} ("PID gains 2"), "process variable"=w1710, "setpoint"=2.0) -> ("output"=w1712:dbl)  [unwired: 6 in, 1 out]
        n1237 = Less?(x=w1717, y=42.0) -> (x < y?=w1715:bool)
        n1238 = global write "Robot Global Data.vi" "1-Trigger"(TRUE ("In pos")) -> ()
        n1239 = global write "Robot Global Data.vi" "In pos"(TRUE ("In pos")) -> ()
        n1240 = global write "Robot Global Data.vi" "1-X"(w1712) -> ()
        n1241 = Wait (ms)(milliseconds to wait=u32 20) -> ()  [unwired: 1 out]
      }
      n1242 = while {
        tunnel: w1557 -> [w1802]
        tunnel: [w1801] -> w1545
        i -> [w1799]
        stop <- w1800 stop-if-true
        w1804 = 0.0 ("1-X")
        n1243 = call <vilib>:"WPI_EncoderReset.vi"("EncoderDevRef"=w1802) -> ("EncoderDevRef"=w1801:T3)  [unwired: 9 in, 1 out]
        n1244 = Wait (ms)(milliseconds to wait=u32 20) -> ()  [unwired: 1 out]
        n1245 = global write "Robot Global Data.vi" "1-X"(w1804) -> ()
        n1246 = Greater?(x=w1799, y=10) -> (0:w1800:bool)
        n1247 = global write "Robot Global Data.vi" "1-Y"(w1804) -> ()
      }
      n1248 = while {
        tunnel: w1545 -> [w1687]
        tunnel: [w1687] -> w1550
        stop <- w1683 stop-if-true
        # "115"
        # "218"
        # "thru the low bar"
        n1249 = global write "Robot Global Data.vi" "in ctl num"(i16 2 ("retainer num")) -> ()
        n1250 = global read "Robot Global Data.vi" "Distance (enc.)"() -> (w1685:dbl)
        n1251 = global write "Robot Global Data.vi" "1-Y"(-0.9 ("1-X")) -> ()
        n1252 = global read "Robot Global Data.vi" "Yaw"() -> (w1678:dbl)
        n1253 = call-poly <vilib>:"PID.vi"("output range"=cluster{"output high":dbl, "output low":dbl} {"output high"=0.8, "output low"=-0.8} ("output range 2"), "PID gains"=T7 {"proportional gain (Kc)"=0.048, "integral time (Ti, min)"=0.015, "derivative time (Td, min)"=0.0} ("PID gains 2"), "process variable"=w1678, "setpoint"=-1.0) -> ("output"=w1680:dbl)  [unwired: 6 in, 1 out]
        n1254 = Greater?(x=w1685, y=70.0) -> (0:w1683:bool)
        n1255 = global write "Robot Global Data.vi" "In pos"(TRUE ("In pos")) -> ()
        n1256 = global write "Robot Global Data.vi" "1-X"(w1680) -> ()
        n1257 = Wait (ms)(milliseconds to wait=u32 20) -> ()  [unwired: 1 out]
      }
      n1258 = while {
        tunnel: w1550 -> [w1618]
        tunnel: [w1618] -> w1551
        stop <- w1614 stop-if-true
        # "125"
        # "thru the low bar"
        n1259 = global write "Robot Global Data.vi" "in ctl num"(i16 0 ("retainer num")) -> ()
        n1260 = global read "Robot Global Data.vi" "Distance (enc.)"() -> (w1616:dbl)
        n1261 = global write "Robot Global Data.vi" "1-Y"(-1.0 ("1-X")) -> ()
        n1262 = global read "Robot Global Data.vi" "Yaw"() -> (w1609:dbl)
        n1263 = call-poly <vilib>:"PID.vi"("output range"=cluster{"output high":dbl, "output low":dbl} {"output high"=0.8, "output low"=-0.8} ("output range 2"), "PID gains"=T7 {"proportional gain (Kc)"=0.048, "integral time (Ti, min)"=0.015, "derivative time (Td, min)"=0.0} ("PID gains 2"), "process variable"=w1609, "setpoint"=4.0) -> ("output"=w1611:dbl)  [unwired: 6 in, 1 out]
        n1264 = Greater?(x=w1616, y=175.0) -> (0:w1614:bool)
        n1265 = global write "Robot Global Data.vi" "1-X"(w1611) -> ()
        n1266 = global write "Robot Global Data.vi" "Slew"(0.04 ("1-Y")) -> ()
        n1267 = global write "Robot Global Data.vi" "In pos"(TRUE ("In pos")) -> ()
        n1268 = Wait (ms)(milliseconds to wait=u32 20) -> ()  [unwired: 1 out]
      }
      n1269 = while {
        tunnel: w1551 -> [w1640]
        tunnel: [w1640] -> w1553
        stop <- w1636 stop-if-true
        # "25"
        n1270 = global write "Robot Global Data.vi" "in ctl num"(i16 0 ("retainer num")) -> ()
        n1271 = global write "Robot Global Data.vi" "Slew"(0.2 ("1-Y")) -> ()
        n1272 = global read "Robot Global Data.vi" "Yaw"() -> (w1638:dbl)
        n1273 = global write "Robot Global Data.vi" "retainer num"(i16 0 ("retainer num")) -> ()
        n1274 = global write "Robot Global Data.vi" "1-Trigger"(FALSE ("In pos")) -> ()
        n1275 = Greater?(x=w1638, y=15.0) -> (0:w1636:bool)
        n1276 = global write "Robot Global Data.vi" "1-Y"(0.0 ("1-Y")) -> ()
        n1277 = global write "Robot Global Data.vi" "1-X"(0.8 ("1-X")) -> ()
        n1278 = Wait (ms)(milliseconds to wait=u32 20) -> ()  [unwired: 1 out]
      }
      n1279 = while {
        tunnel: w1553 -> [w1628]
        tunnel: [w1628] -> w1552
        stop <- TRUE stop-if-true
        # "stop"
        n1280 = global write "Robot Global Data.vi" "1-X"(0.0 ("1-X")) -> ()
        n1281 = global write "Robot Global Data.vi" "1-Y"(0.0 ("1-X")) -> ()
        n1282 = Wait (ms)(milliseconds to wait=u32 700) -> ()  [unwired: 1 out]
      }
      n1283 = while {
        tunnel: w1552 -> [w1623]
        tunnel: [w1623] -> w1549
        stop <- TRUE stop-if-true
        # "stop"
        n1284 = global write "Robot Global Data.vi" "1-X"(0.0 ("1-X")) -> ()
        n1285 = global write "Robot Global Data.vi" "Slew"(0.2 ("1-Y")) -> ()
        n1286 = global write "Robot Global Data.vi" "1-Y"(0.0 ("1-X")) -> ()
        n1287 = Wait (ms)(milliseconds to wait=u32 20) -> ()  [unwired: 1 out]
      }
      n1288 = while {
        tunnel: [w1704] -> w1562
        tunnel: w1549 -> [w1704]
        stop <- w1706 stop-if-true
        n1289 = global write "Robot Global Data.vi" "Shot Selector"(FALSE ("In pos")) -> ()
        n1290 = global write "Robot Global Data.vi" "1-Button 8"(TRUE ("1-Button 8")) -> ()
        n1291 = global read "Robot Global Data.vi" "4?"() -> (w1706:bool)
        n1292 = Wait (ms)(milliseconds to wait=u32 20) -> ()  [unwired: 1 out]
      }
      n1293 = while {
        tunnel: w1562 -> [w1690]
        tunnel: [w1690] -> w1560
        stop <- TRUE stop-if-true
        n1294 = Wait (ms)(milliseconds to wait=u32 250) -> ()  [unwired: 1 out]
      }
      n1295 = while {
        tunnel: [w1701] -> w1561
        tunnel: w1560 -> [w1701]
        i -> [w1699]
        stop <- w1697 stop-if-true
        n1296 = global write "Robot Global Data.vi" "Shoot!"(TRUE ("1-Button 8")) -> ()
        n1297 = Greater?(x=w1699, y=5) -> (0:w1697:bool)
        n1298 = Wait (ms)(milliseconds to wait=u32 20) -> ()  [unwired: 1 out]
      }
      n1299 = while {
        tunnel: [w1695] -> w1559
        tunnel: w1561 -> [w1695]
        stop <- TRUE stop-if-true
        n1300 = global write "Robot Global Data.vi" "Shoot!"(FALSE ("1-Button 8")) -> ()
        n1301 = Wait (ms)(milliseconds to wait=u32 700) -> ()  [unwired: 1 out]
      }
      n1302 = while {
        tunnel: w1559 -> [w1797]
        tunnel: [w1797] -> w1570
        stop <- FALSE stop-if-true
        w1795 = 0.0 ("1-X")
        n1303 = global write "Robot Global Data.vi" "1-X"(w1795) -> ()
        n1304 = global write "Robot Global Data.vi" "1-Y"(w1795) -> ()
      }
    }
    frame 15 {
      # "OLD 2 BALL"
      # "LAST THING JACOB DID ON 4/20"
      # "APPRX GOAL"
      # "and STOP"
      # "DO IT AGAIN"
      # "PICK UP"
      # "COME BACK"
      # "TURN TO 0"
      # "FIRE"
      # "AIM"
      # "SICK DROPS"
      # "S CURVE"
      # "APPRX GOAL"
      # "DISRGARD ALL COMMENTS NOT IN CAPS"
      # "2 BALL?"
      n1305 = while {
        tunnel: w1848 -> [w2018]
        tunnel: [w2018] -> w1847
        i -> [w2011]
        stop <- w2015 stop-if-true
        # "stop"
        n1306 = global write "Robot Global Data.vi" "Arm Control"(-1.0 ("retainer num")) -> ()
        n1307 = global write "Robot Global Data.vi" "In pos"(TRUE ("In pos")) -> ()
        n1308 = global write "Robot Global Data.vi" "in ctl num"(i16 2 ("retainer num")) -> ()
        n1309 = global write "Robot Global Data.vi" "1-Trigger"(TRUE ("In pos")) -> ()
        n1310 = global write "Robot Global Data.vi" "retainer num"(i16 2 ("retainer num")) -> ()
        n1311 = global write "Robot Global Data.vi" "1-X"(0.0 ("1-X")) -> ()
        n1312 = Greater?(x=w2011, y=15) -> (0:w2015:bool)
        n1313 = global write "Robot Global Data.vi" "1-Y"(0.0 ("1-X")) -> ()
        n1314 = Wait (ms)(milliseconds to wait=u32 20) -> ()  [unwired: 1 out]
      }
      n1315 = while {
        tunnel: w1847 -> [w2006]
        tunnel: [w2006] -> w1846
        i -> [w1999]
        stop <- w2003 stop-if-true
        # "stop"
        n1316 = global write "Robot Global Data.vi" "In pos"(TRUE ("In pos")) -> ()
        n1317 = global write "Robot Global Data.vi" "in ctl num"(i16 2 ("retainer num")) -> ()
        n1318 = global write "Robot Global Data.vi" "retainer num"(i16 2 ("retainer num")) -> ()
        n1319 = global write "Robot Global Data.vi" "Arm Control"(1.0 ("retainer num")) -> ()
        n1320 = global write "Robot Global Data.vi" "1-X"(0.0 ("1-X")) -> ()
        n1321 = Greater?(x=w1999, y=17) -> (0:w2003:bool)
        n1322 = global write "Robot Global Data.vi" "1-Y"(0.0 ("1-X")) -> ()
        n1323 = Wait (ms)(milliseconds to wait=u32 20) -> ()  [unwired: 1 out]
      }
      n1324 = while {
        tunnel: w1846 -> [w2044]
        tunnel: [w2044] -> w1849
        stop <- w2040 stop-if-true
        # "-23"
        # "218"
        # "thru the low bar"
        n1325 = global read "Robot Global Data.vi" "Distance (enc.)"() -> (w2042:dbl)
        n1326 = global write "Robot Global Data.vi" "1-Y"(-0.8 ("1-X")) -> ()
        n1327 = global read "Robot Global Data.vi" "Yaw"() -> (w2035:dbl)
        n1328 = global write "Robot Global Data.vi" "Pins / Intake timing"(0.0 ("Pins / Intake timing")) -> ()
        n1329 = call-poly <vilib>:"PID.vi"("output range"=cluster{"output high":dbl, "output low":dbl} {"output high"=0.8, "output low"=-0.8} ("output range 2"), "PID gains"=T7 {"proportional gain (Kc)"=0.048, "integral time (Ti, min)"=0.015, "derivative time (Td, min)"=0.0} ("PID gains 2"), "process variable"=w2035, "setpoint"=-26.0) -> ("output"=w2037:dbl)  [unwired: 6 in, 1 out]
        n1330 = Greater?(x=w2042, y=16.0) -> (0:w2040:bool)
        n1331 = global write "Robot Global Data.vi" "1-X"(w2037) -> ()
        n1332 = Wait (ms)(milliseconds to wait=u32 20) -> ()  [unwired: 1 out]
      }
      n1333 = while {
        tunnel: w1849 -> [w2033]
        tunnel: [w2033] -> w1833
        stop <- w2029 stop-if-true
        # "125"
        # "thru the low bar"
        n1334 = global write "Robot Global Data.vi" "in ctl num"(i16 0 ("retainer num")) -> ()
        n1335 = global read "Robot Global Data.vi" "Distance (enc.)"() -> (w2031:dbl)
        n1336 = global write "Robot Global Data.vi" "1-Y"(-1.0 ("1-X")) -> ()
        n1337 = global read "Robot Global Data.vi" "Yaw"() -> (w2024:dbl)
        n1338 = call-poly <vilib>:"PID.vi"("output range"=cluster{"output high":dbl, "output low":dbl} {"output high"=0.8, "output low"=-0.8} ("output range 2"), "PID gains"=T7 {"proportional gain (Kc)"=0.048, "integral time (Ti, min)"=0.015, "derivative time (Td, min)"=0.0} ("PID gains 2"), "process variable"=w2024, "setpoint"=4.0) -> ("output"=w2026:dbl)  [unwired: 6 in, 1 out]
        n1339 = Greater?(x=w2031, y=100.0) -> (0:w2029:bool)
        n1340 = global write "Robot Global Data.vi" "1-X"(w2026) -> ()
        n1341 = global write "Robot Global Data.vi" "Slew"(0.2 ("1-Y")) -> ()
        n1342 = global write "Robot Global Data.vi" "In pos"(TRUE ("In pos")) -> ()
        n1343 = Wait (ms)(milliseconds to wait=u32 20) -> ()  [unwired: 1 out]
      }
      n1344 = while {
        tunnel: w1833 -> [w1904]
        tunnel: [w1904] -> w1832
        stop <- w1900 stop-if-true
        # "125"
        # "thru the low bar"
        n1345 = global write "Robot Global Data.vi" "in ctl num"(i16 0 ("retainer num")) -> ()
        n1346 = global read "Robot Global Data.vi" "Distance (enc.)"() -> (w1902:dbl)
        n1347 = global write "Robot Global Data.vi" "1-Y"(-1.0 ("1-X")) -> ()
        n1348 = global read "Robot Global Data.vi" "Yaw"() -> (w1895:dbl)
        n1349 = call-poly <vilib>:"PID.vi"("output range"=cluster{"output high":dbl, "output low":dbl} {"output high"=0.8, "output low"=-0.8} ("output range 2"), "PID gains"=T7 {"proportional gain (Kc)"=0.048, "integral time (Ti, min)"=0.015, "derivative time (Td, min)"=0.0} ("PID gains 2"), "process variable"=w1895, "setpoint"=4.0) -> ("output"=w1897:dbl)  [unwired: 6 in, 1 out]
        n1350 = Greater?(x=w1902, y=175.0) -> (0:w1900:bool)
        n1351 = global write "Robot Global Data.vi" "1-X"(w1897) -> ()
        n1352 = global write "Robot Global Data.vi" "Slew"(0.04 ("1-Y")) -> ()
        n1353 = global write "Robot Global Data.vi" "In pos"(TRUE ("In pos")) -> ()
        n1354 = Wait (ms)(milliseconds to wait=u32 20) -> ()  [unwired: 1 out]
      }
      n1355 = while {
        tunnel: w1832 -> [w1926]
        tunnel: [w1926] -> w1837
        stop <- w1922 stop-if-true
        # "35"
        n1356 = global write "Robot Global Data.vi" "in ctl num"(i16 0 ("retainer num")) -> ()
        n1357 = global write "Robot Global Data.vi" "Slew"(0.2 ("1-Y")) -> ()
        n1358 = global read "Robot Global Data.vi" "Yaw"() -> (w1924:dbl)
        n1359 = global write "Robot Global Data.vi" "retainer num"(i16 0 ("retainer num")) -> ()
        n1360 = global write "Robot Global Data.vi" "1-Trigger"(FALSE ("In pos")) -> ()
        n1361 = Greater?(x=w1924, y=15.0) -> (0:w1922:bool)
        n1362 = global write "Robot Global Data.vi" "1-Y"(0.0 ("1-Y")) -> ()
        n1363 = global write "Robot Global Data.vi" "1-X"(0.8 ("1-X")) -> ()
        n1364 = Wait (ms)(milliseconds to wait=u32 20) -> ()  [unwired: 1 out]
      }
      n1365 = while {
        tunnel: w1837 -> [w1914]
        tunnel: [w1914] -> w1835
        stop <- TRUE stop-if-true
        # "stop"
        n1366 = global write "Robot Global Data.vi" "1-X"(0.0 ("1-X")) -> ()
        n1367 = global write "Robot Global Data.vi" "1-Y"(0.0 ("1-X")) -> ()
        n1368 = Wait (ms)(milliseconds to wait=u32 600) -> ()  [unwired: 1 out]
      }
      n1369 = while {
        tunnel: w1835 -> [w1909]
        tunnel: [w1909] -> w1834
        stop <- TRUE stop-if-true
        # "stop"
        n1370 = global write "Robot Global Data.vi" "1-X"(0.0 ("1-X")) -> ()
        n1371 = global write "Robot Global Data.vi" "Slew"(0.2 ("1-Y")) -> ()
        n1372 = global write "Robot Global Data.vi" "1-Y"(0.0 ("1-X")) -> ()
        n1373 = Wait (ms)(milliseconds to wait=u32 20) -> ()  [unwired: 1 out]
      }
      n1374 = while {
        tunnel: [w2075] -> w1852
        tunnel: w1834 -> [w2075]
        stop <- w2077 stop-if-true
        n1375 = global write "Robot Global Data.vi" "Shot Selector"(FALSE ("In pos")) -> ()
        n1376 = global write "Robot Global Data.vi" "1-Button 8"(TRUE ("1-Button 8")) -> ()
        n1377 = global read "Robot Global Data.vi" "4?"() -> (w2077:bool)
        n1378 = Wait (ms)(milliseconds to wait=u32 20) -> ()  [unwired: 1 out]
      }
      n1379 = while {
        tunnel: w1852 -> [w2061]
        tunnel: [w2061] -> w1853
        stop <- TRUE stop-if-true
        n1380 = Wait (ms)(milliseconds to wait=u32 200) -> ()  [unwired: 1 out]
      }
      n1381 = while {
        tunnel: [w2072] -> w1854
        tunnel: w1853 -> [w2072]
        i -> [w2070]
        stop <- w2068 stop-if-true
        n1382 = global write "Robot Global Data.vi" "Shoot!"(TRUE ("1-Button 8")) -> ()
        n1383 = Greater?(x=w2070, y=5) -> (0:w2068:bool)
        n1384 = Wait (ms)(milliseconds to wait=u32 20) -> ()  [unwired: 1 out]
      }
      n1385 = while {
        tunnel: [w2066] -> w1851
        tunnel: w1854 -> [w2066]
        stop <- TRUE stop-if-true
        n1386 = global write "Robot Global Data.vi" "Shoot!"(FALSE ("1-Button 8")) -> ()
        n1387 = Wait (ms)(milliseconds to wait=u32 500) -> ()  [unwired: 1 out]
      }
      n1388 = while {
        tunnel: w1851 -> [w2058]
        tunnel: [w2058] -> w1844
        stop <- TRUE stop-if-true
        n1389 = global write "Robot Global Data.vi" "1-Button 8"(FALSE ("1-Button 8")) -> ()
        n1390 = Wait (ms)(milliseconds to wait=u32 20) -> ()  [unwired: 1 out]
      }
      n1391 = while {
        tunnel: w1844 -> [w1991]
        tunnel: [w1991] -> w1845
        stop <- w1993 stop-if-true
        # "13"
        n1392 = global read "Robot Global Data.vi" "Yaw"() -> (w1990:dbl)
        n1393 = global write "Robot Global Data.vi" "1-Button 8"(FALSE ("1-Button 8")) -> ()
        n1394 = Sign(1:w1990) -> (0:w1989:dbl)
        n1395 = global read "Robot Global Data.vi" "Yaw"() -> (w1996:dbl)
        n1396 = Multiply(x=-0.65, y=w1989) -> (x*y=w1987:dbl)
        n1397 = global write "Robot Global Data.vi" "retainer num"(i16 2 ("retainer num")) -> ()
        n1398 = Absolute Value(x=w1996) -> (abs(x)=w1995:dbl)
        n1399 = Less?(x=w1995, y=21.0) -> (x < y?=w1993:bool)
        n1400 = global write "Robot Global Data.vi" "1-X"(w1987) -> ()
        n1401 = Wait (ms)(milliseconds to wait=u32 20) -> ()  [unwired: 1 out]
      }
      n1402 = while {
        tunnel: w1845 -> [w1983]
        tunnel: [w1983] -> w1843
        stop <- w1979 stop-if-true
        # "218"
        # "thru the low bar"
        n1403 = global write "Robot Global Data.vi" "in ctl num"(i16 0 ("retainer num")) -> ()
        n1404 = global read "Robot Global Data.vi" "Distance (enc.)"() -> (w1981:dbl)
        n1405 = global write "Robot Global Data.vi" "1-Y"(1.0 ("1-X")) -> ()
        n1406 = global read "Robot Global Data.vi" "Yaw"() -> (w1974:dbl)
        n1407 = call-poly <vilib>:"PID.vi"("output range"=cluster{"output high":dbl, "output low":dbl} {"output high"=0.8, "output low"=-0.8} ("output range 2"), "PID gains"=T7 {"proportional gain (Kc)"=0.048, "integral time (Ti, min)"=0.015, "derivative time (Td, min)"=0.0} ("PID gains 2"), "process variable"=w1974, "setpoint"=1.0) -> ("output"=w1976:dbl)  [unwired: 6 in, 1 out]
        n1408 = Less?(x=w1981, y=90.0) -> (x < y?=w1979:bool)
        n1409 = global write "Robot Global Data.vi" "In pos"(TRUE ("In pos")) -> ()
        n1410 = global write "Robot Global Data.vi" "1-X"(w1976) -> ()
        n1411 = Wait (ms)(milliseconds to wait=u32 20) -> ()  [unwired: 1 out]
      }
      n1412 = while {
        tunnel: w1843 -> [w1970]
        tunnel: [w1970] -> w1836
        stop <- w1966 stop-if-true
        # "32"
        # "thru the low bar"
        n1413 = global write "Robot Global Data.vi" "in ctl num"(i16 2 ("retainer num")) -> ()
        n1414 = global read "Robot Global Data.vi" "Distance (enc.)"() -> (w1968:dbl)
        n1415 = global write "Robot Global Data.vi" "1-Y"(0.66 ("1-X")) -> ()
        n1416 = global read "Robot Global Data.vi" "Yaw"() -> (w1961:dbl)
        n1417 = call-poly <vilib>:"PID.vi"("output range"=cluster{"output high":dbl, "output low":dbl} {"output high"=0.8, "output low"=-0.8} ("output range 2"), "PID gains"=T7 {"proportional gain (Kc)"=0.048, "integral time (Ti, min)"=0.015, "derivative time (Td, min)"=0.0} ("PID gains 2"), "process variable"=w1961, "setpoint"=0.0) -> ("output"=w1963:dbl)  [unwired: 6 in, 1 out]
        n1418 = Less?(x=w1968, y=42.0) -> (x < y?=w1966:bool)
        n1419 = global write "Robot Global Data.vi" "1-Trigger"(TRUE ("In pos")) -> ()
        n1420 = global write "Robot Global Data.vi" "In pos"(TRUE ("In pos")) -> ()
        n1421 = global write "Robot Global Data.vi" "1-X"(w1963) -> ()
        n1422 = Wait (ms)(milliseconds to wait=u32 20) -> ()  [unwired: 1 out]
      }
      n1423 = while {
        tunnel: w1836 -> [w2053]
        tunnel: [w2052] -> w1842
        i -> [w2050]
        stop <- w2051 stop-if-true
        w2055 = 0.0 ("1-X")
        n1424 = call <vilib>:"WPI_EncoderReset.vi"("EncoderDevRef"=w2053) -> ("EncoderDevRef"=w2052:T3)  [unwired: 9 in, 1 out]
        n1425 = Wait (ms)(milliseconds to wait=u32 20) -> ()  [unwired: 1 out]
        n1426 = global write "Robot Global Data.vi" "1-X"(w2055) -> ()
        n1427 = Greater?(x=w2050, y=10) -> (0:w2051:bool)
        n1428 = global write "Robot Global Data.vi" "1-Y"(w2055) -> ()
      }
      n1429 = while {
        tunnel: w1842 -> [w1938]
        tunnel: [w1938] -> w1828
        stop <- w1934 stop-if-true
        # "115"
        # "218"
        # "thru the low bar"
        n1430 = global write "Robot Global Data.vi" "in ctl num"(i16 2 ("retainer num")) -> ()
        n1431 = global read "Robot Global Data.vi" "Distance (enc.)"() -> (w1936:dbl)
        n1432 = global write "Robot Global Data.vi" "1-Y"(-1.0 ("1-X")) -> ()
        n1433 = global read "Robot Global Data.vi" "Yaw"() -> (w1929:dbl)
        n1434 = call-poly <vilib>:"PID.vi"("output range"=cluster{"output high":dbl, "output low":dbl} {"output high"=0.8, "output low"=-0.8} ("output range 2"), "PID gains"=T7 {"proportional gain (Kc)"=0.048, "integral time (Ti, min)"=0.015, "derivative time (Td, min)"=0.0} ("PID gains 2"), "process variable"=w1929, "setpoint"=0.0) -> ("output"=w1931:dbl)  [unwired: 6 in, 1 out]
        n1435 = Greater?(x=w1936, y=100.0) -> (0:w1934:bool)
        n1436 = global write "Robot Global Data.vi" "In pos"(TRUE ("In pos")) -> ()
        n1437 = global write "Robot Global Data.vi" "1-X"(w1931) -> ()
        n1438 = Wait (ms)(milliseconds to wait=u32 20) -> ()  [unwired: 1 out]
      }
      n1439 = while {
        tunnel: w1828 -> [w1868]
        tunnel: [w1868] -> w1829
        stop <- w1864 stop-if-true
        # "125"
        # "thru the low bar"
        n1440 = global write "Robot Global Data.vi" "in ctl num"(i16 0 ("retainer num")) -> ()
        n1441 = global read "Robot Global Data.vi" "Distance (enc.)"() -> (w1866:dbl)
        n1442 = global write "Robot Global Data.vi" "1-Y"(-1.0 ("1-X")) -> ()
        n1443 = global read "Robot Global Data.vi" "Yaw"() -> (w1859:dbl)
        n1444 = call-poly <vilib>:"PID.vi"("output range"=cluster{"output high":dbl, "output low":dbl} {"output high"=0.8, "output low"=-0.8} ("output range 2"), "PID gains"=T7 {"proportional gain (Kc)"=0.048, "integral time (Ti, min)"=0.015, "derivative time (Td, min)"=0.0} ("PID gains 2"), "process variable"=w1859, "setpoint"=5.0) -> ("output"=w1861:dbl)  [unwired: 6 in, 1 out]
        n1445 = Greater?(x=w1866, y=175.0) -> (0:w1864:bool)
        n1446 = global write "Robot Global Data.vi" "1-X"(w1861) -> ()
        n1447 = global write "Robot Global Data.vi" "Slew"(0.04 ("1-Y")) -> ()
        n1448 = global write "Robot Global Data.vi" "In pos"(TRUE ("In pos")) -> ()
        n1449 = Wait (ms)(milliseconds to wait=u32 20) -> ()  [unwired: 1 out]
      }
      n1450 = while {
        tunnel: w1829 -> [w1890]
        tunnel: [w1890] -> w1831
        stop <- w1886 stop-if-true
        # "25"
        n1451 = global write "Robot Global Data.vi" "in ctl num"(i16 0 ("retainer num")) -> ()
        n1452 = global write "Robot Global Data.vi" "Slew"(0.2 ("1-Y")) -> ()
        n1453 = global read "Robot Global Data.vi" "Yaw"() -> (w1888:dbl)
        n1454 = global write "Robot Global Data.vi" "retainer num"(i16 0 ("retainer num")) -> ()
        n1455 = global write "Robot Global Data.vi" "1-Trigger"(FALSE ("In pos")) -> ()
        n1456 = Greater?(x=w1888, y=15.0) -> (0:w1886:bool)
        n1457 = global write "Robot Global Data.vi" "1-Y"(0.0 ("1-Y")) -> ()
        n1458 = global write "Robot Global Data.vi" "1-X"(0.75 ("1-X")) -> ()
        n1459 = Wait (ms)(milliseconds to wait=u32 20) -> ()  [unwired: 1 out]
      }
      n1460 = while {
        tunnel: w1831 -> [w1878]
        tunnel: [w1878] -> w1830
        stop <- TRUE stop-if-true
        # "stop"
        n1461 = global write "Robot Global Data.vi" "1-X"(0.0 ("1-X")) -> ()
        n1462 = global write "Robot Global Data.vi" "1-Y"(0.0 ("1-X")) -> ()
        n1463 = Wait (ms)(milliseconds to wait=u32 700) -> ()  [unwired: 1 out]
      }
      n1464 = while {
        tunnel: w1830 -> [w1873]
        tunnel: [w1873] -> w1827
        stop <- TRUE stop-if-true
        # "stop"
        n1465 = global write "Robot Global Data.vi" "1-X"(0.0 ("1-X")) -> ()
        n1466 = global write "Robot Global Data.vi" "Slew"(0.2 ("1-Y")) -> ()
        n1467 = global write "Robot Global Data.vi" "1-Y"(0.0 ("1-X")) -> ()
        n1468 = Wait (ms)(milliseconds to wait=u32 20) -> ()  [unwired: 1 out]
      }
      n1469 = while {
        tunnel: [w1955] -> w1841
        tunnel: w1827 -> [w1955]
        stop <- w1957 stop-if-true
        n1470 = global write "Robot Global Data.vi" "Shot Selector"(FALSE ("In pos")) -> ()
        n1471 = global write "Robot Global Data.vi" "1-Button 8"(TRUE ("1-Button 8")) -> ()
        n1472 = global read "Robot Global Data.vi" "4?"() -> (w1957:bool)
        n1473 = Wait (ms)(milliseconds to wait=u32 20) -> ()  [unwired: 1 out]
      }
      n1474 = while {
        tunnel: w1841 -> [w1941]
        tunnel: [w1941] -> w1839
        stop <- TRUE stop-if-true
        n1475 = Wait (ms)(milliseconds to wait=u32 250) -> ()  [unwired: 1 out]
      }
      n1476 = while {
        tunnel: [w1952] -> w1840
        tunnel: w1839 -> [w1952]
        i -> [w1950]
        stop <- w1948 stop-if-true
        n1477 = global write "Robot Global Data.vi" "Shoot!"(TRUE ("1-Button 8")) -> ()
        n1478 = Greater?(x=w1950, y=5) -> (0:w1948:bool)
        n1479 = Wait (ms)(milliseconds to wait=u32 20) -> ()  [unwired: 1 out]
      }
      n1480 = while {
        tunnel: [w1946] -> w1838
        tunnel: w1840 -> [w1946]
        stop <- TRUE stop-if-true
        n1481 = global write "Robot Global Data.vi" "Shoot!"(FALSE ("1-Button 8")) -> ()
        n1482 = Wait (ms)(milliseconds to wait=u32 700) -> ()  [unwired: 1 out]
      }
      n1483 = while {
        tunnel: w1838 -> [w2048]
        tunnel: [w2048] -> w1850
        stop <- FALSE stop-if-true
        w2046 = 0.0 ("1-X")
        n1484 = global write "Robot Global Data.vi" "1-X"(w2046) -> ()
        n1485 = global write "Robot Global Data.vi" "1-Y"(w2046) -> ()
      }
    }
  }
  n1486 = global read "Robot Global Data.vi" "Starting Position"() -> (w6:i32)
  n1487 = global read "Robot Global Data.vi" "Defense to Cross"() -> (w11:i32)
  n1488 = Equal?(x=w11, y=2) -> (x = y?=w9:bool)
  n1489 = Select(t=1, s=w9, f=w6) -> (s? t:f=w7:i32)
  n1490 = case shown="6, Default" w7 {
    tunnel: w3 -> [w2085 w2125 w2262 w2312 w2366 w2406]
    tunnel: [w2078 w2124 w2258 w2308 w2359 w2406] -> w4
    frame 1 {
      # "Stay here"
      # "Release shoot button"
      # "Shoot"
      # "Stop"
      # "Drive to Batter"
      # "Stop turn and reset encoder"
      # "Turn to angle"
      # "Low bar position"
      n1491 = while {
        tunnel: [w2114] -> w2084
        tunnel: w2085 -> [w2114]
        stop <- w2113 stop-if-true
        n1492 = global read "Robot Global Data.vi" "Yaw"() -> (w2119:dbl)
        n1493 = global read "Robot Global Data.vi" "Yaw"() -> (w2116:dbl)
        n1494 = call-poly <vilib>:"PID.vi"("output range"=cluster{"output high":dbl, "output low":dbl} {"output high"=0.8, "output low"=-0.8}, "PID gains"=T7 {"proportional gain (Kc)"=0.048, "integral time (Ti, min)"=0.015, "derivative time (Td, min)"=0.0}, "process variable"=w2119, "setpoint"=57.5) -> ("output"=w2118:dbl)  [unwired: 6 in, 1 out]
        n1495 = global write "Robot Global Data.vi" "1-X"(w2118) -> ()
        n1496 = Greater?(x=w2116, y=55.5) -> (0:w2113:bool)
        n1497 = Wait (ms)(milliseconds to wait=u32 20) -> ()  [unwired: 1 out]
      }
      n1498 = while {
        tunnel: [w2100] -> w2083
        tunnel: w2084 -> [w2101]
        stop <- TRUE stop-if-true
        # "stop"
        n1499 = call <vilib>:"WPI_EncoderReset.vi"("EncoderDevRef"=w2101) -> ("EncoderDevRef"=w2100:T3)  [unwired: 9 in, 1 out]
        n1500 = global write "Robot Global Data.vi" "1-X"(0.0 ("1-X")) -> ()
        n1501 = Wait (ms)(milliseconds to wait=u32 100) -> ()  [unwired: 1 out]
      }
      n1502 = while {
        tunnel: w2083 -> [w2098]
        tunnel: [w2098] -> w2082
        stop <- w2094 stop-if-true
        # "100"
        n1503 = global read "Robot Global Data.vi" "Distance (enc.)"() -> (w2096:dbl)
        n1504 = global write "Robot Global Data.vi" "1-Y"(-1.0 ("1-X")) -> ()
        n1505 = Greater?(x=w2096, y=100.0) -> (0:w2094:bool)
        n1506 = Wait (ms)(milliseconds to wait=u32 20) -> ()  [unwired: 1 out]
      }
      n1507 = while {
        tunnel: w2082 -> [w2091]
        tunnel: [w2091] -> w2081
        stop <- TRUE stop-if-true
        n1508 = global write "Robot Global Data.vi" "1-Y"(0.0 ("1-X")) -> ()
        n1509 = Wait (ms)(milliseconds to wait=u32 100) -> ()  [unwired: 1 out]
      }
      n1510 = while {
        tunnel: w2081 -> [w2109]
        tunnel: [w2109] -> w2080
        stop <- TRUE stop-if-true
        n1511 = global write "Robot Global Data.vi" "Shoot!"(TRUE ("Shoot!")) -> ()
        n1512 = Wait (ms)(milliseconds to wait=u32 50) -> ()  [unwired: 1 out]
      }
      n1513 = while {
        tunnel: w2080 -> [w2105]
        tunnel: [w2105] -> w2079
        stop <- TRUE stop-if-true
        n1514 = global write "Robot Global Data.vi" "Shoot!"(FALSE ("Shoot!")) -> ()
        n1515 = Wait (ms)(milliseconds to wait=u32 1500) -> ()  [unwired: 1 out]
      }
      n1516 = while {
        tunnel: [w2089] -> w2078
        tunnel: w2079 -> [w2089]
        stop <- FALSE stop-if-true
        n1517 = global write "Robot Global Data.vi" "1-Button 8"(FALSE ("1-Button 8")) -> ()
        n1518 = Wait (ms)(milliseconds to wait=u32 400) -> ()  [unwired: 1 out]
      }
    }
    frame 2 {
      # "Position two has an option to fade left or right into position 1 or 3, to better fit our partners auto mode."
      n1519 = global read "Robot Global Data.vi" "LR"() -> (w2123:bool)
      n1520 = case shown="True" w2123 {
        tunnel: w2125 -> [w2127 w2188]
        tunnel: [w2126 w2187] -> w2124
        frame False {
          # "Left"
          n1521 = while {
            tunnel: [w2160] -> w2133
            tunnel: w2127 -> [w2158]
            stop <- TRUE stop-if-true
            n1522 = call <vilib>:"WPI_EncoderReset.vi"("EncoderDevRef"=w2158) -> ("EncoderDevRef"=w2160:T3)  [unwired: 9 in, 1 out]
            n1523 = Wait (ms)(milliseconds to wait=u32 50) -> ()  [unwired: 1 out]
          }
          n1524 = while {
            tunnel: w2133 -> [w2176]
            tunnel: [w2176] -> w2135
            stop <- w2173 stop-if-true
            n1525 = global read "Robot Global Data.vi" "Distance (enc.)"() -> (w2175:dbl)
            n1526 = global read "Robot Global Data.vi" "Yaw"() -> (w2168:dbl)
            n1527 = call-poly <vilib>:"PID.vi"("output range"=cluster{"output high":dbl, "output low":dbl} {"output high"=0.8, "output low"=-0.8} ("output range 2"), "PID gains"=T7 {"proportional gain (Kc)"=0.048, "integral time (Ti, min)"=0.01, "derivative time (Td, min)"=0.0} ("PID gains 2"), "process variable"=w2168, "setpoint"=-20.0) -> ("output"=w2170:dbl)  [unwired: 6 in, 1 out]
            n1528 = global write "Robot Global Data.vi" "1-Y"(-1.0 ("1-X")) -> ()
            n1529 = Greater?(x=w2175, y=80.0) -> (0:w2173:bool)
            n1530 = global write "Robot Global Data.vi" "1-X"(w2170) -> ()
            n1531 = Wait (ms)(milliseconds to wait=u32 20) -> ()  [unwired: 1 out]
          }
          n1532 = while {
            tunnel: w2135 -> [w2165]
            tunnel: [w2165] -> w2134
            stop <- TRUE stop-if-true
            # "stop"
            n1533 = global write "Robot Global Data.vi" "1-X"(0.0 ("1-X")) -> ()
            n1534 = global write "Robot Global Data.vi" "1-Y"(0.0 ("1-X")) -> ()
            n1535 = Wait (ms)(milliseconds to wait=u32 50) -> ()  [unwired: 1 out]
          }
          n1536 = while {
            tunnel: [w2180] -> w2129
            tunnel: w2134 -> [w2180]
            stop <- w2183 stop-if-true
            # "Turn to angle"
            n1537 = global read "Robot Global Data.vi" "Yaw"() -> (w2181:dbl)
            n1538 = Greater?(x=w2181, y=20.0) -> (0:w2183:bool)
            n1539 = global write "Robot Global Data.vi" "1-X"(1.0 ("1-X")) -> ()
            n1540 = Wait (ms)(milliseconds to wait=u32 20) -> ()  [unwired: 1 out]
          }
          n1541 = while {
            tunnel: w2129 -> [w2142]
            tunnel: [w2142] -> w2130
            stop <- TRUE stop-if-true
            n1542 = global write "Robot Global Data.vi" "1-X"(0.0 ("1-X")) -> ()
            n1543 = Wait (ms)(milliseconds to wait=u32 500) -> ()  [unwired: 1 out]
          }
          n1544 = while {
            tunnel: [w2155] -> w2128
            tunnel: w2130 -> [w2155]
            stop <- w2157 stop-if-true
            n1545 = global write "Robot Global Data.vi" "Shot Selector"(FALSE ("In pos")) -> ()
            n1546 = global write "Robot Global Data.vi" "1-Button 8"(TRUE ("1-Button 8")) -> ()
            n1547 = global read "Robot Global Data.vi" "4?"() -> (w2157:bool)
            n1548 = Wait (ms)(milliseconds to wait=u32 20) -> ()  [unwired: 1 out]
          }
          n1549 = while {
            tunnel: w2128 -> [w2137]
            tunnel: [w2137] -> w2131
            stop <- TRUE stop-if-true
            n1550 = Wait (ms)(milliseconds to wait=u32 20) -> ()  [unwired: 1 out]
          }
          n1551 = while {
            tunnel: [w2152] -> w2132
            tunnel: w2131 -> [w2152]
            i -> [w2150]
            stop <- w2148 stop-if-true
            n1552 = global write "Robot Global Data.vi" "Shoot!"(TRUE ("1-Button 8")) -> ()
            n1553 = Greater?(x=w2150, y=5) -> (0:w2148:bool)
            n1554 = Wait (ms)(milliseconds to wait=u32 20) -> ()  [unwired: 1 out]
          }
          n1555 = while {
            tunnel: [w2146] -> w2126
            tunnel: w2132 -> [w2146]
            stop <- FALSE stop-if-true
            n1556 = global write "Robot Global Data.vi" "Shoot!"(FALSE ("1-Button 8")) -> ()
            n1557 = Wait (ms)(milliseconds to wait=u32 1500) -> ()  [unwired: 1 out]
          }
        }
        frame True {
          # "Left"
          n1558 = while {
            tunnel: [w2233] -> w2193
            tunnel: w2188 -> [w2231]
            stop <- TRUE stop-if-true
            n1559 = call <vilib>:"WPI_EncoderReset.vi"("EncoderDevRef"=w2231) -> ("EncoderDevRef"=w2233:T3)  [unwired: 9 in, 1 out]
            n1560 = Wait (ms)(milliseconds to wait=u32 50) -> ()  [unwired: 1 out]
          }
          n1561 = while {
            tunnel: w2193 -> [w2245]
            tunnel: [w2245] -> w2195
            stop <- w2242 stop-if-true
            n1562 = global read "Robot Global Data.vi" "Yaw"() -> (w2244:dbl)
            n1563 = global write "Robot Global Data.vi" "1-Y"(0.0 ("1-X")) -> ()
            n1564 = Greater?(x=w2244, y=40.0) -> (0:w2242:bool)
            n1565 = global write "Robot Global Data.vi" "1-X"(0.9 ("1-X")) -> ()
            n1566 = Wait (ms)(milliseconds to wait=u32 20) -> ()  [unwired: 1 out]
          }
          n1567 = while {
            tunnel: w2195 -> [w2238]
            tunnel: [w2238] -> w2194
            stop <- TRUE stop-if-true
            # "stop"
            n1568 = global write "Robot Global Data.vi" "1-X"(0.0 ("1-X")) -> ()
            n1569 = global write "Robot Global Data.vi" "1-Y"(0.0 ("1-X")) -> ()
            n1570 = Wait (ms)(milliseconds to wait=u32 50) -> ()  [unwired: 1 out]
          }
          n1571 = while {
            tunnel: [w2254] -> w2190
            tunnel: w2194 -> [w2254]
            stop <- w2257 stop-if-true
            # "Turn to angle"
            n1572 = global read "Robot Global Data.vi" "Distance (enc.)"() -> (w2255:dbl)
            n1573 = global read "Robot Global Data.vi" "Yaw"() -> (w2247:dbl)
            n1574 = Greater?(x=w2255, y=80.0) -> (0:w2257:bool)
            n1575 = call-poly <vilib>:"PID.vi"("output range"=cluster{"output high":dbl, "output low":dbl} {"output high"=0.8, "output low"=-0.8} ("output range 2"), "PID gains"=T7 {"proportional gain (Kc)"=0.048, "integral time (Ti, min)"=0.015, "derivative time (Td, min)"=0.0} ("PID gains 2"), "process variable"=w2247, "setpoint"=80.0) -> ("output"=w2249:dbl)  [unwired: 6 in, 1 out]
            n1576 = global write "Robot Global Data.vi" "1-Y"(-0.9 ("1-X")) -> ()
            n1577 = global write "Robot Global Data.vi" "1-X"(w2249) -> ()
            n1578 = Wait (ms)(milliseconds to wait=u32 20) -> ()  [unwired: 1 out]
          }
          n1579 = while {
            tunnel: w2190 -> [w2215]
            tunnel: [w2215] -> w2186
            stop <- TRUE stop-if-true
            n1580 = global write "Robot Global Data.vi" "1-Y"(0.0 ("1-X")) -> ()
            n1581 = global write "Robot Global Data.vi" "1-X"(0.0 ("1-X")) -> ()
            n1582 = Wait (ms)(milliseconds to wait=u32 500) -> ()  [unwired: 1 out]
          }
          n1583 = while {
            tunnel: w2186 -> [w2206]
            tunnel: [w2206] -> w2185
            stop <- w2203 stop-if-true
            n1584 = global read "Robot Global Data.vi" "Yaw"() -> (w2205:dbl)
            n1585 = global write "Robot Global Data.vi" "1-Y"(0.0 ("1-X")) -> ()
            n1586 = Less?(x=w2205, y=60.0) -> (x < y?=w2203:bool)
            n1587 = global write "Robot Global Data.vi" "1-X"(-0.9 ("1-X")) -> ()
            n1588 = Wait (ms)(milliseconds to wait=u32 20) -> ()  [unwired: 1 out]
          }
          n1589 = while {
            tunnel: w2185 -> [w2200]
            tunnel: [w2200] -> w2184
            stop <- TRUE stop-if-true
            n1590 = global write "Robot Global Data.vi" "1-Y"(0.0 ("1-X")) -> ()
            n1591 = global write "Robot Global Data.vi" "1-X"(0.0 ("1-X")) -> ()
            n1592 = Wait (ms)(milliseconds to wait=u32 1000) -> ()  [unwired: 1 out]
          }
          n1593 = while {
            tunnel: [w2228] -> w2189
            tunnel: w2184 -> [w2228]
            stop <- w2230 stop-if-true
            n1594 = global write "Robot Global Data.vi" "Shot Selector"(FALSE ("In pos")) -> ()
            n1595 = global write "Robot Global Data.vi" "1-Button 8"(TRUE ("1-Button 8")) -> ()
            n1596 = global read "Robot Global Data.vi" "4?"() -> (w2230:bool)
            n1597 = Wait (ms)(milliseconds to wait=u32 20) -> ()  [unwired: 1 out]
          }
          n1598 = while {
            tunnel: w2189 -> [w2209]
            tunnel: [w2209] -> w2191
            stop <- TRUE stop-if-true
            n1599 = Wait (ms)(milliseconds to wait=u32 20) -> ()  [unwired: 1 out]
          }
          n1600 = while {
            tunnel: [w2225] -> w2192
            tunnel: w2191 -> [w2225]
            i -> [w2223]
            stop <- w2221 stop-if-true
            n1601 = global write "Robot Global Data.vi" "Shoot!"(TRUE ("1-Button 8")) -> ()
            n1602 = Greater?(x=w2223, y=5) -> (0:w2221:bool)
            n1603 = Wait (ms)(milliseconds to wait=u32 20) -> ()  [unwired: 1 out]
          }
          n1604 = while {
            tunnel: [w2219] -> w2187
            tunnel: w2192 -> [w2219]
            stop <- FALSE stop-if-true
            n1605 = global write "Robot Global Data.vi" "Shoot!"(FALSE ("1-Button 8")) -> ()
            n1606 = Wait (ms)(milliseconds to wait=u32 1500) -> ()  [unwired: 1 out]
          }
        }
      }
    }
    frame 3 {
      # "Release the shoot button."
      # "Fire the catapult."
      # "Brief pause before shooting while holding aim."
      # "Select a \"far\" shot and start aiming sequence."
      # "Stop and let the robot\ncome to rest before\naiming."
      # "Drive deeper (straight) into the goal to avoid\nthe apex of our shot arch.  Notice that Y is still\nthe speed from the defense crossing."
      # "Reset encoder to prepare to\ndrive deeper."
      # "Position 3 (Just left of center goall.)"
      n1607 = while {
        tunnel: w2262 -> [w2276]
        tunnel: [w2274] -> w2261
        stop <- TRUE stop-if-true
        n1608 = call <vilib>:"WPI_EncoderReset.vi"("EncoderDevRef"=w2276) -> ("EncoderDevRef"=w2274:T3)  [unwired: 9 in, 1 out]
        n1609 = Wait (ms)(milliseconds to wait=u32 20) -> ()  [unwired: 1 out]
      }
      n1610 = while {
        tunnel: w2261 -> [w2287]
        tunnel: [w2287] -> w2263
        stop <- w2283 stop-if-true
        # "30"
        n1611 = global read "Robot Global Data.vi" "Distance (enc.)"() -> (w2285:dbl)
        n1612 = global read "Robot Global Data.vi" "Yaw"() -> (w2278:dbl)
        n1613 = call-poly <vilib>:"PID.vi"("output range"=cluster{"output high":dbl, "output low":dbl} {"output high"=0.8, "output low"=-0.8} ("output range 2"), "PID gains"=T7 {"proportional gain (Kc)"=0.048, "integral time (Ti, min)"=0.015, "derivative time (Td, min)"=0.0} ("PID gains 2"), "process variable"=w2278, "setpoint"=0.0) -> ("output"=w2280:dbl)  [unwired: 6 in, 1 out]
        n1614 = Greater?(x=w2285, y=10.0) -> (0:w2283:bool)
        n1615 = global write "Robot Global Data.vi" "1-X"(w2280) -> ()
        n1616 = Wait (ms)(milliseconds to wait=u32 20) -> ()  [unwired: 1 out]
      }
      n1617 = while {
        tunnel: w2263 -> [w2292]
        tunnel: [w2292] -> w2264
        stop <- TRUE stop-if-true
        # "800"
        n1618 = global write "Robot Global Data.vi" "1-X"(0.0 ("1-X")) -> ()
        n1619 = global write "Robot Global Data.vi" "1-Y"(0.0 ("1-Y")) -> ()
        n1620 = Wait (ms)(milliseconds to wait=u32 500) -> ()  [unwired: 1 out]
      }
      n1621 = while {
        tunnel: [w2305] -> w2260
        tunnel: w2264 -> [w2305]
        stop <- w2307 stop-if-true
        n1622 = global write "Robot Global Data.vi" "Shot Selector"(FALSE ("In pos")) -> ()
        n1623 = global write "Robot Global Data.vi" "1-Button 8"(TRUE ("1-Button 8")) -> ()
        n1624 = global read "Robot Global Data.vi" "4?"() -> (w2307:bool)
        n1625 = Wait (ms)(milliseconds to wait=u32 20) -> ()  [unwired: 1 out]
      }
      n1626 = while {
        tunnel: [w2271] -> w2265
        tunnel: w2260 -> [w2271]
        stop <- TRUE stop-if-true
        # "500"
        n1627 = Wait (ms)(milliseconds to wait=u32 300) -> ()  [unwired: 1 out]
      }
      n1628 = while {
        tunnel: [w2302] -> w2266
        tunnel: w2265 -> [w2302]
        i -> [w2300]
        stop <- w2298 stop-if-true
        n1629 = global write "Robot Global Data.vi" "Shoot!"(TRUE ("1-Button 8")) -> ()
        n1630 = Greater?(x=w2300, y=5) -> (0:w2298:bool)
        n1631 = Wait (ms)(milliseconds to wait=u32 20) -> ()  [unwired: 1 out]
      }
      n1632 = while {
        tunnel: [w2296] -> w2259
        tunnel: w2266 -> [w2296]
        stop <- TRUE stop-if-true
        n1633 = global write "Robot Global Data.vi" "Shoot!"(FALSE ("1-Button 8")) -> ()
        n1634 = Wait (ms)(milliseconds to wait=u32 1200) -> ()  [unwired: 1 out]
      }
      n1635 = while {
        tunnel: [w2270] -> w2258
        tunnel: w2259 -> [w2270]
        stop <- TRUE stop-if-true
        n1636 = global write "Robot Global Data.vi" "1-Button 8"(FALSE ("1-Button 8")) -> ()
        n1637 = Wait (ms)(milliseconds to wait=u32 400) -> ()  [unwired: 1 out]
      }
    }
    frame 4 {
      # "Release the shoot button."
      # "Fire the catapult."
      # "Let robot come to rest before shooting."
      # "Select a \"far\" shot and start aiming sequence."
      # "Stop and let the robot\ncome to rest before\naiming."
      # "Drive deeper (straight) into the goal to avoid\nthe apex of our shot arch.  Notice that Y is still\nthe speed from the defense crossing."
      # "Reset encoder to prepare to\ndrive deeper."
      # "Position 4 (Most centered on goal.)"
      n1638 = while {
        tunnel: w2312 -> [w2327]
        tunnel: [w2325] -> w2311
        stop <- TRUE stop-if-true
        n1639 = call <vilib>:"WPI_EncoderReset.vi"("EncoderDevRef"=w2327) -> ("EncoderDevRef"=w2325:T3)  [unwired: 9 in, 1 out]
        n1640 = Wait (ms)(milliseconds to wait=u32 20) -> ()  [unwired: 1 out]
      }
      n1641 = while {
        tunnel: w2311 -> [w2338]
        tunnel: [w2338] -> w2313
        stop <- w2334 stop-if-true
        # "20"
        n1642 = global read "Robot Global Data.vi" "Distance (enc.)"() -> (w2336:dbl)
        n1643 = global read "Robot Global Data.vi" "Yaw"() -> (w2329:dbl)
        n1644 = call-poly <vilib>:"PID.vi"("output range"=cluster{"output high":dbl, "output low":dbl} {"output high"=0.8, "output low"=-0.8} ("output range 2"), "PID gains"=T7 {"proportional gain (Kc)"=0.048, "integral time (Ti, min)"=0.015, "derivative time (Td, min)"=0.0} ("PID gains 2"), "process variable"=w2329, "setpoint"=0.0) -> ("output"=w2331:dbl)  [unwired: 6 in, 1 out]
        n1645 = Greater?(x=w2336, y=15.0) -> (0:w2334:bool)
        n1646 = global write "Robot Global Data.vi" "1-X"(w2331) -> ()
        n1647 = Wait (ms)(milliseconds to wait=u32 20) -> ()  [unwired: 1 out]
      }
      n1648 = while {
        tunnel: w2313 -> [w2343]
        tunnel: [w2343] -> w2314
        stop <- TRUE stop-if-true
        n1649 = global write "Robot Global Data.vi" "1-X"(0.0 ("1-X")) -> ()
        n1650 = global write "Robot Global Data.vi" "1-Y"(0.0 ("1-Y")) -> ()
        n1651 = Wait (ms)(milliseconds to wait=u32 500) -> ()  [unwired: 1 out]
      }
      n1652 = while {
        tunnel: [w2356] -> w2310
        tunnel: w2314 -> [w2356]
        stop <- w2358 stop-if-true
        n1653 = global write "Robot Global Data.vi" "Shot Selector"(FALSE ("In pos")) -> ()
        n1654 = global write "Robot Global Data.vi" "1-Button 8"(TRUE ("1-Button 8")) -> ()
        n1655 = global read "Robot Global Data.vi" "4?"() -> (w2358:bool)
        n1656 = Wait (ms)(milliseconds to wait=u32 20) -> ()  [unwired: 1 out]
      }
      n1657 = while {
        tunnel: w2310 -> [w2323]
        tunnel: [w2323] -> w2315
        stop <- TRUE stop-if-true
        n1658 = global write "Robot Global Data.vi" "1-X"(0.0 ("1-X")) -> ()
        n1659 = Wait (ms)(milliseconds to wait=u32 20) -> ()  [unwired: 1 out]
      }
      n1660 = while {
        tunnel: [w2353] -> w2316
        tunnel: w2315 -> [w2353]
        i -> [w2351]
        stop <- w2349 stop-if-true
        n1661 = global write "Robot Global Data.vi" "Shoot!"(TRUE ("1-Button 8")) -> ()
        n1662 = Greater?(x=w2351, y=5) -> (0:w2349:bool)
        n1663 = Wait (ms)(milliseconds to wait=u32 20) -> ()  [unwired: 1 out]
      }
      n1664 = while {
        tunnel: [w2347] -> w2309
        tunnel: w2316 -> [w2347]
        stop <- TRUE stop-if-true
        n1665 = global write "Robot Global Data.vi" "Shoot!"(FALSE ("1-Button 8")) -> ()
        n1666 = Wait (ms)(milliseconds to wait=u32 1200) -> ()  [unwired: 1 out]
      }
      n1667 = while {
        tunnel: [w2320] -> w2308
        tunnel: w2309 -> [w2320]
        stop <- TRUE stop-if-true
        n1668 = global write "Robot Global Data.vi" "1-Button 8"(FALSE ("1-Button 8")) -> ()
        n1669 = Wait (ms)(milliseconds to wait=u32 400) -> ()  [unwired: 1 out]
      }
    }
    frame 5 {
      # "Fire the catapult."
      # "Brief pause before shooting."
      # "Select a \"far\" shot and start aiming sequence."
      # "Stop and let the robot\ncome to rest before\naiming."
      # "Turn left to angle (facing goal.)"
      # "Reset encoder to prepare to\ndrive deeper.  Stop all drive."
      # "Position 5 (Right of center goall.)"
      n1670 = while {
        tunnel: w2366 -> [w2390]
        tunnel: [w2388] -> w2365
        stop <- TRUE stop-if-true
        n1671 = call <vilib>:"WPI_EncoderReset.vi"("EncoderDevRef"=w2390) -> ("EncoderDevRef"=w2388:T3)  [unwired: 9 in, 1 out]
        n1672 = global write "Robot Global Data.vi" "1-Y"(0.0 ("1-Y")) -> ()
        n1673 = global write "Robot Global Data.vi" "1-X"(0.0 ("1-X")) -> ()
        n1674 = Wait (ms)(milliseconds to wait=u32 200) -> ()  [unwired: 1 out]
      }
      n1675 = while {
        tunnel: w2365 -> [w2385]
        tunnel: [w2385] -> w2364
        stop <- w2380 stop-if-true
        n1676 = global read "Robot Global Data.vi" "Yaw"() -> (w2383:dbl)
        n1677 = Less?(x=w2383, y=-10.0) -> (x < y?=w2380:bool)
        n1678 = global write "Robot Global Data.vi" "1-X"(-0.8 ("1-X")) -> ()
        n1679 = Wait (ms)(milliseconds to wait=u32 20) -> ()  [unwired: 1 out]
      }
      n1680 = while {
        tunnel: w2364 -> [w2395]
        tunnel: [w2395] -> w2362
        stop <- TRUE stop-if-true
        n1681 = global write "Robot Global Data.vi" "1-X"(0.0 ("1-X")) -> ()
        n1682 = Wait (ms)(milliseconds to wait=u32 500) -> ()  [unwired: 1 out]
      }
      n1683 = while {
        tunnel: [w2377] -> w2363
        tunnel: w2362 -> [w2377]
        stop <- w2379 stop-if-true
        n1684 = global write "Robot Global Data.vi" "Shot Selector"(FALSE ("In pos")) -> ()
        n1685 = global write "Robot Global Data.vi" "1-Button 8"(TRUE ("1-Button 8")) -> ()
        n1686 = global read "Robot Global Data.vi" "4?"() -> (w2379:bool)
        n1687 = Wait (ms)(milliseconds to wait=u32 20) -> ()  [unwired: 1 out]
      }
      n1688 = while {
        tunnel: w2363 -> [w2373]
        tunnel: [w2373] -> w2361
        stop <- TRUE stop-if-true
        n1689 = Wait (ms)(milliseconds to wait=u32 20) -> ()  [unwired: 1 out]
      }
      n1690 = while {
        tunnel: [w2405] -> w2367
        tunnel: w2361 -> [w2405]
        i -> [w2403]
        stop <- w2401 stop-if-true
        n1691 = global write "Robot Global Data.vi" "Shoot!"(TRUE ("1-Button 8")) -> ()
        n1692 = Greater?(x=w2403, y=5) -> (0:w2401:bool)
        n1693 = Wait (ms)(milliseconds to wait=u32 20) -> ()  [unwired: 1 out]
      }
      n1694 = while {
        tunnel: [w2399] -> w2360
        tunnel: w2367 -> [w2399]
        stop <- TRUE stop-if-true
        n1695 = global write "Robot Global Data.vi" "Shoot!"(FALSE ("1-Button 8")) -> ()
        n1696 = Wait (ms)(milliseconds to wait=u32 1500) -> ()  [unwired: 1 out]
      }
      n1697 = while {
        tunnel: [w2371] -> w2359
        tunnel: w2360 -> [w2371]
        stop <- TRUE stop-if-true
        n1698 = global write "Robot Global Data.vi" "1-Button 8"(FALSE ("1-Button 8")) -> ()
        n1699 = Wait (ms)(milliseconds to wait=u32 400) -> ()  [unwired: 1 out]
      }
    }
    frame 6, Default {
    }
  }
  n1700 = global read "Robot Global Data.vi" "Defense to Cross"() -> (w5:i32)
  n1701 = case shown="0" w5 {
    tunnel: w4 -> [w2408 w2463 w2466 w2503 w2540 w2577]
    frame 0 {
      # "To return on the port, spin around, come thru, spin again and put up the arms"
      # "Port"
      n1702 = global read "Robot Global Data.vi" "Starting Position"() -> (w2409:i32)
      n1703 = Not Equal?(x=w2409, y=2) -> (x != y?=w2407:bool)
      n1704 = case shown="True" w2407 {
        tunnel: w2408 -> [w2412 w2422]
        tunnel: [w2411 w2417] -> _
        frame False {
          n1705 = while {
            tunnel: w2412 -> [w2413]
            tunnel: [w2413] -> w2411
            stop <- FALSE stop-if-true
            n1706 = Wait (ms)(milliseconds to wait=u32 200) -> ()  [unwired: 1 out]
          }
        }
        frame True {
          n1707 = while {
            tunnel: [w2456] -> w2419
            tunnel: w2422 -> [w2456]
            stop <- w2458 stop-if-true
            # "Seriously though, my gyro rolls over at 180. It counts\n 179, 180, -180, -179..."
            # "Future me or anyone reading this:\nif it works, it works. Don't even ask"
            n1708 = global read "Robot Global Data.vi" "Yaw"() -> (w2461:dbl)
            n1709 = Absolute Value(x=w2461) -> (abs(x)=w2460:dbl)
            n1710 = Wait (ms)(milliseconds to wait=u32 20) -> ()  [unwired: 1 out]
            n1711 = Greater?(x=w2460, y=135.0) -> (0:w2458:bool)
            n1712 = global write "Robot Global Data.vi" "1-X"(-0.85 ("1-X")) -> ()
          }
          n1713 = while {
            tunnel: w2419 -> [w2433]
            tunnel: [w2433] -> w2418
            stop <- w2427 stop-if-true
            n1714 = global read "Robot Global Data.vi" "Yaw"() -> (w2430:dbl)
            n1715 = Absolute Value(x=w2430) -> (abs(x)=w2429:dbl)
            n1716 = Wait (ms)(milliseconds to wait=u32 30) -> ()  [unwired: 1 out]
            n1717 = global write "Robot Global Data.vi" "1-X"(-0.5 ("1-X")) -> ()
            n1718 = Greater?(x=w2429, y=175.0) -> (0:w2427:bool)
          }
          n1719 = while {
            tunnel: w2418 -> [w2450]
            tunnel: [w2449] -> w2420
            i -> [w2452]
            stop <- w2453 stop-if-true
            w2454 = 0.0 ("1-Y")
            n1720 = call <vilib>:"WPI_EncoderReset.vi"("EncoderDevRef"=w2450) -> ("EncoderDevRef"=w2449:T3)  [unwired: 9 in, 1 out]
            n1721 = global write "Robot Global Data.vi" "1-X"(w2454) -> ()
            n1722 = global write "Robot Global Data.vi" "1-Y"(w2454) -> ()
            n1723 = Greater?(x=w2452, y=5) -> (0:w2453:bool)
            n1724 = Wait (ms)(milliseconds to wait=u32 30) -> ()  [unwired: 1 out]
          }
          n1725 = while {
            tunnel: w2420 -> [w2447]
            tunnel: [w2447] -> w2421
            stop <- w2443 stop-if-true
            n1726 = global read "Robot Global Data.vi" "Distance (enc.)"() -> (w2445:dbl)
            n1727 = global write "Robot Global Data.vi" "1-Y"(-0.85 ("1-X")) -> ()
            n1728 = Greater?(x=w2445, y=120.0) -> (0:w2443:bool)
            n1729 = Wait (ms)(milliseconds to wait=u32 20) -> ()  [unwired: 1 out]
          }
          n1730 = while {
            tunnel: [w2440] -> w2416
            tunnel: w2421 -> [w2440]
            stop <- w2434 stop-if-true
            n1731 = global read "Robot Global Data.vi" "Yaw"() -> (w2438:dbl)
            n1732 = global write "Robot Global Data.vi" "Arm Control"(1.0 ("Arm Control")) -> ()
            n1733 = Absolute Value(x=w2438) -> (abs(x)=w2437:dbl)
            n1734 = global write "Robot Global Data.vi" "1-Y"(0.0 ("1-X")) -> ()
            n1735 = Less?(x=w2437, y=30.0) -> (x < y?=w2434:bool)
            n1736 = global write "Robot Global Data.vi" "1-X"(-0.85 ("1-X")) -> ()
            n1737 = Wait (ms)(milliseconds to wait=u32 20) -> ()  [unwired: 1 out]
          }
          n1738 = while {
            tunnel: [w2425] -> w2417
            tunnel: w2416 -> [w2425]
            stop <- FALSE stop-if-true
            w2426 = 0.0 ("1-X")
            n1739 = Wait (ms)(milliseconds to wait=u32 20) -> ()  [unwired: 1 out]
            n1740 = global write "Robot Global Data.vi" "1-X"(w2426) -> ()
            n1741 = global write "Robot Global Data.vi" "1-Y"(w2426) -> ()
          }
        }
      }
    }
    frame 1, Default {
      # "Do not attempt"
      # "Cheval"
      n1742 = while {
        tunnel: w2463 -> [_]
        stop <- FALSE stop-if-true
        n1743 = Wait (ms)(milliseconds to wait=u32 200) -> ()  [unwired: 1 out]
      }
    }
    frame 3 {
      # "Rock"
      # "turn close enough, come back"
      n1744 = global read "Robot Global Data.vi" "Starting Position"() -> (w2468:i32)
      n1745 = Not Equal?(x=w2468, y=2) -> (x != y?=w2467:bool)
      n1746 = case shown="True" w2467 {
        tunnel: w2466 -> [w2471 w2478]
        tunnel: [w2470 w2475] -> _
        frame False {
          n1747 = while {
            tunnel: w2471 -> [w2473]
            tunnel: [w2473] -> w2470
            stop <- FALSE stop-if-true
            n1748 = Wait (ms)(milliseconds to wait=u32 200) -> ()  [unwired: 1 out]
          }
        }
        frame True {
          n1749 = while {
            tunnel: w2478 -> [w2497]
            tunnel: [w2497] -> w2477
            stop <- w2499 stop-if-true
            n1750 = global read "Robot Global Data.vi" "Yaw"() -> (w2496:dbl)
            n1751 = Sign(1:w2496) -> (0:w2495:dbl)
            n1752 = global read "Robot Global Data.vi" "Yaw"() -> (w2502:dbl)
            n1753 = Multiply(x=-0.55, y=w2495) -> (x*y=w2493:dbl)
            n1754 = Absolute Value(x=w2502) -> (abs(x)=w2501:dbl)
            n1755 = global write "Robot Global Data.vi" "1-X"(w2493) -> ()
            n1756 = Less?(x=w2501, y=2.0) -> (x < y?=w2499:bool)
            n1757 = Wait (ms)(milliseconds to wait=u32 20) -> ()  [unwired: 1 out]
          }
          n1758 = while {
            tunnel: w2477 -> [w2491]
            tunnel: [w2491] -> w2476
            stop <- w2487 stop-if-true
            n1759 = global read "Robot Global Data.vi" "Distance (enc.)"() -> (w2489:dbl)
            n1760 = global read "Robot Global Data.vi" "Yaw"() -> (w2482:dbl)
            n1761 = call-poly <vilib>:"PID.vi"("output range"=cluster{"output high":dbl, "output low":dbl} {"output high"=0.8, "output low"=-0.8} ("output range 2"), "PID gains"=T7 {"proportional gain (Kc)"=0.048, "integral time (Ti, min)"=0.01, "derivative time (Td, min)"=0.0} ("PID gains 2"), "process variable"=w2482, "setpoint"=0.0) -> ("output"=w2484:dbl)  [unwired: 6 in, 1 out]
            n1762 = global write "Robot Global Data.vi" "1-Y"(0.85 ("1-X")) -> ()
            n1763 = Less?(x=w2489, y=-115.0) -> (x < y?=w2487:bool)
            n1764 = global write "Robot Global Data.vi" "1-X"(w2484) -> ()
            n1765 = Wait (ms)(milliseconds to wait=u32 20) -> ()  [unwired: 1 out]
          }
          n1766 = while {
            tunnel: w2476 -> [w2481]
            tunnel: [w2481] -> w2475
            stop <- FALSE stop-if-true
            w2479 = 0.0 ("1-X")
            n1767 = global write "Robot Global Data.vi" "1-Y"(w2479) -> ()
            n1768 = global write "Robot Global Data.vi" "1-X"(w2479) -> ()
          }
        }
      }
    }
    frame 4 {
      # "Rough"
      n1769 = global read "Robot Global Data.vi" "Starting Position"() -> (w2505:i32)
      n1770 = Not Equal?(x=w2505, y=2) -> (x != y?=w2504:bool)
      n1771 = case shown="True" w2504 {
        tunnel: w2503 -> [w2508 w2515]
        tunnel: [w2507 w2512] -> _
        frame False {
          n1772 = while {
            tunnel: w2508 -> [w2510]
            tunnel: [w2510] -> w2507
            stop <- FALSE stop-if-true
            n1773 = Wait (ms)(milliseconds to wait=u32 200) -> ()  [unwired: 1 out]
          }
        }
        frame True {
          n1774 = while {
            tunnel: w2515 -> [w2534]
            tunnel: [w2534] -> w2514
            stop <- w2536 stop-if-true
            n1775 = global read "Robot Global Data.vi" "Yaw"() -> (w2533:dbl)
            n1776 = Sign(1:w2533) -> (0:w2532:dbl)
            n1777 = global read "Robot Global Data.vi" "Yaw"() -> (w2539:dbl)
            n1778 = Multiply(x=-0.55, y=w2532) -> (x*y=w2530:dbl)
            n1779 = Absolute Value(x=w2539) -> (abs(x)=w2538:dbl)
            n1780 = global write "Robot Global Data.vi" "1-X"(w2530) -> ()
            n1781 = Less?(x=w2538, y=2.0) -> (x < y?=w2536:bool)
            n1782 = Wait (ms)(milliseconds to wait=u32 20) -> ()  [unwired: 1 out]
          }
          n1783 = while {
            tunnel: w2514 -> [w2528]
            tunnel: [w2528] -> w2513
            stop <- w2524 stop-if-true
            n1784 = global read "Robot Global Data.vi" "Distance (enc.)"() -> (w2526:dbl)
            n1785 = global read "Robot Global Data.vi" "Yaw"() -> (w2519:dbl)
            n1786 = call-poly <vilib>:"PID.vi"("output range"=cluster{"output high":dbl, "output low":dbl} {"output high"=0.8, "output low"=-0.8} ("output range 2"), "PID gains"=T7 {"proportional gain (Kc)"=0.048, "integral time (Ti, min)"=0.01, "derivative time (Td, min)"=0.0} ("PID gains 2"), "process variable"=w2519, "setpoint"=0.0) -> ("output"=w2521:dbl)  [unwired: 6 in, 1 out]
            n1787 = global write "Robot Global Data.vi" "1-Y"(0.85 ("1-X")) -> ()
            n1788 = Less?(x=w2526, y=-100.0) -> (x < y?=w2524:bool)
            n1789 = global write "Robot Global Data.vi" "1-X"(w2521) -> ()
            n1790 = Wait (ms)(milliseconds to wait=u32 20) -> ()  [unwired: 1 out]
          }
          n1791 = while {
            tunnel: w2513 -> [w2518]
            tunnel: [w2518] -> w2512
            stop <- FALSE stop-if-true
            w2516 = 0.0 ("1-X")
            n1792 = global write "Robot Global Data.vi" "1-Y"(w2516) -> ()
            n1793 = global write "Robot Global Data.vi" "1-X"(w2516) -> ()
          }
        }
      }
    }
    frame 5 {
      # "Moat"
      n1794 = global read "Robot Global Data.vi" "Starting Position"() -> (w2542:i32)
      n1795 = Not Equal?(x=w2542, y=2) -> (x != y?=w2541:bool)
      n1796 = case shown="True" w2541 {
        tunnel: w2540 -> [w2545 w2552]
        tunnel: [w2544 w2550] -> _
        frame False {
          n1797 = while {
            tunnel: w2545 -> [w2547]
            tunnel: [w2547] -> w2544
            stop <- FALSE stop-if-true
            n1798 = Wait (ms)(milliseconds to wait=u32 200) -> ()  [unwired: 1 out]
          }
        }
        frame True {
          n1799 = while {
            tunnel: w2552 -> [w2571]
            tunnel: [w2571] -> w2549
            stop <- w2573 stop-if-true
            n1800 = global read "Robot Global Data.vi" "Yaw"() -> (w2570:dbl)
            n1801 = Sign(1:w2570) -> (0:w2569:dbl)
            n1802 = global read "Robot Global Data.vi" "Yaw"() -> (w2576:dbl)
            n1803 = Multiply(x=-0.55, y=w2569) -> (x*y=w2567:dbl)
            n1804 = Absolute Value(x=w2576) -> (abs(x)=w2575:dbl)
            n1805 = global write "Robot Global Data.vi" "1-X"(w2567) -> ()
            n1806 = Less?(x=w2575, y=2.0) -> (x < y?=w2573:bool)
            n1807 = Wait (ms)(milliseconds to wait=u32 20) -> ()  [unwired: 1 out]
          }
          n1808 = while {
            tunnel: w2549 -> [w2565]
            tunnel: [w2565] -> w2551
            stop <- w2561 stop-if-true
            n1809 = global read "Robot Global Data.vi" "Distance (enc.)"() -> (w2563:dbl)
            n1810 = global read "Robot Global Data.vi" "Yaw"() -> (w2556:dbl)
            n1811 = call-poly <vilib>:"PID.vi"("output range"=cluster{"output high":dbl, "output low":dbl} {"output high"=0.8, "output low"=-0.8} ("output range 2"), "PID gains"=T7 {"proportional gain (Kc)"=0.048, "integral time (Ti, min)"=0.01, "derivative time (Td, min)"=0.0} ("PID gains 2"), "process variable"=w2556, "setpoint"=0.0) -> ("output"=w2558:dbl)  [unwired: 6 in, 1 out]
            n1812 = global write "Robot Global Data.vi" "1-Y"(1.0 ("1-X")) -> ()
            n1813 = Less?(x=w2563, y=-124.0) -> (x < y?=w2561:bool)
            n1814 = global write "Robot Global Data.vi" "1-X"(w2558) -> ()
            n1815 = Wait (ms)(milliseconds to wait=u32 20) -> ()  [unwired: 1 out]
          }
          n1816 = while {
            tunnel: w2551 -> [w2555]
            tunnel: [w2555] -> w2550
            stop <- FALSE stop-if-true
            w2553 = 0.0 ("1-X")
            n1817 = global write "Robot Global Data.vi" "1-Y"(w2553) -> ()
            n1818 = global write "Robot Global Data.vi" "1-X"(w2553) -> ()
          }
        }
      }
    }
    frame 6 {
      # "Ramps"
      n1819 = global read "Robot Global Data.vi" "Starting Position"() -> (w2579:i32)
      n1820 = Not Equal?(x=w2579, y=2) -> (x != y?=w2578:bool)
      n1821 = case shown="True" w2578 {
        tunnel: w2577 -> [w2582 w2589]
        tunnel: [w2581 w2586] -> _
        frame False {
          n1822 = while {
            tunnel: w2582 -> [w2584]
            tunnel: [w2584] -> w2581
            stop <- FALSE stop-if-true
            n1823 = Wait (ms)(milliseconds to wait=u32 200) -> ()  [unwired: 1 out]
          }
        }
        frame True {
          n1824 = while {
            tunnel: w2589 -> [w2608]
            tunnel: [w2608] -> w2588
            stop <- w2610 stop-if-true
            n1825 = global read "Robot Global Data.vi" "Yaw"() -> (w2607:dbl)
            n1826 = Sign(1:w2607) -> (0:w2606:dbl)
            n1827 = global read "Robot Global Data.vi" "Yaw"() -> (w2613:dbl)
            n1828 = Multiply(x=-0.55, y=w2606) -> (x*y=w2604:dbl)
            n1829 = Absolute Value(x=w2613) -> (abs(x)=w2612:dbl)
            n1830 = global write "Robot Global Data.vi" "1-X"(w2604) -> ()
            n1831 = Less?(x=w2612, y=2.0) -> (x < y?=w2610:bool)
            n1832 = Wait (ms)(milliseconds to wait=u32 20) -> ()  [unwired: 1 out]
          }
          n1833 = while {
            tunnel: w2588 -> [w2602]
            tunnel: [w2602] -> w2587
            stop <- w2598 stop-if-true
            n1834 = global read "Robot Global Data.vi" "Distance (enc.)"() -> (w2600:dbl)
            n1835 = global read "Robot Global Data.vi" "Yaw"() -> (w2593:dbl)
            n1836 = call-poly <vilib>:"PID.vi"("output range"=cluster{"output high":dbl, "output low":dbl} {"output high"=0.8, "output low"=-0.8} ("output range 2"), "PID gains"=T7 {"proportional gain (Kc)"=0.048, "integral time (Ti, min)"=0.01, "derivative time (Td, min)"=0.0} ("PID gains 2"), "process variable"=w2593, "setpoint"=0.0) -> ("output"=w2595:dbl)  [unwired: 6 in, 1 out]
            n1837 = global write "Robot Global Data.vi" "1-Y"(0.9 ("1-X")) -> ()
            n1838 = Less?(x=w2600, y=-120.0) -> (x < y?=w2598:bool)
            n1839 = global write "Robot Global Data.vi" "1-X"(w2595) -> ()
            n1840 = Wait (ms)(milliseconds to wait=u32 20) -> ()  [unwired: 1 out]
          }
          n1841 = while {
            tunnel: w2587 -> [w2592]
            tunnel: [w2592] -> w2586
            stop <- FALSE stop-if-true
            w2590 = 0.0 ("1-X")
            n1842 = global write "Robot Global Data.vi" "1-Y"(w2590) -> ()
            n1843 = global write "Robot Global Data.vi" "1-X"(w2590) -> ()
          }
        }
      }
    }
  }
